vi "CAN Calibration Database Template.vi"() -> (0 "Calibration Template":string="<?xml version=\"1.0\" encoding=\"UTF-8\"?>\n<fx:FIBEX xmlns:fx=\"http://www.asam.net/xml/fbx\" xmlns:can=\"http://www.asam.net/xml/fbx/can\" xmlns:flexray=\"http://www.asam.net/xml/fbx/flexray\" xmlns:lin=\"http://www.asam.net/xml/fbx/lin\" xmlns:ho=\"http://www.asam.net/xml\" xmlns:ni=\"http://www.ni.com/xnet\" xmlns:xsi=\"http://www.w3.org/2001/XMLSchema-instance\" xsi:schemaLocation=\"http://www.asam.net/xml/fbx/all \\FIBEX311schema\\fibex4multiplatform.xsd\" VERSION=\"3.1.1\">\n  <fx:PROJECT ID=\"NI-XNET\">\n    <ho:SHORT-NAME>XNET1</ho:SHORT-NAME>\n  </fx:PROJECT>\n  <fx:ELEMENTS>\n    <fx:CLUSTERS>\n      <fx:CLUSTER ID=\"cluster1\">\n        <ho:SHORT-NAME>BS1200_Control_Bus</ho:SHORT-NAME>\n        <ho:DESC></ho:DESC>\n        <fx:SPEED>500000</fx:SPEED>\n        <fx:IS-HIGH-LOW-BIT-ORDER>true</fx:IS-HIGH-LOW-BIT-ORDER>\n        <fx:BIT-COUNTING-POLICY>SAWTOOTH</fx:BIT-COUNTING-POLICY>\n        <fx:PROTOCOL xsi:type=\"can:PROTOCOL-TYPE\">CAN</fx:PROTOCOL>\n        <fx:CHANNEL-REFS>\n          <fx:CHANNEL-REF ID-REF=\"channel1\"/>\n        </fx:CHANNEL-REFS>\n        <fx:MEDIUM>ELECTRICAL</fx:MEDIUM>\n      </fx:CLUSTER>\n    </fx:CLUSTERS>\n    <fx:CHANNELS>\n      <fx:CHANNEL ID=\"channel1\">\n        <ho:SHORT-NAME>Channel1</ho:SHORT-NAME>\n        <fx:PDU-TRIGGERINGS>\n        <fx:PDU-TRIGGERING ID=\"pdutrg1\">\n          <fx:TIMINGS>\n            <fx:CYCLIC-TIMING>\n              <fx:REPEATING-TIME-RANGE>\n                <fx:VALUE>PT0.01000000S</fx:VALUE>\n              </fx:REPEATING-TIME-RANGE>\n            </fx:CYCLIC-TIMING>\n          </fx:TIMINGS>\n          <fx:PDU-REF ID-REF=\"pdu1\"/>\n        </fx:PDU-TRIGGERING>\n        <fx:PDU-TRIGGERING ID=\"pdutrg2\">\n          <fx:TIMINGS>\n            <fx:EVENT-CONTROLLED-TIMING>\n              <fx:DEBOUNCE-TIME-RANGE>\n                <fx:VALUE>PT0.10000000S</fx:VALUE>\n              </fx:DEBOUNCE-TIME-RANGE>\n            </fx:EVENT-CONTROLLED-TIMING>\n          </fx:TIMINGS>\n          <fx:PDU-REF ID-REF=\"pdu10\"/>\n        </fx:PDU-TRIGGERING>\n        <fx:PDU-TRIGGERING ID=\"pdutrg3\">\n          <fx:TIMINGS>\n            <fx:EVENT-CONTROLLED-TIMING>\n              <fx:DEBOUNCE-TIME-RANGE>\n                <fx:VALUE>PT0.10000000S</fx:VALUE>\n              </fx:DEBOUNCE-TIME-RANGE>\n            </fx:EVENT-CONTROLLED-TIMING>\n          </fx:TIMINGS>\n          <fx:PDU-REF ID-REF=\"pdu11\"/>\n        </fx:PDU-TRIGGERING>\n        <fx:PDU-TRIGGERING ID=\"pdutrg4\">\n          <fx:TIMINGS>\n            <fx:CYCLIC-TIMING>\n              <fx:REPEATING-TIME-RANGE>\n                <fx:VALUE>PT0.01000000S</fx:VALUE>\n              </fx:REPEATING-TIME-RANGE>\n            </fx:CYCLIC-TIMING>\n          </fx:TIMINGS>\n          <fx:PDU-REF ID-REF=\"pdu12\"/>\n        </fx:PDU-TRIGGERING>\n        <fx:PDU-TRIGGERING ID=\"pdutrg5\">\n          <fx:TIMINGS>\n            <fx:CYCLIC-TIMING>\n              <fx:REPEATING-TIME-RANGE>\n                <fx:VALUE>PT0.01000000S</fx:VALUE>\n              </fx:REPEATING-TIME-RANGE>\n            </fx:CYCLIC-TIMING>\n          </fx:TIMINGS>\n          <fx:PDU-REF ID-REF=\"pdu13\"/>\n        </fx:PDU-TRIGGERING>\n        <fx:PDU-TRIGGERING ID=\"pdutrg6\">\n          <fx:TIMINGS>\n            <fx:CYCLIC-TIMING>\n              <fx:REPEATING-TIME-RANGE>\n                <fx:VALUE>PT0.01000000S</fx:VALUE>\n              </fx:REPEATING-TIME-RANGE>\n            </fx:CYCLIC-TIMING>\n          </fx:TIMINGS>\n          <fx:PDU-REF ID-REF=\"pdu14\"/>\n        </fx:PDU-TRIGGERING>\n        <fx:PDU-TRIGGERING ID=\"pdutrg7\">\n          <fx:TIMINGS>\n            <fx:EVENT-CONTROLLED-TIMING>\n              <fx:DEBOUNCE-TIME-RANGE>\n                <fx:VALUE>PT0.10000000S</fx:VALUE>\n              </fx:DEBOUNCE-TIME-RANGE>\n            </fx:EVENT-CONTROLLED-TIMING>\n          </fx:TIMINGS>\n          <fx:PDU-REF ID-REF=\"pdu15\"/>\n        </fx:PDU-TRIGGERING>\n        <fx:PDU-TRIGGERING ID=\"pdutrg8\">\n          <fx:TIMINGS>\n            <fx:EVENT-CONTROLLED-TIMING>\n              <fx:DEBOUNCE-TIME-RANGE>\n                <fx:VALUE>PT0.10000000S</fx:VALUE>\n              </fx:DEBOUNCE-TIME-RANGE>\n            </fx:EVENT-CONTROLLED-TIMING>\n          </fx:TIMINGS>\n          <fx:PDU-REF ID-REF=\"pdu16\"/>\n        </fx:PDU-TRIGGERING>\n        <fx:PDU-TRIGGERING ID=\"pdutrg9\">\n          <fx:TIMINGS>\n            <fx:EVENT-CONTROLLED-TIMING>\n              <fx:DEBOUNCE-TIME-RANGE>\n                <fx:VALUE>PT0.10000000S</fx:VALUE>\n              </fx:DEBOUNCE-TIME-RANGE>\n            </fx:EVENT-CONTROLLED-TIMING>\n          </fx:TIMINGS>\n          <fx:PDU-REF ID-REF=\"pdu17\"/>\n        </fx:PDU-TRIGGERING>\n        <fx:PDU-TRIGGERING ID=\"pdutrg10\">\n          <fx:TIMINGS>\n            <fx:EVENT-CONTROLLED-TIMING>\n              <fx:DEBOUNCE-TIME-RANGE>\n                <fx:VALUE>PT0.10000000S</fx:VALUE>\n              </fx:DEBOUNCE-TIME-RANGE>\n            </fx:EVENT-CONTROLLED-TIMING>\n          </fx:TIMINGS>\n          <fx:PDU-REF ID-REF=\"pdu18\"/>\n        </fx:PDU-TRIGGERING>\n        <fx:PDU-TRIGGERING ID=\"pdutrg11\">\n          <fx:TIMINGS>\n            <fx:EVENT-CONTROLLED-TIMING>\n              <fx:DEBOUNCE-TIME-RANGE>\n                <fx:VALUE>PT0.10000000S</fx:VALUE>\n              </fx:DEBOUNCE-TIME-RANGE>\n            </fx:EVENT-CONTROLLED-TIMING>\n          </fx:TIMINGS>\n          <fx:PDU-REF ID-REF=\"pdu19\"/>\n        </fx:PDU-TRIGGERING>\n        <fx:PDU-TRIGGERING ID=\"pdutrg12\">\n          <fx:TIMINGS>\n            <fx:CYCLIC-TIMING>\n              <fx:REPEATING-TIME-RANGE>\n                <fx:VALUE>PT0.01000000S</fx:VALUE>\n              </fx:REPEATING-TIME-RANGE>\n            </fx:CYCLIC-TIMING>\n          </fx:TIMINGS>\n          <fx:PDU-REF ID-REF=\"pdu2\"/>\n        </fx:PDU-TRIGGERING>\n        <fx:PDU-TRIGGERING ID=\"pdutrg13\">\n          <fx:TIMINGS>\n            <fx:EVENT-CONTROLLED-TIMING>\n              <fx:DEBOUNCE-TIME-RANGE>\n                <fx:VALUE>PT0.10000000S</fx:VALUE>\n              </fx:DEBOUNCE-TIME-RANGE>\n            </fx:EVENT-CONTROLLED-TIMING>\n          </fx:TIMINGS>\n          <fx:PDU-REF ID-REF=\"pdu20\"/>\n        </fx:PDU-TRIGGERING>\n        <fx:PDU-TRIGGERING ID=\"pdutrg14\">\n          <fx:TIMINGS>\n            <fx:CYCLIC-TIMING>\n              <fx:REPEATING-TIME-RANGE>\n                <fx:VALUE>PT0.01000000S</fx:VALUE>\n              </fx:REPEATING-TIME-RANGE>\n            </fx:CYCLIC-TIMING>\n          </fx:TIMINGS>\n          <fx:PDU-REF ID-REF=\"pdu21\"/>\n        </fx:PDU-TRIGGERING>\n        <fx:PDU-TRIGGERING ID=\"pdutrg15\">\n          <fx:TIMINGS>\n            <fx:EVENT-CONTROLLED-TIMING>\n              <fx:DEBOUNCE-TIME-RANGE>\n                <fx:VALUE>PT0.10000000S</fx:VALUE>\n              </fx:DEBOUNCE-TIME-RANGE>\n            </fx:EVENT-CONTROLLED-TIMING>\n          </fx:TIMINGS>\n          <fx:PDU-REF ID-REF=\"pdu22\"/>\n        </fx:PDU-TRIGGERING>\n        <fx:PDU-TRIGGERING ID=\"pdutrg16\">\n          <fx:TIMINGS>\n            <fx:EVENT-CONTROLLED-TIMING>\n              <fx:DEBOUNCE-TIME-RANGE>\n                <fx:VALUE>PT0.10000000S</fx:VALUE>\n              </fx:DEBOUNCE-TIME-RANGE>\n            </fx:EVENT-CONTROLLED-TIMING>\n          </fx:TIMINGS>\n          <fx:PDU-REF ID-REF=\"pdu23\"/>\n        </fx:PDU-TRIGGERING>\n        <fx:PDU-TRIGGERING ID=\"pdutrg17\">\n          <fx:TIMINGS>\n            <fx:CYCLIC-TIMING>\n              <fx:REPEATING-TIME-RANGE>\n                <fx:VALUE>PT1.000000S</fx:VALUE>\n              </fx:REPEATING-TIME-RANGE>\n            </fx:CYCLIC-TIMING>\n          </fx:TIMINGS>\n          <fx:PDU-REF ID-REF=\"pdu24\"/>\n        </fx:PDU-TRIGGERING>\n        <fx:PDU-TRIGGERING ID=\"pdutrg18\">\n          <fx:TIMINGS>\n            <fx:EVENT-CONTROLLED-TIMING>\n              <fx:DEBOUNCE-TIME-RANGE>\n                <fx:VALUE>PT0.10000000S</fx:VALUE>\n              </fx:DEBOUNCE-TIME-RANGE>\n            </fx:EVENT-CONTROLLED-TIMING>\n          </fx:TIMINGS>\n          <fx:PDU-REF ID-REF=\"pdu3\"/>\n        </fx:PDU-TRIGGERING>\n        <fx:PDU-TRIGGERING ID=\"pdutrg19\">\n          <fx:TIMINGS>\n            <fx:EVENT-CONTROLLED-TIMING>\n              <fx:DEBOUNCE-TIME-RANGE>\n                <fx:VALUE>PT0.10000000S</fx:VALUE>\n              </fx:DEBOUNCE-TIME-RANGE>\n            </fx:EVENT-CONTROLLED-TIMING>\n          </fx:TIMINGS>\n          <fx:PDU-REF ID-REF=\"pdu4\"/>\n        </fx:PDU-TRIGGERING>\n        <fx:PDU-TRIGGERING ID=\"pdutrg20\">\n          <fx:TIMINGS>\n            <fx:EVENT-CONTROLLED-TIMING>\n              <fx:DEBOUNCE-TIME-RANGE>\n                <fx:VALUE>PT0.10000000S</fx:VALUE>\n              </fx:DEBOUNCE-TIME-RANGE>\n            </fx:EVENT-CONTROLLED-TIMING>\n          </fx:TIMINGS>\n          <fx:PDU-REF ID-REF=\"pdu5\"/>\n        </fx:PDU-TRIGGERING>\n        <fx:PDU-TRIGGERING ID=\"pdutrg21\">\n          <fx:TIMINGS>\n            <fx:CYCLIC-TIMING>\n              <fx:REPEATING-TIME-RANGE>\n                <fx:VALUE>PT0.01000000S</fx:VALUE>\n              </fx:REPEATING-TIME-RANGE>\n            </fx:CYCLIC-TIMING>\n          </fx:TIMINGS>\n          <fx:PDU-REF ID-REF=\"pdu6\"/>\n        </fx:PDU-TRIGGERING>\n        <fx:PDU-TRIGGERING ID=\"pdutrg22\">\n          <fx:TIMINGS>\n            <fx:CYCLIC-TIMING>\n              <fx:REPEATING-TIME-RANGE>\n                <fx:VALUE>PT0.01000000S</fx:VALUE>\n              </fx:REPEATING-TIME-RANGE>\n            </fx:CYCLIC-TIMING>\n          </fx:TIMINGS>\n          <fx:PDU-REF ID-REF=\"pdu7\"/>\n        </fx:PDU-TRIGGERING>\n        <fx:PDU-TRIGGERING ID=\"pdutrg23\">\n          <fx:TIMINGS>\n            <fx:CYCLIC-TIMING>\n              <fx:REPEATING-TIME-RANGE>\n                <fx:VALUE>PT0.01000000S</fx:VALUE>\n              </fx:REPEATING-TIME-RANGE>\n            </fx:CYCLIC-TIMING>\n          </fx:TIMINGS>\n          <fx:PDU-REF ID-REF=\"pdu8\"/>\n        </fx:PDU-TRIGGERING>\n        <fx:PDU-TRIGGERING ID=\"pdutrg24\">\n          <fx:TIMINGS>\n            <fx:EVENT-CONTROLLED-TIMING>\n              <fx:DEBOUNCE-TIME-RANGE>\n                <fx:VALUE>PT0.10000000S</fx:VALUE>\n              </fx:DEBOUNCE-TIME-RANGE>\n            </fx:EVENT-CONTROLLED-TIMING>\n          </fx:TIMINGS>\n          <fx:PDU-REF ID-REF=\"pdu9\"/>\n        </fx:PDU-TRIGGERING>\n        </fx:PDU-TRIGGERINGS>\n        <fx:FRAME-TRIGGERINGS>\n          <fx:FRAME-TRIGGERING ID=\"trig1\">\n            <fx:IDENTIFIER>\n              <fx:IDENTIFIER-VALUE>128</fx:IDENTIFIER-VALUE>\n            </fx:IDENTIFIER>\n            <fx:FRAME-REF ID-REF=\"frm1\"/>\n          </fx:FRAME-TRIGGERING>\n          <fx:FRAME-TRIGGERING ID=\"trig2\">\n            <fx:IDENTIFIER>\n              <fx:IDENTIFIER-VALUE>192</fx:IDENTIFIER-VALUE>\n            </fx:IDENTIFIER>\n            <fx:FRAME-REF ID-REF=\"frm2\"/>\n          </fx:FRAME-TRIGGERING>\n          <fx:FRAME-TRIGGERING ID=\"trig3\">\n            <fx:IDENTIFIER>\n              <fx:IDENTIFIER-VALUE>1200</fx:IDENTIFIER-VALUE>\n            </fx:IDENTIFIER>\n            <fx:FRAME-REF ID-REF=\"frm3\"/>\n          </fx:FRAME-TRIGGERING>\n          <fx:FRAME-TRIGGERING ID=\"trig4\">\n            <fx:IDENTIFIER>\n              <fx:IDENTIFIER-VALUE>1280</fx:IDENTIFIER-VALUE>\n            </fx:IDENTIFIER>\n            <fx:FRAME-REF ID-REF=\"frm4\"/>\n          </fx:FRAME-TRIGGERING>\n          <fx:FRAME-TRIGGERING ID=\"trig5\">\n            <fx:IDENTIFIER>\n              <fx:IDENTIFIER-VALUE>512</fx:IDENTIFIER-VALUE>\n            </fx:IDENTIFIER>\n            <fx:FRAME-REF ID-REF=\"frm5\"/>\n          </fx:FRAME-TRIGGERING>\n          <fx:FRAME-TRIGGERING ID=\"trig6\">\n            <fx:IDENTIFIER>\n              <fx:IDENTIFIER-VALUE>544</fx:IDENTIFIER-VALUE>\n            </fx:IDENTIFIER>\n            <fx:FRAME-REF ID-REF=\"frm6\"/>\n          </fx:FRAME-TRIGGERING>\n          <fx:FRAME-TRIGGERING ID=\"trig7\">\n            <fx:IDENTIFIER>\n              <fx:IDENTIFIER-VALUE>1024</fx:IDENTIFIER-VALUE>\n            </fx:IDENTIFIER>\n            <fx:FRAME-REF ID-REF=\"frm7\"/>\n          </fx:FRAME-TRIGGERING>\n          <fx:FRAME-TRIGGERING ID=\"trig8\">\n            <fx:IDENTIFIER>\n              <fx:IDENTIFIER-VALUE>1152</fx:IDENTIFIER-VALUE>\n            </fx:IDENTIFIER>\n            <fx:FRAME-REF ID-REF=\"frm8\"/>\n          </fx:FRAME-TRIGGERING>\n          <fx:FRAME-TRIGGERING ID=\"trig9\">\n            <fx:IDENTIFIER>\n              <fx:IDENTIFIER-VALUE>1184</fx:IDENTIFIER-VALUE>\n            </fx:IDENTIFIER>\n            <fx:FRAME-REF ID-REF=\"frm9\"/>\n          </fx:FRAME-TRIGGERING>\n          <fx:FRAME-TRIGGERING ID=\"trig10\">\n            <fx:IDENTIFIER>\n              <fx:IDENTIFIER-VALUE>1296</fx:IDENTIFIER-VALUE>\n            </fx:IDENTIFIER>\n            <fx:FRAME-REF ID-REF=\"frm10\"/>\n          </fx:FRAME-TRIGGERING>\n          <fx:FRAME-TRIGGERING ID=\"trig11\">\n            <fx:IDENTIFIER>\n              <fx:IDENTIFIER-VALUE>320</fx:IDENTIFIER-VALUE>\n            </fx:IDENTIFIER>\n            <fx:FRAME-REF ID-REF=\"frm11\"/>\n          </fx:FRAME-TRIGGERING>\n          <fx:FRAME-TRIGGERING ID=\"trig12\">\n            <fx:IDENTIFIER>\n              <fx:IDENTIFIER-VALUE>384</fx:IDENTIFIER-VALUE>\n            </fx:IDENTIFIER>\n            <fx:FRAME-REF ID-REF=\"frm12\"/>\n          </fx:FRAME-TRIGGERING>\n          <fx:FRAME-TRIGGERING ID=\"trig13\">\n            <fx:IDENTIFIER>\n              <fx:IDENTIFIER-VALUE>1344</fx:IDENTIFIER-VALUE>\n            </fx:IDENTIFIER>\n            <fx:FRAME-REF ID-REF=\"frm13\"/>\n          </fx:FRAME-TRIGGERING>\n          <fx:FRAME-TRIGGERING ID=\"trig14\">\n            <fx:IDENTIFIER>\n              <fx:IDENTIFIER-VALUE>1360</fx:IDENTIFIER-VALUE>\n            </fx:IDENTIFIER>\n            <fx:FRAME-REF ID-REF=\"frm14\"/>\n          </fx:FRAME-TRIGGERING>\n          <fx:FRAME-TRIGGERING ID=\"trig15\">\n            <fx:IDENTIFIER>\n              <fx:IDENTIFIER-VALUE>256</fx:IDENTIFIER-VALUE>\n            </fx:IDENTIFIER>\n            <fx:FRAME-REF ID-REF=\"frm15\"/>\n            <fx:MANUFACTURER-EXTENSION>\n              <ni:NI-XNET-EXTENSION>\n                <ni:CAN-FD-MODE>0</ni:CAN-FD-MODE>\n              </ni:NI-XNET-EXTENSION>\n            </fx:MANUFACTURER-EXTENSION>\n          </fx:FRAME-TRIGGERING>\n          <fx:FRAME-TRIGGERING ID=\"trig16\">\n            <fx:IDENTIFIER>\n              <fx:IDENTIFIER-VALUE>288</fx:IDENTIFIER-VALUE>\n            </fx:IDENTIFIER>\n            <fx:FRAME-REF ID-REF=\"frm16\"/>\n          </fx:FRAME-TRIGGERING>\n          <fx:FRAME-TRIGGERING ID=\"trig17\">\n            <fx:IDENTIFIER>\n              <fx:IDENTIFIER-VALUE>304</fx:IDENTIFIER-VALUE>\n            </fx:IDENTIFIER>\n            <fx:FRAME-REF ID-REF=\"frm17\"/>\n          </fx:FRAME-TRIGGERING>\n          <fx:FRAME-TRIGGERING ID=\"trig18\">\n            <fx:IDENTIFIER>\n              <fx:IDENTIFIER-VALUE>160</fx:IDENTIFIER-VALUE>\n            </fx:IDENTIFIER>\n            <fx:FRAME-REF ID-REF=\"frm18\"/>\n          </fx:FRAME-TRIGGERING>\n          <fx:FRAME-TRIGGERING ID=\"trig19\">\n            <fx:IDENTIFIER>\n              <fx:IDENTIFIER-VALUE>176</fx:IDENTIFIER-VALUE>\n            </fx:IDENTIFIER>\n            <fx:FRAME-REF ID-REF=\"frm19\"/>\n          </fx:FRAME-TRIGGERING>\n          <fx:FRAME-TRIGGERING ID=\"trig20\">\n            <fx:IDENTIFIER>\n              <fx:IDENTIFIER-VALUE>400</fx:IDENTIFIER-VALUE>\n            </fx:IDENTIFIER>\n            <fx:FRAME-REF ID-REF=\"frm20\"/>\n          </fx:FRAME-TRIGGERING>\n          <fx:FRAME-TRIGGERING ID=\"trig21\">\n            <fx:IDENTIFIER>\n              <fx:IDENTIFIER-VALUE>416</fx:IDENTIFIER-VALUE>\n            </fx:IDENTIFIER>\n            <fx:FRAME-REF ID-REF=\"frm21\"/>\n          </fx:FRAME-TRIGGERING>\n          <fx:FRAME-TRIGGERING ID=\"trig22\">\n            <fx:IDENTIFIER>\n              <fx:IDENTIFIER-VALUE>640</fx:IDENTIFIER-VALUE>\n            </fx:IDENTIFIER>\n            <fx:FRAME-REF ID-REF=\"frm22\"/>\n            <fx:MANUFACTURER-EXTENSION>\n              <ni:NI-XNET-EXTENSION>\n                <ni:CAN-FD-MODE>0</ni:CAN-FD-MODE>\n              </ni:NI-XNET-EXTENSION>\n            </fx:MANUFACTURER-EXTENSION>\n          </fx:FRAME-TRIGGERING>\n          <fx:FRAME-TRIGGERING ID=\"trig23\">\n            <fx:IDENTIFIER>\n              <fx:IDENTIFIER-VALUE>672</fx:IDENTIFIER-VALUE>\n            </fx:IDENTIFIER>\n            <fx:FRAME-REF ID-REF=\"frm23\"/>\n          </fx:FRAME-TRIGGERING>\n          <fx:FRAME-TRIGGERING ID=\"trig24\">\n            <fx:IDENTIFIER>\n              <fx:IDENTIFIER-VALUE>688</fx:IDENTIFIER-VALUE>\n            </fx:IDENTIFIER>\n            <fx:FRAME-REF ID-REF=\"frm24\"/>\n          </fx:FRAME-TRIGGERING>\n        </fx:FRAME-TRIGGERINGS>\n      </fx:CHANNEL>\n    </fx:CHANNELS>\n    <fx:PDUS>\n      <fx:PDU ID=\"pdu1\">\n        <ho:SHORT-NAME>AI_Readback_1_4_pdu</ho:SHORT-NAME>\n        <ho:DESC></ho:DESC>\n        <fx:BYTE-LENGTH>8</fx:BYTE-LENGTH>\n        <fx:PDU-TYPE>APPLICATION</fx:PDU-TYPE>\n        <fx:SIGNAL-INSTANCES>\n          <fx:SIGNAL-INSTANCE ID=\"sgi1\">\n            <fx:BIT-POSITION>0</fx:BIT-POSITION>\n            <fx:IS-HIGH-LOW-BYTE-ORDER>false</fx:IS-HIGH-LOW-BYTE-ORDER>\n            <fx:SIGNAL-REF ID-REF=\"sig68\"/>\n          </fx:SIGNAL-INSTANCE>\n          <fx:SIGNAL-INSTANCE ID=\"sgi2\">\n            <fx:BIT-POSITION>16</fx:BIT-POSITION>\n            <fx:IS-HIGH-LOW-BYTE-ORDER>false</fx:IS-HIGH-LOW-BYTE-ORDER>\n            <fx:SIGNAL-REF ID-REF=\"sig69\"/>\n          </fx:SIGNAL-INSTANCE>\n          <fx:SIGNAL-INSTANCE ID=\"sgi3\">\n            <fx:BIT-POSITION>32</fx:BIT-POSITION>\n            <fx:IS-HIGH-LOW-BYTE-ORDER>false</fx:IS-HIGH-LOW-BYTE-ORDER>\n            <fx:SIGNAL-REF ID-REF=\"sig70\"/>\n          </fx:SIGNAL-INSTANCE>\n          <fx:SIGNAL-INSTANCE ID=\"sgi4\">\n            <fx:BIT-POSITION>48</fx:BIT-POSITION>\n            <fx:IS-HIGH-LOW-BYTE-ORDER>false</fx:IS-HIGH-LOW-BYTE-ORDER>\n            <fx:SIGNAL-REF ID-REF=\"sig71\"/>\n          </fx:SIGNAL-INSTANCE>\n        </fx:SIGNAL-INSTANCES>\n      </fx:PDU>\n      <fx:PDU ID=\"pdu2\">\n        <ho:SHORT-NAME>AI_Readback_5_8_pdu</ho:SHORT-NAME>\n        <ho:DESC></ho:DESC>\n        <fx:BYTE-LENGTH>8</fx:BYTE-LENGTH>\n        <fx:PDU-TYPE>APPLICATION</fx:PDU-TYPE>\n        <fx:SIGNAL-INSTANCES>\n          <fx:SIGNAL-INSTANCE ID=\"sgi5\">\n            <fx:BIT-POSITION>0</fx:BIT-POSITION>\n            <fx:IS-HIGH-LOW-BYTE-ORDER>false</fx:IS-HIGH-LOW-BYTE-ORDER>\n            <fx:SIGNAL-REF ID-REF=\"sig72\"/>\n          </fx:SIGNAL-INSTANCE>\n          <fx:SIGNAL-INSTANCE ID=\"sgi6\">\n            <fx:BIT-POSITION>16</fx:BIT-POSITION>\n            <fx:IS-HIGH-LOW-BYTE-ORDER>false</fx:IS-HIGH-LOW-BYTE-ORDER>\n            <fx:SIGNAL-REF ID-REF=\"sig73\"/>\n          </fx:SIGNAL-INSTANCE>\n          <fx:SIGNAL-INSTANCE ID=\"sgi7\">\n            <fx:BIT-POSITION>32</fx:BIT-POSITION>\n            <fx:IS-HIGH-LOW-BYTE-ORDER>false</fx:IS-HIGH-LOW-BYTE-ORDER>\n            <fx:SIGNAL-REF ID-REF=\"sig74\"/>\n          </fx:SIGNAL-INSTANCE>\n          <fx:SIGNAL-INSTANCE ID=\"sgi8\">\n            <fx:BIT-POSITION>48</fx:BIT-POSITION>\n            <fx:IS-HIGH-LOW-BYTE-ORDER>false</fx:IS-HIGH-LOW-BYTE-ORDER>\n            <fx:SIGNAL-REF ID-REF=\"sig75\"/>\n          </fx:SIGNAL-INSTANCE>\n        </fx:SIGNAL-INSTANCES>\n      </fx:PDU>\n      <fx:PDU ID=\"pdu3\">\n        <ho:SHORT-NAME>Analog_Out_Set_1_2_pdu</ho:SHORT-NAME>\n        <ho:DESC></ho:DESC>\n        <fx:BYTE-LENGTH>8</fx:BYTE-LENGTH>\n        <fx:PDU-TYPE>APPLICATION</fx:PDU-TYPE>\n        <fx:SIGNAL-INSTANCES>\n          <fx:SIGNAL-INSTANCE ID=\"sgi9\">\n            <fx:BIT-POSITION>0</fx:BIT-POSITION>\n            <fx:IS-HIGH-LOW-BYTE-ORDER>false</fx:IS-HIGH-LOW-BYTE-ORDER>\n            <fx:SIGNAL-REF ID-REF=\"sig11\"/>\n          </fx:SIGNAL-INSTANCE>\n          <fx:SIGNAL-INSTANCE ID=\"sgi10\">\n            <fx:BIT-POSITION>16</fx:BIT-POSITION>\n            <fx:IS-HIGH-LOW-BYTE-ORDER>false</fx:IS-HIGH-LOW-BYTE-ORDER>\n            <fx:SIGNAL-REF ID-REF=\"sig12\"/>\n          </fx:SIGNAL-INSTANCE>\n        </fx:SIGNAL-INSTANCES>\n      </fx:PDU>\n      <fx:PDU ID=\"pdu4\">\n        <ho:SHORT-NAME>Cell_Enable_All_pdu</ho:SHORT-NAME>\n        <ho:DESC></ho:DESC>\n        <fx:BYTE-LENGTH>1</fx:BYTE-LENGTH>\n        <fx:PDU-TYPE>APPLICATION</fx:PDU-TYPE>\n        <fx:SIGNAL-INSTANCES>\n          <fx:SIGNAL-INSTANCE ID=\"sgi11\">\n            <fx:BIT-POSITION>0</fx:BIT-POSITION>\n            <fx:IS-HIGH-LOW-BYTE-ORDER>false</fx:IS-HIGH-LOW-BYTE-ORDER>\n            <fx:SIGNAL-REF ID-REF=\"sig33\"/>\n          </fx:SIGNAL-INSTANCE>\n        </fx:SIGNAL-INSTANCES>\n      </fx:PDU>\n      <fx:PDU ID=\"pdu5\">\n        <ho:SHORT-NAME>Cell_Enable_pdu</ho:SHORT-NAME>\n        <ho:DESC></ho:DESC>\n        <fx:BYTE-LENGTH>2</fx:BYTE-LENGTH>\n        <fx:PDU-TYPE>APPLICATION</fx:PDU-TYPE>\n        <fx:SIGNAL-INSTANCES>\n          <fx:SIGNAL-INSTANCE ID=\"sgi12\">\n            <fx:BIT-POSITION>0</fx:BIT-POSITION>\n            <fx:IS-HIGH-LOW-BYTE-ORDER>false</fx:IS-HIGH-LOW-BYTE-ORDER>\n            <fx:SIGNAL-REF ID-REF=\"sig34\"/>\n          </fx:SIGNAL-INSTANCE>\n          <fx:SIGNAL-INSTANCE ID=\"sgi13\">\n            <fx:BIT-POSITION>8</fx:BIT-POSITION>\n            <fx:IS-HIGH-LOW-BYTE-ORDER>false</fx:IS-HIGH-LOW-BYTE-ORDER>\n            <fx:SIGNAL-REF ID-REF=\"sig35\"/>\n          </fx:SIGNAL-INSTANCE>\n        </fx:SIGNAL-INSTANCES>\n      </fx:PDU>\n      <fx:PDU ID=\"pdu6\">\n        <ho:SHORT-NAME>Cell_I_Readback_1_4_pdu</ho:SHORT-NAME>\n        <ho:DESC></ho:DESC>\n        <fx:BYTE-LENGTH>8</fx:BYTE-LENGTH>\n        <fx:PDU-TYPE>APPLICATION</fx:PDU-TYPE>\n        <fx:SIGNAL-INSTANCES>\n          <fx:SIGNAL-INSTANCE ID=\"sgi14\">\n            <fx:BIT-POSITION>0</fx:BIT-POSITION>\n            <fx:IS-HIGH-LOW-BYTE-ORDER>false</fx:IS-HIGH-LOW-BYTE-ORDER>\n            <fx:SIGNAL-REF ID-REF=\"sig29\"/>\n          </fx:SIGNAL-INSTANCE>\n          <fx:SIGNAL-INSTANCE ID=\"sgi15\">\n            <fx:BIT-POSITION>16</fx:BIT-POSITION>\n            <fx:IS-HIGH-LOW-BYTE-ORDER>false</fx:IS-HIGH-LOW-BYTE-ORDER>\n            <fx:SIGNAL-REF ID-REF=\"sig30\"/>\n          </fx:SIGNAL-INSTANCE>\n          <fx:SIGNAL-INSTANCE ID=\"sgi16\">\n            <fx:BIT-POSITION>32</fx:BIT-POSITION>\n            <fx:IS-HIGH-LOW-BYTE-ORDER>false</fx:IS-HIGH-LOW-BYTE-ORDER>\n            <fx:SIGNAL-REF ID-REF=\"sig31\"/>\n          </fx:SIGNAL-INSTANCE>\n          <fx:SIGNAL-INSTANCE ID=\"sgi17\">\n            <fx:BIT-POSITION>48</fx:BIT-POSITION>\n            <fx:IS-HIGH-LOW-BYTE-ORDER>false</fx:IS-HIGH-LOW-BYTE-ORDER>\n            <fx:SIGNAL-REF ID-REF=\"sig32\"/>\n          </fx:SIGNAL-INSTANCE>\n        </fx:SIGNAL-INSTANCES>\n      </fx:PDU>\n      <fx:PDU ID=\"pdu7\">\n        <ho:SHORT-NAME>Cell_I_Readback_5_8_pdu</ho:SHORT-NAME>\n        <ho:DESC></ho:DESC>\n        <fx:BYTE-LENGTH>8</fx:BYTE-LENGTH>\n        <fx:PDU-TYPE>APPLICATION</fx:PDU-TYPE>\n        <fx:SIGNAL-INSTANCES>\n          <fx:SIGNAL-INSTANCE ID=\"sgi18\">\n            <fx:BIT-POSITION>0</fx:BIT-POSITION>\n            <fx:IS-HIGH-LOW-BYTE-ORDER>false</fx:IS-HIGH-LOW-BYTE-ORDER>\n            <fx:SIGNAL-REF ID-REF=\"sig59\"/>\n          </fx:SIGNAL-INSTANCE>\n          <fx:SIGNAL-INSTANCE ID=\"sgi19\">\n            <fx:BIT-POSITION>16</fx:BIT-POSITION>\n            <fx:IS-HIGH-LOW-BYTE-ORDER>false</fx:IS-HIGH-LOW-BYTE-ORDER>\n            <fx:SIGNAL-REF ID-REF=\"sig60\"/>\n          </fx:SIGNAL-INSTANCE>\n          <fx:SIGNAL-INSTANCE ID=\"sgi20\">\n            <fx:BIT-POSITION>32</fx:BIT-POSITION>\n            <fx:IS-HIGH-LOW-BYTE-ORDER>false</fx:IS-HIGH-LOW-BYTE-ORDER>\n            <fx:SIGNAL-REF ID-REF=\"sig61\"/>\n          </fx:SIGNAL-INSTANCE>\n          <fx:SIGNAL-INSTANCE ID=\"sgi21\">\n            <fx:BIT-POSITION>48</fx:BIT-POSITION>\n            <fx:IS-HIGH-LOW-BYTE-ORDER>false</fx:IS-HIGH-LOW-BYTE-ORDER>\n            <fx:SIGNAL-REF ID-REF=\"sig62\"/>\n          </fx:SIGNAL-INSTANCE>\n        </fx:SIGNAL-INSTANCES>\n      </fx:PDU>\n      <fx:PDU ID=\"pdu8\">\n        <ho:SHORT-NAME>Cell_I_Readback_9_12_pdu</ho:SHORT-NAME>\n        <ho:DESC></ho:DESC>\n        <fx:BYTE-LENGTH>8</fx:BYTE-LENGTH>\n        <fx:PDU-TYPE>APPLICATION</fx:PDU-TYPE>\n        <fx:SIGNAL-INSTANCES>\n          <fx:SIGNAL-INSTANCE ID=\"sgi22\">\n            <fx:BIT-POSITION>0</fx:BIT-POSITION>\n            <fx:IS-HIGH-LOW-BYTE-ORDER>false</fx:IS-HIGH-LOW-BYTE-ORDER>\n            <fx:SIGNAL-REF ID-REF=\"sig63\"/>\n          </fx:SIGNAL-INSTANCE>\n          <fx:SIGNAL-INSTANCE ID=\"sgi23\">\n            <fx:BIT-POSITION>16</fx:BIT-POSITION>\n            <fx:IS-HIGH-LOW-BYTE-ORDER>false</fx:IS-HIGH-LOW-BYTE-ORDER>\n            <fx:SIGNAL-REF ID-REF=\"sig64\"/>\n          </fx:SIGNAL-INSTANCE>\n          <fx:SIGNAL-INSTANCE ID=\"sgi24\">\n            <fx:BIT-POSITION>32</fx:BIT-POSITION>\n            <fx:IS-HIGH-LOW-BYTE-ORDER>false</fx:IS-HIGH-LOW-BYTE-ORDER>\n            <fx:SIGNAL-REF ID-REF=\"sig65\"/>\n          </fx:SIGNAL-INSTANCE>\n          <fx:SIGNAL-INSTANCE ID=\"sgi25\">\n            <fx:BIT-POSITION>48</fx:BIT-POSITION>\n            <fx:IS-HIGH-LOW-BYTE-ORDER>false</fx:IS-HIGH-LOW-BYTE-ORDER>\n            <fx:SIGNAL-REF ID-REF=\"sig66\"/>\n          </fx:SIGNAL-INSTANCE>\n        </fx:SIGNAL-INSTANCES>\n      </fx:PDU>\n      <fx:PDU ID=\"pdu9\">\n        <ho:SHORT-NAME>Cell_I_Set_All_pdu</ho:SHORT-NAME>\n        <ho:DESC></ho:DESC>\n        <fx:BYTE-LENGTH>4</fx:BYTE-LENGTH>\n        <fx:PDU-TYPE>APPLICATION</fx:PDU-TYPE>\n        <fx:SIGNAL-INSTANCES>\n          <fx:SIGNAL-INSTANCE ID=\"sgi26\">\n            <fx:BIT-POSITION>0</fx:BIT-POSITION>\n            <fx:IS-HIGH-LOW-BYTE-ORDER>false</fx:IS-HIGH-LOW-BYTE-ORDER>\n            <fx:SIGNAL-REF ID-REF=\"sig19\"/>\n          </fx:SIGNAL-INSTANCE>\n          <fx:SIGNAL-INSTANCE ID=\"sgi27\">\n            <fx:BIT-POSITION>16</fx:BIT-POSITION>\n            <fx:IS-HIGH-LOW-BYTE-ORDER>false</fx:IS-HIGH-LOW-BYTE-ORDER>\n            <fx:SIGNAL-REF ID-REF=\"sig20\"/>\n          </fx:SIGNAL-INSTANCE>\n        </fx:SIGNAL-INSTANCES>\n      </fx:PDU>\n      <fx:PDU ID=\"pdu10\">\n        <ho:SHORT-NAME>Cell_I_Sink_Set_pdu</ho:SHORT-NAME>\n        <ho:DESC></ho:DESC>\n        <fx:BYTE-LENGTH>3</fx:BYTE-LENGTH>\n        <fx:PDU-TYPE>APPLICATION</fx:PDU-TYPE>\n        <fx:SIGNAL-INSTANCES>\n          <fx:SIGNAL-INSTANCE ID=\"sgi28\">\n            <fx:BIT-POSITION>0</fx:BIT-POSITION>\n            <fx:IS-HIGH-LOW-BYTE-ORDER>false</fx:IS-HIGH-LOW-BYTE-ORDER>\n            <fx:SIGNAL-REF ID-REF=\"sig21\"/>\n          </fx:SIGNAL-INSTANCE>\n          <fx:SIGNAL-INSTANCE ID=\"sgi29\">\n            <fx:BIT-POSITION>8</fx:BIT-POSITION>\n            <fx:IS-HIGH-LOW-BYTE-ORDER>false</fx:IS-HIGH-LOW-BYTE-ORDER>\n            <fx:SIGNAL-REF ID-REF=\"sig22\"/>\n          </fx:SIGNAL-INSTANCE>\n        </fx:SIGNAL-INSTANCES>\n      </fx:PDU>\n      <fx:PDU ID=\"pdu11\">\n        <ho:SHORT-NAME>Cell_I_Source_Set_pdu</ho:SHORT-NAME>\n        <ho:DESC></ho:DESC>\n        <fx:BYTE-LENGTH>3</fx:BYTE-LENGTH>\n        <fx:PDU-TYPE>APPLICATION</fx:PDU-TYPE>\n        <fx:SIGNAL-INSTANCES>\n          <fx:SIGNAL-INSTANCE ID=\"sgi30\">\n            <fx:BIT-POSITION>0</fx:BIT-POSITION>\n            <fx:IS-HIGH-LOW-BYTE-ORDER>false</fx:IS-HIGH-LOW-BYTE-ORDER>\n            <fx:SIGNAL-REF ID-REF=\"sig6\"/>\n          </fx:SIGNAL-INSTANCE>\n          <fx:SIGNAL-INSTANCE ID=\"sgi31\">\n            <fx:BIT-POSITION>8</fx:BIT-POSITION>\n            <fx:IS-HIGH-LOW-BYTE-ORDER>false</fx:IS-HIGH-LOW-BYTE-ORDER>\n            <fx:SIGNAL-REF ID-REF=\"sig7\"/>\n          </fx:SIGNAL-INSTANCE>\n        </fx:SIGNAL-INSTANCES>\n      </fx:PDU>\n      <fx:PDU ID=\"pdu12\">\n        <ho:SHORT-NAME>Cell_V_Readback_1_4_pdu</ho:SHORT-NAME>\n        <ho:DESC></ho:DESC>\n        <fx:BYTE-LENGTH>8</fx:BYTE-LENGTH>\n        <fx:PDU-TYPE>APPLICATION</fx:PDU-TYPE>\n        <fx:SIGNAL-INSTANCES>\n          <fx:SIGNAL-INSTANCE ID=\"sgi32\">\n            <fx:BIT-POSITION>0</fx:BIT-POSITION>\n            <fx:IS-HIGH-LOW-BYTE-ORDER>false</fx:IS-HIGH-LOW-BYTE-ORDER>\n            <fx:SIGNAL-REF ID-REF=\"sig43\"/>\n          </fx:SIGNAL-INSTANCE>\n          <fx:SIGNAL-INSTANCE ID=\"sgi33\">\n            <fx:BIT-POSITION>16</fx:BIT-POSITION>\n            <fx:IS-HIGH-LOW-BYTE-ORDER>false</fx:IS-HIGH-LOW-BYTE-ORDER>\n            <fx:SIGNAL-REF ID-REF=\"sig44\"/>\n          </fx:SIGNAL-INSTANCE>\n          <fx:SIGNAL-INSTANCE ID=\"sgi34\">\n            <fx:BIT-POSITION>32</fx:BIT-POSITION>\n            <fx:IS-HIGH-LOW-BYTE-ORDER>false</fx:IS-HIGH-LOW-BYTE-ORDER>\n            <fx:SIGNAL-REF ID-REF=\"sig45\"/>\n          </fx:SIGNAL-INSTANCE>\n          <fx:SIGNAL-INSTANCE ID=\"sgi35\">\n            <fx:BIT-POSITION>48</fx:BIT-POSITION>\n            <fx:IS-HIGH-LOW-BYTE-ORDER>false</fx:IS-HIGH-LOW-BYTE-ORDER>\n            <fx:SIGNAL-REF ID-REF=\"sig46\"/>\n          </fx:SIGNAL-INSTANCE>\n        </fx:SIGNAL-INSTANCES>\n      </fx:PDU>\n      <fx:PDU ID=\"pdu13\">\n        <ho:SHORT-NAME>Cell_V_Readback_5_8_pdu</ho:SHORT-NAME>\n        <ho:DESC></ho:DESC>\n        <fx:BYTE-LENGTH>8</fx:BYTE-LENGTH>\n        <fx:PDU-TYPE>APPLICATION</fx:PDU-TYPE>\n        <fx:SIGNAL-INSTANCES>\n          <fx:SIGNAL-INSTANCE ID=\"sgi36\">\n            <fx:BIT-POSITION>0</fx:BIT-POSITION>\n            <fx:IS-HIGH-LOW-BYTE-ORDER>false</fx:IS-HIGH-LOW-BYTE-ORDER>\n            <fx:SIGNAL-REF ID-REF=\"sig47\"/>\n          </fx:SIGNAL-INSTANCE>\n          <fx:SIGNAL-INSTANCE ID=\"sgi37\">\n            <fx:BIT-POSITION>16</fx:BIT-POSITION>\n            <fx:IS-HIGH-LOW-BYTE-ORDER>false</fx:IS-HIGH-LOW-BYTE-ORDER>\n            <fx:SIGNAL-REF ID-REF=\"sig48\"/>\n          </fx:SIGNAL-INSTANCE>\n          <fx:SIGNAL-INSTANCE ID=\"sgi38\">\n            <fx:BIT-POSITION>32</fx:BIT-POSITION>\n            <fx:IS-HIGH-LOW-BYTE-ORDER>false</fx:IS-HIGH-LOW-BYTE-ORDER>\n            <fx:SIGNAL-REF ID-REF=\"sig49\"/>\n          </fx:SIGNAL-INSTANCE>\n          <fx:SIGNAL-INSTANCE ID=\"sgi39\">\n            <fx:BIT-POSITION>48</fx:BIT-POSITION>\n            <fx:IS-HIGH-LOW-BYTE-ORDER>false</fx:IS-HIGH-LOW-BYTE-ORDER>\n            <fx:SIGNAL-REF ID-REF=\"sig50\"/>\n          </fx:SIGNAL-INSTANCE>\n        </fx:SIGNAL-INSTANCES>\n      </fx:PDU>\n      <fx:PDU ID=\"pdu14\">\n        <ho:SHORT-NAME>Cell_V_Readback_9_12_pdu</ho:SHORT-NAME>\n        <ho:DESC></ho:DESC>\n        <fx:BYTE-LENGTH>8</fx:BYTE-LENGTH>\n        <fx:PDU-TYPE>APPLICATION</fx:PDU-TYPE>\n        <fx:SIGNAL-INSTANCES>\n          <fx:SIGNAL-INSTANCE ID=\"sgi40\">\n            <fx:BIT-POSITION>0</fx:BIT-POSITION>\n            <fx:IS-HIGH-LOW-BYTE-ORDER>false</fx:IS-HIGH-LOW-BYTE-ORDER>\n            <fx:SIGNAL-REF ID-REF=\"sig25\"/>\n          </fx:SIGNAL-INSTANCE>\n          <fx:SIGNAL-INSTANCE ID=\"sgi41\">\n            <fx:BIT-POSITION>16</fx:BIT-POSITION>\n            <fx:IS-HIGH-LOW-BYTE-ORDER>false</fx:IS-HIGH-LOW-BYTE-ORDER>\n            <fx:SIGNAL-REF ID-REF=\"sig26\"/>\n          </fx:SIGNAL-INSTANCE>\n          <fx:SIGNAL-INSTANCE ID=\"sgi42\">\n            <fx:BIT-POSITION>32</fx:BIT-POSITION>\n            <fx:IS-HIGH-LOW-BYTE-ORDER>false</fx:IS-HIGH-LOW-BYTE-ORDER>\n            <fx:SIGNAL-REF ID-REF=\"sig27\"/>\n          </fx:SIGNAL-INSTANCE>\n          <fx:SIGNAL-INSTANCE ID=\"sgi43\">\n            <fx:BIT-POSITION>48</fx:BIT-POSITION>\n            <fx:IS-HIGH-LOW-BYTE-ORDER>false</fx:IS-HIGH-LOW-BYTE-ORDER>\n            <fx:SIGNAL-REF ID-REF=\"sig28\"/>\n          </fx:SIGNAL-INSTANCE>\n        </fx:SIGNAL-INSTANCES>\n      </fx:PDU>\n      <fx:PDU ID=\"pdu15\">\n        <ho:SHORT-NAME>Cell_V_Set_1_4_pdu</ho:SHORT-NAME>\n        <ho:DESC></ho:DESC>\n        <fx:BYTE-LENGTH>8</fx:BYTE-LENGTH>\n        <fx:PDU-TYPE>APPLICATION</fx:PDU-TYPE>\n        <fx:SIGNAL-INSTANCES>\n          <fx:SIGNAL-INSTANCE ID=\"sgi44\">\n            <fx:BIT-POSITION>0</fx:BIT-POSITION>\n            <fx:IS-HIGH-LOW-BYTE-ORDER>false</fx:IS-HIGH-LOW-BYTE-ORDER>\n            <fx:SIGNAL-REF ID-REF=\"sig51\"/>\n          </fx:SIGNAL-INSTANCE>\n          <fx:SIGNAL-INSTANCE ID=\"sgi45\">\n            <fx:BIT-POSITION>16</fx:BIT-POSITION>\n            <fx:IS-HIGH-LOW-BYTE-ORDER>false</fx:IS-HIGH-LOW-BYTE-ORDER>\n            <fx:SIGNAL-REF ID-REF=\"sig52\"/>\n          </fx:SIGNAL-INSTANCE>\n          <fx:SIGNAL-INSTANCE ID=\"sgi46\">\n            <fx:BIT-POSITION>32</fx:BIT-POSITION>\n            <fx:IS-HIGH-LOW-BYTE-ORDER>false</fx:IS-HIGH-LOW-BYTE-ORDER>\n            <fx:SIGNAL-REF ID-REF=\"sig53\"/>\n          </fx:SIGNAL-INSTANCE>\n          <fx:SIGNAL-INSTANCE ID=\"sgi47\">\n            <fx:BIT-POSITION>48</fx:BIT-POSITION>\n            <fx:IS-HIGH-LOW-BYTE-ORDER>false</fx:IS-HIGH-LOW-BYTE-ORDER>\n            <fx:SIGNAL-REF ID-REF=\"sig54\"/>\n          </fx:SIGNAL-INSTANCE>\n        </fx:SIGNAL-INSTANCES>\n      </fx:PDU>\n      <fx:PDU ID=\"pdu16\">\n        <ho:SHORT-NAME>Cell_V_Set_5_8_pdu</ho:SHORT-NAME>\n        <ho:DESC></ho:DESC>\n        <fx:BYTE-LENGTH>8</fx:BYTE-LENGTH>\n        <fx:PDU-TYPE>APPLICATION</fx:PDU-TYPE>\n        <fx:SIGNAL-INSTANCES>\n          <fx:SIGNAL-INSTANCE ID=\"sgi48\">\n            <fx:BIT-POSITION>0</fx:BIT-POSITION>\n            <fx:IS-HIGH-LOW-BYTE-ORDER>false</fx:IS-HIGH-LOW-BYTE-ORDER>\n            <fx:SIGNAL-REF ID-REF=\"sig55\"/>\n          </fx:SIGNAL-INSTANCE>\n          <fx:SIGNAL-INSTANCE ID=\"sgi49\">\n            <fx:BIT-POSITION>16</fx:BIT-POSITION>\n            <fx:IS-HIGH-LOW-BYTE-ORDER>false</fx:IS-HIGH-LOW-BYTE-ORDER>\n            <fx:SIGNAL-REF ID-REF=\"sig56\"/>\n          </fx:SIGNAL-INSTANCE>\n          <fx:SIGNAL-INSTANCE ID=\"sgi50\">\n            <fx:BIT-POSITION>32</fx:BIT-POSITION>\n            <fx:IS-HIGH-LOW-BYTE-ORDER>false</fx:IS-HIGH-LOW-BYTE-ORDER>\n            <fx:SIGNAL-REF ID-REF=\"sig57\"/>\n          </fx:SIGNAL-INSTANCE>\n          <fx:SIGNAL-INSTANCE ID=\"sgi51\">\n            <fx:BIT-POSITION>48</fx:BIT-POSITION>\n            <fx:IS-HIGH-LOW-BYTE-ORDER>false</fx:IS-HIGH-LOW-BYTE-ORDER>\n            <fx:SIGNAL-REF ID-REF=\"sig58\"/>\n          </fx:SIGNAL-INSTANCE>\n        </fx:SIGNAL-INSTANCES>\n      </fx:PDU>\n      <fx:PDU ID=\"pdu17\">\n        <ho:SHORT-NAME>Cell_V_Set_9_12_pdu</ho:SHORT-NAME>\n        <ho:DESC></ho:DESC>\n        <fx:BYTE-LENGTH>8</fx:BYTE-LENGTH>\n        <fx:PDU-TYPE>APPLICATION</fx:PDU-TYPE>\n        <fx:SIGNAL-INSTANCES>\n          <fx:SIGNAL-INSTANCE ID=\"sgi52\">\n            <fx:BIT-POSITION>0</fx:BIT-POSITION>\n            <fx:IS-HIGH-LOW-BYTE-ORDER>false</fx:IS-HIGH-LOW-BYTE-ORDER>\n            <fx:SIGNAL-REF ID-REF=\"sig2\"/>\n          </fx:SIGNAL-INSTANCE>\n          <fx:SIGNAL-INSTANCE ID=\"sgi53\">\n            <fx:BIT-POSITION>16</fx:BIT-POSITION>\n            <fx:IS-HIGH-LOW-BYTE-ORDER>false</fx:IS-HIGH-LOW-BYTE-ORDER>\n            <fx:SIGNAL-REF ID-REF=\"sig3\"/>\n          </fx:SIGNAL-INSTANCE>\n          <fx:SIGNAL-INSTANCE ID=\"sgi54\">\n            <fx:BIT-POSITION>32</fx:BIT-POSITION>\n            <fx:IS-HIGH-LOW-BYTE-ORDER>false</fx:IS-HIGH-LOW-BYTE-ORDER>\n            <fx:SIGNAL-REF ID-REF=\"sig4\"/>\n          </fx:SIGNAL-INSTANCE>\n          <fx:SIGNAL-INSTANCE ID=\"sgi55\">\n            <fx:BIT-POSITION>48</fx:BIT-POSITION>\n            <fx:IS-HIGH-LOW-BYTE-ORDER>false</fx:IS-HIGH-LOW-BYTE-ORDER>\n            <fx:SIGNAL-REF ID-REF=\"sig5\"/>\n          </fx:SIGNAL-INSTANCE>\n        </fx:SIGNAL-INSTANCES>\n      </fx:PDU>\n      <fx:PDU ID=\"pdu18\">\n        <ho:SHORT-NAME>Cell_V_Set_All_pdu</ho:SHORT-NAME>\n        <ho:DESC></ho:DESC>\n        <fx:BYTE-LENGTH>2</fx:BYTE-LENGTH>\n        <fx:PDU-TYPE>APPLICATION</fx:PDU-TYPE>\n        <fx:SIGNAL-INSTANCES>\n          <fx:SIGNAL-INSTANCE ID=\"sgi56\">\n            <fx:BIT-POSITION>0</fx:BIT-POSITION>\n            <fx:IS-HIGH-LOW-BYTE-ORDER>false</fx:IS-HIGH-LOW-BYTE-ORDER>\n            <fx:SIGNAL-REF ID-REF=\"sig8\"/>\n          </fx:SIGNAL-INSTANCE>\n        </fx:SIGNAL-INSTANCES>\n      </fx:PDU>\n      <fx:PDU ID=\"pdu19\">\n        <ho:SHORT-NAME>Cell_V_Set_pdu</ho:SHORT-NAME>\n        <ho:DESC></ho:DESC>\n        <fx:BYTE-LENGTH>3</fx:BYTE-LENGTH>\n        <fx:PDU-TYPE>APPLICATION</fx:PDU-TYPE>\n        <fx:SIGNAL-INSTANCES>\n          <fx:SIGNAL-INSTANCE ID=\"sgi57\">\n            <fx:BIT-POSITION>0</fx:BIT-POSITION>\n            <fx:IS-HIGH-LOW-BYTE-ORDER>false</fx:IS-HIGH-LOW-BYTE-ORDER>\n            <fx:SIGNAL-REF ID-REF=\"sig23\"/>\n          </fx:SIGNAL-INSTANCE>\n          <fx:SIGNAL-INSTANCE ID=\"sgi58\">\n            <fx:BIT-POSITION>8</fx:BIT-POSITION>\n            <fx:IS-HIGH-LOW-BYTE-ORDER>false</fx:IS-HIGH-LOW-BYTE-ORDER>\n            <fx:SIGNAL-REF ID-REF=\"sig24\"/>\n          </fx:SIGNAL-INSTANCE>\n        </fx:SIGNAL-INSTANCES>\n      </fx:PDU>\n      <fx:PDU ID=\"pdu20\">\n        <ho:SHORT-NAME>Configure_pdu</ho:SHORT-NAME>\n        <ho:DESC></ho:DESC>\n        <fx:BYTE-LENGTH>3</fx:BYTE-LENGTH>\n        <fx:PDU-TYPE>APPLICATION</fx:PDU-TYPE>\n        <fx:SIGNAL-INSTANCES>\n          <fx:SIGNAL-INSTANCE ID=\"sgi59\">\n            <fx:BIT-POSITION>0</fx:BIT-POSITION>\n            <fx:IS-HIGH-LOW-BYTE-ORDER>false</fx:IS-HIGH-LOW-BYTE-ORDER>\n            <fx:SIGNAL-REF ID-REF=\"sig13\"/>\n          </fx:SIGNAL-INSTANCE>\n          <fx:SIGNAL-INSTANCE ID=\"sgi60\">\n            <fx:BIT-POSITION>1</fx:BIT-POSITION>\n            <fx:IS-HIGH-LOW-BYTE-ORDER>false</fx:IS-HIGH-LOW-BYTE-ORDER>\n            <fx:SIGNAL-REF ID-REF=\"sig14\"/>\n          </fx:SIGNAL-INSTANCE>\n          <fx:SIGNAL-INSTANCE ID=\"sgi61\">\n            <fx:BIT-POSITION>8</fx:BIT-POSITION>\n            <fx:IS-HIGH-LOW-BYTE-ORDER>false</fx:IS-HIGH-LOW-BYTE-ORDER>\n            <fx:SIGNAL-REF ID-REF=\"sig15\"/>\n          </fx:SIGNAL-INSTANCE>\n          <fx:SIGNAL-INSTANCE ID=\"sgi62\">\n            <fx:BIT-POSITION>9</fx:BIT-POSITION>\n            <fx:IS-HIGH-LOW-BYTE-ORDER>false</fx:IS-HIGH-LOW-BYTE-ORDER>\n            <fx:SIGNAL-REF ID-REF=\"sig16\"/>\n          </fx:SIGNAL-INSTANCE>\n          <fx:SIGNAL-INSTANCE ID=\"sgi63\">\n            <fx:BIT-POSITION>10</fx:BIT-POSITION>\n            <fx:IS-HIGH-LOW-BYTE-ORDER>false</fx:IS-HIGH-LOW-BYTE-ORDER>\n            <fx:SIGNAL-REF ID-REF=\"sig17\"/>\n          </fx:SIGNAL-INSTANCE>\n          <fx:SIGNAL-INSTANCE ID=\"sgi64\">\n            <fx:BIT-POSITION>16</fx:BIT-POSITION>\n            <fx:IS-HIGH-LOW-BYTE-ORDER>false</fx:IS-HIGH-LOW-BYTE-ORDER>\n            <fx:SIGNAL-REF ID-REF=\"sig18\"/>\n          </fx:SIGNAL-INSTANCE>\n        </fx:SIGNAL-INSTANCES>\n      </fx:PDU>\n      <fx:PDU ID=\"pdu21\">\n        <ho:SHORT-NAME>DIO_Readback_1_8_pdu</ho:SHORT-NAME>\n        <ho:DESC></ho:DESC>\n        <fx:BYTE-LENGTH>8</fx:BYTE-LENGTH>\n        <fx:PDU-TYPE>APPLICATION</fx:PDU-TYPE>\n        <fx:SIGNAL-INSTANCES>\n          <fx:SIGNAL-INSTANCE ID=\"sgi65\">\n            <fx:BIT-POSITION>0</fx:BIT-POSITION>\n            <fx:IS-HIGH-LOW-BYTE-ORDER>false</fx:IS-HIGH-LOW-BYTE-ORDER>\n            <fx:SIGNAL-REF ID-REF=\"sig67\"/>\n          </fx:SIGNAL-INSTANCE>\n        </fx:SIGNAL-INSTANCES>\n      </fx:PDU>\n      <fx:PDU ID=\"pdu22\">\n        <ho:SHORT-NAME>Digital_IO_Set_1_8_pdu</ho:SHORT-NAME>\n        <ho:DESC></ho:DESC>\n        <fx:BYTE-LENGTH>2</fx:BYTE-LENGTH>\n        <fx:PDU-TYPE>APPLICATION</fx:PDU-TYPE>\n        <fx:SIGNAL-INSTANCES>\n          <fx:SIGNAL-INSTANCE ID=\"sgi66\">\n            <fx:BIT-POSITION>0</fx:BIT-POSITION>\n            <fx:IS-HIGH-LOW-BYTE-ORDER>false</fx:IS-HIGH-LOW-BYTE-ORDER>\n            <fx:SIGNAL-REF ID-REF=\"sig9\"/>\n          </fx:SIGNAL-INSTANCE>\n          <fx:SIGNAL-INSTANCE ID=\"sgi67\">\n            <fx:BIT-POSITION>8</fx:BIT-POSITION>\n            <fx:IS-HIGH-LOW-BYTE-ORDER>false</fx:IS-HIGH-LOW-BYTE-ORDER>\n            <fx:SIGNAL-REF ID-REF=\"sig10\"/>\n          </fx:SIGNAL-INSTANCE>\n        </fx:SIGNAL-INSTANCES>\n      </fx:PDU>\n      <fx:PDU ID=\"pdu23\">\n        <ho:SHORT-NAME>HIL_Mode_pdu</ho:SHORT-NAME>\n        <ho:DESC></ho:DESC>\n        <fx:BYTE-LENGTH>1</fx:BYTE-LENGTH>\n        <fx:PDU-TYPE>APPLICATION</fx:PDU-TYPE>\n        <fx:SIGNAL-INSTANCES>\n          <fx:SIGNAL-INSTANCE ID=\"sgi68\">\n            <fx:BIT-POSITION>0</fx:BIT-POSITION>\n            <fx:IS-HIGH-LOW-BYTE-ORDER>false</fx:IS-HIGH-LOW-BYTE-ORDER>\n            <fx:SIGNAL-REF ID-REF=\"sig1\"/>\n          </fx:SIGNAL-INSTANCE>\n        </fx:SIGNAL-INSTANCES>\n      </fx:PDU>\n      <fx:PDU ID=\"pdu24\">\n        <ho:SHORT-NAME>System_Status_pdu</ho:SHORT-NAME>\n        <ho:DESC></ho:DESC>\n        <fx:BYTE-LENGTH>8</fx:BYTE-LENGTH>\n        <fx:PDU-TYPE>APPLICATION</fx:PDU-TYPE>\n        <fx:SIGNAL-INSTANCES>\n          <fx:SIGNAL-INSTANCE ID=\"sgi69\">\n            <fx:BIT-POSITION>8</fx:BIT-POSITION>\n            <fx:IS-HIGH-LOW-BYTE-ORDER>false</fx:IS-HIGH-LOW-BYTE-ORDER>\n            <fx:SIGNAL-REF ID-REF=\"sig36\"/>\n          </fx:SIGNAL-INSTANCE>\n          <fx:SIGNAL-INSTANCE ID=\"sgi70\">\n            <fx:BIT-POSITION>16</fx:BIT-POSITION>\n            <fx:IS-HIGH-LOW-BYTE-ORDER>false</fx:IS-HIGH-LOW-BYTE-ORDER>\n            <fx:SIGNAL-REF ID-REF=\"sig37\"/>\n          </fx:SIGNAL-INSTANCE>\n          <fx:SIGNAL-INSTANCE ID=\"sgi71\">\n            <fx:BIT-POSITION>24</fx:BIT-POSITION>\n            <fx:IS-HIGH-LOW-BYTE-ORDER>false</fx:IS-HIGH-LOW-BYTE-ORDER>\n            <fx:SIGNAL-REF ID-REF=\"sig38\"/>\n          </fx:SIGNAL-INSTANCE>\n          <fx:SIGNAL-INSTANCE ID=\"sgi72\">\n            <fx:BIT-POSITION>0</fx:BIT-POSITION>\n            <fx:IS-HIGH-LOW-BYTE-ORDER>false</fx:IS-HIGH-LOW-BYTE-ORDER>\n            <fx:SIGNAL-REF ID-REF=\"sig39\"/>\n          </fx:SIGNAL-INSTANCE>\n          <fx:SIGNAL-INSTANCE ID=\"sgi73\">\n            <fx:BIT-POSITION>1</fx:BIT-POSITION>\n            <fx:IS-HIGH-LOW-BYTE-ORDER>false</fx:IS-HIGH-LOW-BYTE-ORDER>\n            <fx:SIGNAL-REF ID-REF=\"sig40\"/>\n          </fx:SIGNAL-INSTANCE>\n          <fx:SIGNAL-INSTANCE ID=\"sgi74\">\n            <fx:BIT-POSITION>2</fx:BIT-POSITION>\n            <fx:IS-HIGH-LOW-BYTE-ORDER>false</fx:IS-HIGH-LOW-BYTE-ORDER>\n            <fx:SIGNAL-REF ID-REF=\"sig41\"/>\n          </fx:SIGNAL-INSTANCE>\n          <fx:SIGNAL-INSTANCE ID=\"sgi75\">\n            <fx:BIT-POSITION>3</fx:BIT-POSITION>\n            <fx:IS-HIGH-LOW-BYTE-ORDER>false</fx:IS-HIGH-LOW-BYTE-ORDER>\n            <fx:SIGNAL-REF ID-REF=\"sig42\"/>\n          </fx:SIGNAL-INSTANCE>\n        </fx:SIGNAL-INSTANCES>\n      </fx:PDU>\n    </fx:PDUS>\n    <fx:FRAMES>\n      <fx:FRAME ID=\"frm1\">\n        <ho:SHORT-NAME>HIL_Mode</ho:SHORT-NAME>\n        <ho:DESC></ho:DESC>\n        <fx:BYTE-LENGTH>1</fx:BYTE-LENGTH>\n        <fx:PDU-INSTANCES>\n          <fx:PDU-INSTANCE ID=\"pduinst1\">\n            <fx:PDU-REF ID-REF=\"pdu23\"/>\n            <fx:BIT-POSITION>0</fx:BIT-POSITION>\n            <fx:IS-HIGH-LOW-BYTE-ORDER>false</fx:IS-HIGH-LOW-BYTE-ORDER>\n          </fx:PDU-INSTANCE>\n        </fx:PDU-INSTANCES>\n      </fx:FRAME>\n      <fx:FRAME ID=\"frm2\">\n        <ho:SHORT-NAME>Cell_V_Set_9_12</ho:SHORT-NAME>\n        <ho:DESC></ho:DESC>\n        <fx:BYTE-LENGTH>8</fx:BYTE-LENGTH>\n        <fx:PDU-INSTANCES>\n          <fx:PDU-INSTANCE ID=\"pduinst2\">\n            <fx:PDU-REF ID-REF=\"pdu17\"/>\n            <fx:BIT-POSITION>0</fx:BIT-POSITION>\n            <fx:IS-HIGH-LOW-BYTE-ORDER>false</fx:IS-HIGH-LOW-BYTE-ORDER>\n          </fx:PDU-INSTANCE>\n        </fx:PDU-INSTANCES>\n      </fx:FRAME>\n      <fx:FRAME ID=\"frm3\">\n        <ho:SHORT-NAME>Cell_I_Source_Set</ho:SHORT-NAME>\n        <ho:DESC></ho:DESC>\n        <fx:BYTE-LENGTH>3</fx:BYTE-LENGTH>\n        <fx:PDU-INSTANCES>\n          <fx:PDU-INSTANCE ID=\"pduinst3\">\n            <fx:PDU-REF ID-REF=\"pdu11\"/>\n            <fx:BIT-POSITION>0</fx:BIT-POSITION>\n            <fx:IS-HIGH-LOW-BYTE-ORDER>false</fx:IS-HIGH-LOW-BYTE-ORDER>\n          </fx:PDU-INSTANCE>\n        </fx:PDU-INSTANCES>\n      </fx:FRAME>\n      <fx:FRAME ID=\"frm4\">\n        <ho:SHORT-NAME>Cell_V_Set_All</ho:SHORT-NAME>\n        <ho:DESC></ho:DESC>\n        <fx:BYTE-LENGTH>2</fx:BYTE-LENGTH>\n        <fx:PDU-INSTANCES>\n          <fx:PDU-INSTANCE ID=\"pduinst4\">\n            <fx:PDU-REF ID-REF=\"pdu18\"/>\n            <fx:BIT-POSITION>0</fx:BIT-POSITION>\n            <fx:IS-HIGH-LOW-BYTE-ORDER>false</fx:IS-HIGH-LOW-BYTE-ORDER>\n          </fx:PDU-INSTANCE>\n        </fx:PDU-INSTANCES>\n      </fx:FRAME>\n      <fx:FRAME ID=\"frm5\">\n        <ho:SHORT-NAME>Digital_IO_Set_1_8</ho:SHORT-NAME>\n        <ho:DESC></ho:DESC>\n        <fx:BYTE-LENGTH>2</fx:BYTE-LENGTH>\n        <fx:PDU-INSTANCES>\n          <fx:PDU-INSTANCE ID=\"pduinst5\">\n            <fx:PDU-REF ID-REF=\"pdu22\"/>\n            <fx:BIT-POSITION>0</fx:BIT-POSITION>\n            <fx:IS-HIGH-LOW-BYTE-ORDER>false</fx:IS-HIGH-LOW-BYTE-ORDER>\n          </fx:PDU-INSTANCE>\n        </fx:PDU-INSTANCES>\n      </fx:FRAME>\n      <fx:FRAME ID=\"frm6\">\n        <ho:SHORT-NAME>Analog_Out_Set_1_2</ho:SHORT-NAME>\n        <ho:DESC></ho:DESC>\n        <fx:BYTE-LENGTH>8</fx:BYTE-LENGTH>\n        <fx:PDU-INSTANCES>\n          <fx:PDU-INSTANCE ID=\"pduinst6\">\n            <fx:PDU-REF ID-REF=\"pdu3\"/>\n            <fx:BIT-POSITION>0</fx:BIT-POSITION>\n            <fx:IS-HIGH-LOW-BYTE-ORDER>false</fx:IS-HIGH-LOW-BYTE-ORDER>\n          </fx:PDU-INSTANCE>\n        </fx:PDU-INSTANCES>\n      </fx:FRAME>\n      <fx:FRAME ID=\"frm7\">\n        <ho:SHORT-NAME>Configure</ho:SHORT-NAME>\n        <ho:DESC></ho:DESC>\n        <fx:BYTE-LENGTH>3</fx:BYTE-LENGTH>\n        <fx:PDU-INSTANCES>\n          <fx:PDU-INSTANCE ID=\"pduinst7\">\n            <fx:PDU-REF ID-REF=\"pdu20\"/>\n            <fx:BIT-POSITION>0</fx:BIT-POSITION>\n            <fx:IS-HIGH-LOW-BYTE-ORDER>false</fx:IS-HIGH-LOW-BYTE-ORDER>\n          </fx:PDU-INSTANCE>\n        </fx:PDU-INSTANCES>\n      </fx:FRAME>\n      <fx:FRAME ID=\"frm8\">\n        <ho:SHORT-NAME>Cell_I_Set_All</ho:SHORT-NAME>\n        <ho:DESC></ho:DESC>\n        <fx:BYTE-LENGTH>4</fx:BYTE-LENGTH>\n        <fx:PDU-INSTANCES>\n          <fx:PDU-INSTANCE ID=\"pduinst8\">\n            <fx:PDU-REF ID-REF=\"pdu9\"/>\n            <fx:BIT-POSITION>0</fx:BIT-POSITION>\n            <fx:IS-HIGH-LOW-BYTE-ORDER>false</fx:IS-HIGH-LOW-BYTE-ORDER>\n          </fx:PDU-INSTANCE>\n        </fx:PDU-INSTANCES>\n      </fx:FRAME>\n      <fx:FRAME ID=\"frm9\">\n        <ho:SHORT-NAME>Cell_I_Sink_Set</ho:SHORT-NAME>\n        <ho:DESC></ho:DESC>\n        <fx:BYTE-LENGTH>3</fx:BYTE-LENGTH>\n        <fx:PDU-INSTANCES>\n          <fx:PDU-INSTANCE ID=\"pduinst9\">\n            <fx:PDU-REF ID-REF=\"pdu10\"/>\n            <fx:BIT-POSITION>0</fx:BIT-POSITION>\n            <fx:IS-HIGH-LOW-BYTE-ORDER>false</fx:IS-HIGH-LOW-BYTE-ORDER>\n          </fx:PDU-INSTANCE>\n        </fx:PDU-INSTANCES>\n      </fx:FRAME>\n      <fx:FRAME ID=\"frm10\">\n        <ho:SHORT-NAME>Cell_V_Set</ho:SHORT-NAME>\n        <ho:DESC></ho:DESC>\n        <fx:BYTE-LENGTH>3</fx:BYTE-LENGTH>\n        <fx:PDU-INSTANCES>\n          <fx:PDU-INSTANCE ID=\"pduinst10\">\n            <fx:PDU-REF ID-REF=\"pdu19\"/>\n            <fx:BIT-POSITION>0</fx:BIT-POSITION>\n            <fx:IS-HIGH-LOW-BYTE-ORDER>false</fx:IS-HIGH-LOW-BYTE-ORDER>\n          </fx:PDU-INSTANCE>\n        </fx:PDU-INSTANCES>\n      </fx:FRAME>\n      <fx:FRAME ID=\"frm11\">\n        <ho:SHORT-NAME>Cell_V_Readback_9_12</ho:SHORT-NAME>\n        <ho:DESC></ho:DESC>\n        <fx:BYTE-LENGTH>8</fx:BYTE-LENGTH>\n        <fx:PDU-INSTANCES>\n          <fx:PDU-INSTANCE ID=\"pduinst11\">\n            <fx:PDU-REF ID-REF=\"pdu14\"/>\n            <fx:BIT-POSITION>0</fx:BIT-POSITION>\n            <fx:IS-HIGH-LOW-BYTE-ORDER>false</fx:IS-HIGH-LOW-BYTE-ORDER>\n          </fx:PDU-INSTANCE>\n        </fx:PDU-INSTANCES>\n      </fx:FRAME>\n      <fx:FRAME ID=\"frm12\">\n        <ho:SHORT-NAME>Cell_I_Readback_1_4</ho:SHORT-NAME>\n        <ho:DESC></ho:DESC>\n        <fx:BYTE-LENGTH>8</fx:BYTE-LENGTH>\n        <fx:PDU-INSTANCES>\n          <fx:PDU-INSTANCE ID=\"pduinst12\">\n            <fx:PDU-REF ID-REF=\"pdu6\"/>\n            <fx:BIT-POSITION>0</fx:BIT-POSITION>\n            <fx:IS-HIGH-LOW-BYTE-ORDER>false</fx:IS-HIGH-LOW-BYTE-ORDER>\n          </fx:PDU-INSTANCE>\n        </fx:PDU-INSTANCES>\n      </fx:FRAME>\n      <fx:FRAME ID=\"frm13\">\n        <ho:SHORT-NAME>Cell_Enable_All</ho:SHORT-NAME>\n        <ho:DESC></ho:DESC>\n        <fx:BYTE-LENGTH>1</fx:BYTE-LENGTH>\n        <fx:PDU-INSTANCES>\n          <fx:PDU-INSTANCE ID=\"pduinst13\">\n            <fx:PDU-REF ID-REF=\"pdu4\"/>\n            <fx:BIT-POSITION>0</fx:BIT-POSITION>\n            <fx:IS-HIGH-LOW-BYTE-ORDER>false</fx:IS-HIGH-LOW-BYTE-ORDER>\n          </fx:PDU-INSTANCE>\n        </fx:PDU-INSTANCES>\n      </fx:FRAME>\n      <fx:FRAME ID=\"frm14\">\n        <ho:SHORT-NAME>Cell_Enable</ho:SHORT-NAME>\n        <ho:DESC></ho:DESC>\n        <fx:BYTE-LENGTH>2</fx:BYTE-LENGTH>\n        <fx:PDU-INSTANCES>\n          <fx:PDU-INSTANCE ID=\"pduinst14\">\n            <fx:PDU-REF ID-REF=\"pdu5\"/>\n            <fx:BIT-POSITION>0</fx:BIT-POSITION>\n            <fx:IS-HIGH-LOW-BYTE-ORDER>false</fx:IS-HIGH-LOW-BYTE-ORDER>\n          </fx:PDU-INSTANCE>\n        </fx:PDU-INSTANCES>\n      </fx:FRAME>\n      <fx:FRAME ID=\"frm15\">\n        <ho:SHORT-NAME>System_Status</ho:SHORT-NAME>\n        <ho:DESC></ho:DESC>\n        <fx:BYTE-LENGTH>8</fx:BYTE-LENGTH>\n        <fx:PDU-INSTANCES>\n          <fx:PDU-INSTANCE ID=\"pduinst15\">\n            <fx:PDU-REF ID-REF=\"pdu24\"/>\n            <fx:BIT-POSITION>0</fx:BIT-POSITION>\n            <fx:IS-HIGH-LOW-BYTE-ORDER>false</fx:IS-HIGH-LOW-BYTE-ORDER>\n          </fx:PDU-INSTANCE>\n        </fx:PDU-INSTANCES>\n      </fx:FRAME>\n      <fx:FRAME ID=\"frm16\">\n        <ho:SHORT-NAME>Cell_V_Readback_1_4</ho:SHORT-NAME>\n        <ho:DESC></ho:DESC>\n        <fx:BYTE-LENGTH>8</fx:BYTE-LENGTH>\n        <fx:PDU-INSTANCES>\n          <fx:PDU-INSTANCE ID=\"pduinst16\">\n            <fx:PDU-REF ID-REF=\"pdu12\"/>\n            <fx:BIT-POSITION>0</fx:BIT-POSITION>\n            <fx:IS-HIGH-LOW-BYTE-ORDER>false</fx:IS-HIGH-LOW-BYTE-ORDER>\n          </fx:PDU-INSTANCE>\n        </fx:PDU-INSTANCES>\n      </fx:FRAME>\n      <fx:FRAME ID=\"frm17\">\n        <ho:SHORT-NAME>Cell_V_Readback_5_8</ho:SHORT-NAME>\n        <ho:DESC></ho:DESC>\n        <fx:BYTE-LENGTH>8</fx:BYTE-LENGTH>\n        <fx:PDU-INSTANCES>\n          <fx:PDU-INSTANCE ID=\"pduinst17\">\n            <fx:PDU-REF ID-REF=\"pdu13\"/>\n            <fx:BIT-POSITION>0</fx:BIT-POSITION>\n            <fx:IS-HIGH-LOW-BYTE-ORDER>false</fx:IS-HIGH-LOW-BYTE-ORDER>\n          </fx:PDU-INSTANCE>\n        </fx:PDU-INSTANCES>\n      </fx:FRAME>\n      <fx:FRAME ID=\"frm18\">\n        <ho:SHORT-NAME>Cell_V_Set_1_4</ho:SHORT-NAME>\n        <ho:DESC></ho:DESC>\n        <fx:BYTE-LENGTH>8</fx:BYTE-LENGTH>\n        <fx:PDU-INSTANCES>\n          <fx:PDU-INSTANCE ID=\"pduinst18\">\n            <fx:PDU-REF ID-REF=\"pdu15\"/>\n            <fx:BIT-POSITION>0</fx:BIT-POSITION>\n            <fx:IS-HIGH-LOW-BYTE-ORDER>false</fx:IS-HIGH-LOW-BYTE-ORDER>\n          </fx:PDU-INSTANCE>\n        </fx:PDU-INSTANCES>\n      </fx:FRAME>\n      <fx:FRAME ID=\"frm19\">\n        <ho:SHORT-NAME>Cell_V_Set_5_8</ho:SHORT-NAME>\n        <ho:DESC></ho:DESC>\n        <fx:BYTE-LENGTH>8</fx:BYTE-LENGTH>\n        <fx:PDU-INSTANCES>\n          <fx:PDU-INSTANCE ID=\"pduinst19\">\n            <fx:PDU-REF ID-REF=\"pdu16\"/>\n            <fx:BIT-POSITION>0</fx:BIT-POSITION>\n            <fx:IS-HIGH-LOW-BYTE-ORDER>false</fx:IS-HIGH-LOW-BYTE-ORDER>\n          </fx:PDU-INSTANCE>\n        </fx:PDU-INSTANCES>\n      </fx:FRAME>\n      <fx:FRAME ID=\"frm20\">\n        <ho:SHORT-NAME>Cell_I_Readback_5_8</ho:SHORT-NAME>\n        <ho:DESC></ho:DESC>\n        <fx:BYTE-LENGTH>8</fx:BYTE-LENGTH>\n        <fx:PDU-INSTANCES>\n          <fx:PDU-INSTANCE ID=\"pduinst20\">\n            <fx:PDU-REF ID-REF=\"pdu7\"/>\n            <fx:BIT-POSITION>0</fx:BIT-POSITION>\n            <fx:IS-HIGH-LOW-BYTE-ORDER>false</fx:IS-HIGH-LOW-BYTE-ORDER>\n          </fx:PDU-INSTANCE>\n        </fx:PDU-INSTANCES>\n      </fx:FRAME>\n      <fx:FRAME ID=\"frm21\">\n        <ho:SHORT-NAME>Cell_I_Readback_9_12</ho:SHORT-NAME>\n        <ho:DESC></ho:DESC>\n        <fx:BYTE-LENGTH>8</fx:BYTE-LENGTH>\n        <fx:PDU-INSTANCES>\n          <fx:PDU-INSTANCE ID=\"pduinst21\">\n            <fx:PDU-REF ID-REF=\"pdu8\"/>\n            <fx:BIT-POSITION>0</fx:BIT-POSITION>\n            <fx:IS-HIGH-LOW-BYTE-ORDER>false</fx:IS-HIGH-LOW-BYTE-ORDER>\n          </fx:PDU-INSTANCE>\n        </fx:PDU-INSTANCES>\n      </fx:FRAME>\n      <fx:FRAME ID=\"frm22\">\n        <ho:SHORT-NAME>DIO_Readback_1_8</ho:SHORT-NAME>\n        <ho:DESC></ho:DESC>\n        <fx:BYTE-LENGTH>8</fx:BYTE-LENGTH>\n        <fx:PDU-INSTANCES>\n          <fx:PDU-INSTANCE ID=\"pduinst22\">\n            <fx:PDU-REF ID-REF=\"pdu21\"/>\n            <fx:BIT-POSITION>0</fx:BIT-POSITION>\n            <fx:IS-HIGH-LOW-BYTE-ORDER>false</fx:IS-HIGH-LOW-BYTE-ORDER>\n          </fx:PDU-INSTANCE>\n        </fx:PDU-INSTANCES>\n      </fx:FRAME>\n      <fx:FRAME ID=\"frm23\">\n        <ho:SHORT-NAME>AI_Readback_1_4</ho:SHORT-NAME>\n        <ho:DESC></ho:DESC>\n        <fx:BYTE-LENGTH>8</fx:BYTE-LENGTH>\n        <fx:PDU-INSTANCES>\n          <fx:PDU-INSTANCE ID=\"pduinst23\">\n            <fx:PDU-REF ID-REF=\"pdu1\"/>\n            <fx:BIT-POSITION>0</fx:BIT-POSITION>\n            <fx:IS-HIGH-LOW-BYTE-ORDER>false</fx:IS-HIGH-LOW-BYTE-ORDER>\n          </fx:PDU-INSTANCE>\n        </fx:PDU-INSTANCES>\n      </fx:FRAME>\n      <fx:FRAME ID=\"frm24\">\n        <ho:SHORT-NAME>AI_Readback_5_8</ho:SHORT-NAME>\n        <ho:DESC></ho:DESC>\n        <fx:BYTE-LENGTH>8</fx:BYTE-LENGTH>\n        <fx:PDU-INSTANCES>\n          <fx:PDU-INSTANCE ID=\"pduinst24\">\n            <fx:PDU-REF ID-REF=\"pdu2\"/>\n            <fx:BIT-POSITION>0</fx:BIT-POSITION>\n            <fx:IS-HIGH-LOW-BYTE-ORDER>false</fx:IS-HIGH-LOW-BYTE-ORDER>\n          </fx:PDU-INSTANCE>\n        </fx:PDU-INSTANCES>\n      </fx:FRAME>\n    </fx:FRAMES>\n    <fx:SIGNALS>\n      <fx:SIGNAL ID=\"sig1\">\n        <ho:SHORT-NAME>Enable</ho:SHORT-NAME>\n        <ho:DESC>Set to True to enable HIL mode</ho:DESC>\n        <fx:DEFAULT-VALUE>0</fx:DEFAULT-VALUE>\n        <fx:CODING-REF ID-REF=\"cod1\"/>\n      </fx:SIGNAL>\n      <fx:SIGNAL ID=\"sig2\">\n        <ho:SHORT-NAME>Cell_Voltage_9</ho:SHORT-NAME>\n        <fx:DEFAULT-VALUE>0</fx:DEFAULT-VALUE>\n        <fx:CODING-REF ID-REF=\"cod2\"/>\n      </fx:SIGNAL>\n      <fx:SIGNAL ID=\"sig3\">\n        <ho:SHORT-NAME>Cell_Voltage_10</ho:SHORT-NAME>\n        <fx:DEFAULT-VALUE>0</fx:DEFAULT-VALUE>\n        <fx:CODING-REF ID-REF=\"cod3\"/>\n      </fx:SIGNAL>\n      <fx:SIGNAL ID=\"sig4\">\n        <ho:SHORT-NAME>Cell_Voltage_11</ho:SHORT-NAME>\n        <fx:DEFAULT-VALUE>0</fx:DEFAULT-VALUE>\n        <fx:CODING-REF ID-REF=\"cod4\"/>\n      </fx:SIGNAL>\n      <fx:SIGNAL ID=\"sig5\">\n        <ho:SHORT-NAME>Cell_Voltage_12</ho:SHORT-NAME>\n        <fx:DEFAULT-VALUE>0</fx:DEFAULT-VALUE>\n        <fx:CODING-REF ID-REF=\"cod5\"/>\n      </fx:SIGNAL>\n      <fx:SIGNAL ID=\"sig6\">\n        <ho:SHORT-NAME>Channel</ho:SHORT-NAME>\n        <fx:DEFAULT-VALUE>1</fx:DEFAULT-VALUE>\n        <fx:CODING-REF ID-REF=\"cod6\"/>\n      </fx:SIGNAL>\n      <fx:SIGNAL ID=\"sig7\">\n        <ho:SHORT-NAME>I_Source</ho:SHORT-NAME>\n        <fx:DEFAULT-VALUE>0</fx:DEFAULT-VALUE>\n        <fx:CODING-REF ID-REF=\"cod7\"/>\n      </fx:SIGNAL>\n      <fx:SIGNAL ID=\"sig8\">\n        <ho:SHORT-NAME>Cell_Voltage_All</ho:SHORT-NAME>\n        <fx:DEFAULT-VALUE>0</fx:DEFAULT-VALUE>\n        <fx:CODING-REF ID-REF=\"cod8\"/>\n      </fx:SIGNAL>\n      <fx:SIGNAL ID=\"sig9\">\n        <ho:SHORT-NAME>DIO_Output_Val</ho:SHORT-NAME>\n        <fx:DEFAULT-VALUE>0</fx:DEFAULT-VALUE>\n        <fx:CODING-REF ID-REF=\"cod9\"/>\n      </fx:SIGNAL>\n      <fx:SIGNAL ID=\"sig10\">\n        <ho:SHORT-NAME>DIO_Direction</ho:SHORT-NAME>\n        <fx:DEFAULT-VALUE>0</fx:DEFAULT-VALUE>\n        <fx:CODING-REF ID-REF=\"cod10\"/>\n      </fx:SIGNAL>\n      <fx:SIGNAL ID=\"sig11\">\n        <ho:SHORT-NAME>AO1_Voltage</ho:SHORT-NAME>\n        <fx:DEFAULT-VALUE>0</fx:DEFAULT-VALUE>\n        <fx:CODING-REF ID-REF=\"cod11\"/>\n      </fx:SIGNAL>\n      <fx:SIGNAL ID=\"sig12\">\n        <ho:SHORT-NAME>AO2_Voltage</ho:SHORT-NAME>\n        <fx:DEFAULT-VALUE>0</fx:DEFAULT-VALUE>\n        <fx:CODING-REF ID-REF=\"cod12\"/>\n      </fx:SIGNAL>\n      <fx:SIGNAL ID=\"sig13\">\n        <ho:SHORT-NAME>DIO_HIL_Set_Enable</ho:SHORT-NAME>\n        <fx:DEFAULT-VALUE>0</fx:DEFAULT-VALUE>\n        <fx:CODING-REF ID-REF=\"cod13\"/>\n      </fx:SIGNAL>\n      <fx:SIGNAL ID=\"sig14\">\n        <ho:SHORT-NAME>AO_HIL_Set_Enable</ho:SHORT-NAME>\n        <fx:DEFAULT-VALUE>0</fx:DEFAULT-VALUE>\n        <fx:CODING-REF ID-REF=\"cod14\"/>\n      </fx:SIGNAL>\n      <fx:SIGNAL ID=\"sig15\">\n        <ho:SHORT-NAME>DIO_HIL_BCast_Enable</ho:SHORT-NAME>\n        <fx:DEFAULT-VALUE>0</fx:DEFAULT-VALUE>\n        <fx:CODING-REF ID-REF=\"cod15\"/>\n      </fx:SIGNAL>\n      <fx:SIGNAL ID=\"sig16\">\n        <ho:SHORT-NAME>AI_1_4_HIL_BCast_Enable</ho:SHORT-NAME>\n        <fx:DEFAULT-VALUE>0</fx:DEFAULT-VALUE>\n        <fx:CODING-REF ID-REF=\"cod16\"/>\n      </fx:SIGNAL>\n      <fx:SIGNAL ID=\"sig17\">\n        <ho:SHORT-NAME>AI_5_8_HIL_BCast_Enable</ho:SHORT-NAME>\n        <fx:DEFAULT-VALUE>0</fx:DEFAULT-VALUE>\n        <fx:CODING-REF ID-REF=\"cod17\"/>\n      </fx:SIGNAL>\n      <fx:SIGNAL ID=\"sig18\">\n        <ho:SHORT-NAME>Calibration_Mode</ho:SHORT-NAME>\n        <fx:DEFAULT-VALUE>0</fx:DEFAULT-VALUE>\n        <fx:CODING-REF ID-REF=\"cod18\"/>\n      </fx:SIGNAL>\n      <fx:SIGNAL ID=\"sig19\">\n        <ho:SHORT-NAME>Source_I_All</ho:SHORT-NAME>\n        <fx:DEFAULT-VALUE>0</fx:DEFAULT-VALUE>\n        <fx:CODING-REF ID-REF=\"cod19\"/>\n      </fx:SIGNAL>\n      <fx:SIGNAL ID=\"sig20\">\n        <ho:SHORT-NAME>Sink_I_All</ho:SHORT-NAME>\n        <fx:DEFAULT-VALUE>0</fx:DEFAULT-VALUE>\n        <fx:CODING-REF ID-REF=\"cod20\"/>\n      </fx:SIGNAL>\n      <fx:SIGNAL ID=\"sig21\">\n        <ho:SHORT-NAME>Channel</ho:SHORT-NAME>\n        <fx:DEFAULT-VALUE>1</fx:DEFAULT-VALUE>\n        <fx:CODING-REF ID-REF=\"cod21\"/>\n      </fx:SIGNAL>\n      <fx:SIGNAL ID=\"sig22\">\n        <ho:SHORT-NAME>I_Sink</ho:SHORT-NAME>\n        <fx:DEFAULT-VALUE>0</fx:DEFAULT-VALUE>\n        <fx:CODING-REF ID-REF=\"cod22\"/>\n      </fx:SIGNAL>\n      <fx:SIGNAL ID=\"sig23\">\n        <ho:SHORT-NAME>Channel</ho:SHORT-NAME>\n        <fx:DEFAULT-VALUE>1</fx:DEFAULT-VALUE>\n        <fx:CODING-REF ID-REF=\"cod23\"/>\n      </fx:SIGNAL>\n      <fx:SIGNAL ID=\"sig24\">\n        <ho:SHORT-NAME>Cell_Voltage</ho:SHORT-NAME>\n        <fx:DEFAULT-VALUE>0</fx:DEFAULT-VALUE>\n        <fx:CODING-REF ID-REF=\"cod24\"/>\n      </fx:SIGNAL>\n      <fx:SIGNAL ID=\"sig25\">\n        <ho:SHORT-NAME>Cell_V_09</ho:SHORT-NAME>\n        <fx:DEFAULT-VALUE>0</fx:DEFAULT-VALUE>\n        <fx:CODING-REF ID-REF=\"cod25\"/>\n      </fx:SIGNAL>\n      <fx:SIGNAL ID=\"sig26\">\n        <ho:SHORT-NAME>Cell_V_10</ho:SHORT-NAME>\n        <fx:DEFAULT-VALUE>0</fx:DEFAULT-VALUE>\n        <fx:CODING-REF ID-REF=\"cod26\"/>\n      </fx:SIGNAL>\n      <fx:SIGNAL ID=\"sig27\">\n        <ho:SHORT-NAME>Cell_V_11</ho:SHORT-NAME>\n        <fx:DEFAULT-VALUE>0</fx:DEFAULT-VALUE>\n        <fx:CODING-REF ID-REF=\"cod27\"/>\n      </fx:SIGNAL>\n      <fx:SIGNAL ID=\"sig28\">\n        <ho:SHORT-NAME>Cell_V_12</ho:SHORT-NAME>\n        <fx:DEFAULT-VALUE>0</fx:DEFAULT-VALUE>\n        <fx:CODING-REF ID-REF=\"cod28\"/>\n      </fx:SIGNAL>\n      <fx:SIGNAL ID=\"sig29\">\n        <ho:SHORT-NAME>Cell_I_1</ho:SHORT-NAME>\n        <fx:DEFAULT-VALUE>0</fx:DEFAULT-VALUE>\n        <fx:CODING-REF ID-REF=\"cod29\"/>\n      </fx:SIGNAL>\n      <fx:SIGNAL ID=\"sig30\">\n        <ho:SHORT-NAME>Cell_I_2</ho:SHORT-NAME>\n        <fx:DEFAULT-VALUE>0</fx:DEFAULT-VALUE>\n        <fx:CODING-REF ID-REF=\"cod30\"/>\n      </fx:SIGNAL>\n      <fx:SIGNAL ID=\"sig31\">\n        <ho:SHORT-NAME>Cell_I_3</ho:SHORT-NAME>\n        <fx:DEFAULT-VALUE>0</fx:DEFAULT-VALUE>\n        <fx:CODING-REF ID-REF=\"cod31\"/>\n      </fx:SIGNAL>\n      <fx:SIGNAL ID=\"sig32\">\n        <ho:SHORT-NAME>Cell_I_4</ho:SHORT-NAME>\n        <fx:DEFAULT-VALUE>0</fx:DEFAULT-VALUE>\n        <fx:CODING-REF ID-REF=\"cod32\"/>\n      </fx:SIGNAL>\n      <fx:SIGNAL ID=\"sig33\">\n        <ho:SHORT-NAME>Enable</ho:SHORT-NAME>\n        <fx:DEFAULT-VALUE>0</fx:DEFAULT-VALUE>\n        <fx:CODING-REF ID-REF=\"cod33\"/>\n      </fx:SIGNAL>\n      <fx:SIGNAL ID=\"sig34\">\n        <ho:SHORT-NAME>Channel</ho:SHORT-NAME>\n        <fx:DEFAULT-VALUE>1</fx:DEFAULT-VALUE>\n        <fx:CODING-REF ID-REF=\"cod34\"/>\n      </fx:SIGNAL>\n      <fx:SIGNAL ID=\"sig35\">\n        <ho:SHORT-NAME>Enable</ho:SHORT-NAME>\n        <fx:DEFAULT-VALUE>0</fx:DEFAULT-VALUE>\n        <fx:CODING-REF ID-REF=\"cod35\"/>\n      </fx:SIGNAL>\n      <fx:SIGNAL ID=\"sig36\">\n        <ho:SHORT-NAME>Temp_Sensor_1</ho:SHORT-NAME>\n        <fx:DEFAULT-VALUE>0</fx:DEFAULT-VALUE>\n        <fx:CODING-REF ID-REF=\"cod36\"/>\n      </fx:SIGNAL>\n      <fx:SIGNAL ID=\"sig37\">\n        <ho:SHORT-NAME>Temp_Sensor_2</ho:SHORT-NAME>\n        <fx:DEFAULT-VALUE>0</fx:DEFAULT-VALUE>\n        <fx:CODING-REF ID-REF=\"cod37\"/>\n      </fx:SIGNAL>\n      <fx:SIGNAL ID=\"sig38\">\n        <ho:SHORT-NAME>Temp_Sensor_3</ho:SHORT-NAME>\n        <fx:DEFAULT-VALUE>0</fx:DEFAULT-VALUE>\n        <fx:CODING-REF ID-REF=\"cod38\"/>\n      </fx:SIGNAL>\n      <fx:SIGNAL ID=\"sig39\">\n        <ho:SHORT-NAME>Fan_Fail_1</ho:SHORT-NAME>\n        <fx:DEFAULT-VALUE>0</fx:DEFAULT-VALUE>\n        <fx:CODING-REF ID-REF=\"cod39\"/>\n      </fx:SIGNAL>\n      <fx:SIGNAL ID=\"sig40\">\n        <ho:SHORT-NAME>Fan_Fail_2</ho:SHORT-NAME>\n        <fx:DEFAULT-VALUE>0</fx:DEFAULT-VALUE>\n        <fx:CODING-REF ID-REF=\"cod40\"/>\n      </fx:SIGNAL>\n      <fx:SIGNAL ID=\"sig41\">\n        <ho:SHORT-NAME>Fan_Fail_3</ho:SHORT-NAME>\n        <fx:DEFAULT-VALUE>0</fx:DEFAULT-VALUE>\n        <fx:CODING-REF ID-REF=\"cod41\"/>\n      </fx:SIGNAL>\n      <fx:SIGNAL ID=\"sig42\">\n        <ho:SHORT-NAME>Fan_Fail_4</ho:SHORT-NAME>\n        <fx:DEFAULT-VALUE>0</fx:DEFAULT-VALUE>\n        <fx:CODING-REF ID-REF=\"cod42\"/>\n      </fx:SIGNAL>\n      <fx:SIGNAL ID=\"sig43\">\n        <ho:SHORT-NAME>Cell_V_1</ho:SHORT-NAME>\n        <fx:DEFAULT-VALUE>0</fx:DEFAULT-VALUE>\n        <fx:CODING-REF ID-REF=\"cod43\"/>\n      </fx:SIGNAL>\n      <fx:SIGNAL ID=\"sig44\">\n        <ho:SHORT-NAME>Cell_V_2</ho:SHORT-NAME>\n        <fx:DEFAULT-VALUE>0</fx:DEFAULT-VALUE>\n        <fx:CODING-REF ID-REF=\"cod44\"/>\n      </fx:SIGNAL>\n      <fx:SIGNAL ID=\"sig45\">\n        <ho:SHORT-NAME>Cell_V_3</ho:SHORT-NAME>\n        <fx:DEFAULT-VALUE>0</fx:DEFAULT-VALUE>\n        <fx:CODING-REF ID-REF=\"cod45\"/>\n      </fx:SIGNAL>\n      <fx:SIGNAL ID=\"sig46\">\n        <ho:SHORT-NAME>Cell_V_4</ho:SHORT-NAME>\n        <fx:DEFAULT-VALUE>0</fx:DEFAULT-VALUE>\n        <fx:CODING-REF ID-REF=\"cod46\"/>\n      </fx:SIGNAL>\n      <fx:SIGNAL ID=\"sig47\">\n        <ho:SHORT-NAME>Cell_V_5</ho:SHORT-NAME>\n        <fx:DEFAULT-VALUE>0</fx:DEFAULT-VALUE>\n        <fx:CODING-REF ID-REF=\"cod47\"/>\n      </fx:SIGNAL>\n      <fx:SIGNAL ID=\"sig48\">\n        <ho:SHORT-NAME>Cell_V_6</ho:SHORT-NAME>\n        <fx:DEFAULT-VALUE>0</fx:DEFAULT-VALUE>\n        <fx:CODING-REF ID-REF=\"cod48\"/>\n      </fx:SIGNAL>\n      <fx:SIGNAL ID=\"sig49\">\n        <ho:SHORT-NAME>Cell_V_7</ho:SHORT-NAME>\n        <fx:DEFAULT-VALUE>0</fx:DEFAULT-VALUE>\n        <fx:CODING-REF ID-REF=\"cod49\"/>\n      </fx:SIGNAL>\n      <fx:SIGNAL ID=\"sig50\">\n        <ho:SHORT-NAME>Cell_V_8</ho:SHORT-NAME>\n        <fx:DEFAULT-VALUE>0</fx:DEFAULT-VALUE>\n        <fx:CODING-REF ID-REF=\"cod50\"/>\n      </fx:SIGNAL>\n      <fx:SIGNAL ID=\"sig51\">\n        <ho:SHORT-NAME>Cell_1_Voltage</ho:SHORT-NAME>\n        <fx:DEFAULT-VALUE>0</fx:DEFAULT-VALUE>\n        <fx:CODING-REF ID-REF=\"cod51\"/>\n      </fx:SIGNAL>\n      <fx:SIGNAL ID=\"sig52\">\n        <ho:SHORT-NAME>Cell_2_Voltage</ho:SHORT-NAME>\n        <fx:DEFAULT-VALUE>0</fx:DEFAULT-VALUE>\n        <fx:CODING-REF ID-REF=\"cod52\"/>\n      </fx:SIGNAL>\n      <fx:SIGNAL ID=\"sig53\">\n        <ho:SHORT-NAME>Cell_3_Voltage</ho:SHORT-NAME>\n        <fx:DEFAULT-VALUE>0</fx:DEFAULT-VALUE>\n        <fx:CODING-REF ID-REF=\"cod53\"/>\n      </fx:SIGNAL>\n      <fx:SIGNAL ID=\"sig54\">\n        <ho:SHORT-NAME>Cell_4_Voltage</ho:SHORT-NAME>\n        <fx:DEFAULT-VALUE>0</fx:DEFAULT-VALUE>\n        <fx:CODING-REF ID-REF=\"cod54\"/>\n      </fx:SIGNAL>\n      <fx:SIGNAL ID=\"sig55\">\n        <ho:SHORT-NAME>Cell_5_Voltage</ho:SHORT-NAME>\n        <fx:DEFAULT-VALUE>0</fx:DEFAULT-VALUE>\n        <fx:CODING-REF ID-REF=\"cod55\"/>\n      </fx:SIGNAL>\n      <fx:SIGNAL ID=\"sig56\">\n        <ho:SHORT-NAME>Cell_6_Voltage</ho:SHORT-NAME>\n        <fx:DEFAULT-VALUE>0</fx:DEFAULT-VALUE>\n        <fx:CODING-REF ID-REF=\"cod56\"/>\n      </fx:SIGNAL>\n      <fx:SIGNAL ID=\"sig57\">\n        <ho:SHORT-NAME>Cell_7_Voltage</ho:SHORT-NAME>\n        <fx:DEFAULT-VALUE>0</fx:DEFAULT-VALUE>\n        <fx:CODING-REF ID-REF=\"cod57\"/>\n      </fx:SIGNAL>\n      <fx:SIGNAL ID=\"sig58\">\n        <ho:SHORT-NAME>Cell_8_Voltage</ho:SHORT-NAME>\n        <fx:DEFAULT-VALUE>0</fx:DEFAULT-VALUE>\n        <fx:CODING-REF ID-REF=\"cod58\"/>\n      </fx:SIGNAL>\n      <fx:SIGNAL ID=\"sig59\">\n        <ho:SHORT-NAME>Cell_I_5</ho:SHORT-NAME>\n        <fx:DEFAULT-VALUE>0</fx:DEFAULT-VALUE>\n        <fx:CODING-REF ID-REF=\"cod59\"/>\n      </fx:SIGNAL>\n      <fx:SIGNAL ID=\"sig60\">\n        <ho:SHORT-NAME>Cell_I_6</ho:SHORT-NAME>\n        <fx:DEFAULT-VALUE>0</fx:DEFAULT-VALUE>\n        <fx:CODING-REF ID-REF=\"cod60\"/>\n      </fx:SIGNAL>\n      <fx:SIGNAL ID=\"sig61\">\n        <ho:SHORT-NAME>Cell_I_7</ho:SHORT-NAME>\n        <fx:DEFAULT-VALUE>0</fx:DEFAULT-VALUE>\n        <fx:CODING-REF ID-REF=\"cod61\"/>\n      </fx:SIGNAL>\n      <fx:SIGNAL ID=\"sig62\">\n        <ho:SHORT-NAME>Cell_I_8</ho:SHORT-NAME>\n        <fx:DEFAULT-VALUE>0</fx:DEFAULT-VALUE>\n        <fx:CODING-REF ID-REF=\"cod62\"/>\n      </fx:SIGNAL>\n      <fx:SIGNAL ID=\"sig63\">\n        <ho:SHORT-NAME>Cell_I_09</ho:SHORT-NAME>\n        <fx:DEFAULT-VALUE>0</fx:DEFAULT-VALUE>\n        <fx:CODING-REF ID-REF=\"cod63\"/>\n      </fx:SIGNAL>\n      <fx:SIGNAL ID=\"sig64\">\n        <ho:SHORT-NAME>Cell_I_10</ho:SHORT-NAME>\n        <fx:DEFAULT-VALUE>0</fx:DEFAULT-VALUE>\n        <fx:CODING-REF ID-REF=\"cod64\"/>\n      </fx:SIGNAL>\n      <fx:SIGNAL ID=\"sig65\">\n        <ho:SHORT-NAME>Cell_I_11</ho:SHORT-NAME>\n        <fx:DEFAULT-VALUE>0</fx:DEFAULT-VALUE>\n        <fx:CODING-REF ID-REF=\"cod65\"/>\n      </fx:SIGNAL>\n      <fx:SIGNAL ID=\"sig66\">\n        <ho:SHORT-NAME>Cell_I_12</ho:SHORT-NAME>\n        <fx:DEFAULT-VALUE>0</fx:DEFAULT-VALUE>\n        <fx:CODING-REF ID-REF=\"cod66\"/>\n      </fx:SIGNAL>\n      <fx:SIGNAL ID=\"sig67\">\n        <ho:SHORT-NAME>DIO_1_8</ho:SHORT-NAME>\n        <fx:DEFAULT-VALUE>0</fx:DEFAULT-VALUE>\n        <fx:CODING-REF ID-REF=\"cod67\"/>\n      </fx:SIGNAL>\n      <fx:SIGNAL ID=\"sig68\">\n        <ho:SHORT-NAME>AI_1</ho:SHORT-NAME>\n        <fx:DEFAULT-VALUE>0</fx:DEFAULT-VALUE>\n        <fx:CODING-REF ID-REF=\"cod68\"/>\n      </fx:SIGNAL>\n      <fx:SIGNAL ID=\"sig69\">\n        <ho:SHORT-NAME>AI_2</ho:SHORT-NAME>\n        <fx:DEFAULT-VALUE>0</fx:DEFAULT-VALUE>\n        <fx:CODING-REF ID-REF=\"cod69\"/>\n      </fx:SIGNAL>\n      <fx:SIGNAL ID=\"sig70\">\n        <ho:SHORT-NAME>AI_3</ho:SHORT-NAME>\n        <fx:DEFAULT-VALUE>0</fx:DEFAULT-VALUE>\n        <fx:CODING-REF ID-REF=\"cod70\"/>\n      </fx:SIGNAL>\n      <fx:SIGNAL ID=\"sig71\">\n        <ho:SHORT-NAME>AI_4</ho:SHORT-NAME>\n        <fx:DEFAULT-VALUE>0</fx:DEFAULT-VALUE>\n        <fx:CODING-REF ID-REF=\"cod71\"/>\n      </fx:SIGNAL>\n      <fx:SIGNAL ID=\"sig72\">\n        <ho:SHORT-NAME>AI_5</ho:SHORT-NAME>\n        <fx:DEFAULT-VALUE>0</fx:DEFAULT-VALUE>\n        <fx:CODING-REF ID-REF=\"cod72\"/>\n      </fx:SIGNAL>\n      <fx:SIGNAL ID=\"sig73\">\n        <ho:SHORT-NAME>AI_6</ho:SHORT-NAME>\n        <fx:DEFAULT-VALUE>0</fx:DEFAULT-VALUE>\n        <fx:CODING-REF ID-REF=\"cod73\"/>\n      </fx:SIGNAL>\n      <fx:SIGNAL ID=\"sig74\">\n        <ho:SHORT-NAME>AI_7</ho:SHORT-NAME>\n        <fx:DEFAULT-VALUE>0</fx:DEFAULT-VALUE>\n        <fx:CODING-REF ID-REF=\"cod74\"/>\n      </fx:SIGNAL>\n      <fx:SIGNAL ID=\"sig75\">\n        <ho:SHORT-NAME>AI_8</ho:SHORT-NAME>\n        <fx:DEFAULT-VALUE>0</fx:DEFAULT-VALUE>\n        <fx:CODING-REF ID-REF=\"cod75\"/>\n      </fx:SIGNAL>\n    </fx:SIGNALS>\n  </fx:ELEMENTS>\n  <fx:PROCESSING-INFORMATION xmlns=\"http://www.asam.net/xml\">\n    <ho:UNIT-SPEC>\n      <ho:UNITS>\n        <ho:UNIT ID=\"unit1\">\n          <ho:SHORT-NAME>unit1</ho:SHORT-NAME>\n          <ho:DISPLAY-NAME></ho:DISPLAY-NAME>\n        </ho:UNIT>\n        <ho:UNIT ID=\"unit2\">\n          <ho:SHORT-NAME>unit2</ho:SHORT-NAME>\n          <ho:DISPLAY-NAME>V</ho:DISPLAY-NAME>\n        </ho:UNIT>\n        <ho:UNIT ID=\"unit3\">\n          <ho:SHORT-NAME>unit3</ho:SHORT-NAME>\n          <ho:DISPLAY-NAME>V</ho:DISPLAY-NAME>\n        </ho:UNIT>\n        <ho:UNIT ID=\"unit4\">\n          <ho:SHORT-NAME>unit4</ho:SHORT-NAME>\n          <ho:DISPLAY-NAME>V</ho:DISPLAY-NAME>\n        </ho:UNIT>\n        <ho:UNIT ID=\"unit5\">\n          <ho:SHORT-NAME>unit5</ho:SHORT-NAME>\n          <ho:DISPLAY-NAME>V</ho:DISPLAY-NAME>\n        </ho:UNIT>\n        <ho:UNIT ID=\"unit6\">\n          <ho:SHORT-NAME>unit6</ho:SHORT-NAME>\n          <ho:DISPLAY-NAME></ho:DISPLAY-NAME>\n        </ho:UNIT>\n        <ho:UNIT ID=\"unit7\">\n          <ho:SHORT-NAME>unit7</ho:SHORT-NAME>\n          <ho:DISPLAY-NAME>mA</ho:DISPLAY-NAME>\n        </ho:UNIT>\n        <ho:UNIT ID=\"unit8\">\n          <ho:SHORT-NAME>unit8</ho:SHORT-NAME>\n          <ho:DISPLAY-NAME>V</ho:DISPLAY-NAME>\n        </ho:UNIT>\n        <ho:UNIT ID=\"unit9\">\n          <ho:SHORT-NAME>unit9</ho:SHORT-NAME>\n          <ho:DISPLAY-NAME></ho:DISPLAY-NAME>\n        </ho:UNIT>\n        <ho:UNIT ID=\"unit10\">\n          <ho:SHORT-NAME>unit10</ho:SHORT-NAME>\n          <ho:DISPLAY-NAME></ho:DISPLAY-NAME>\n        </ho:UNIT>\n        <ho:UNIT ID=\"unit11\">\n          <ho:SHORT-NAME>unit11</ho:SHORT-NAME>\n          <ho:DISPLAY-NAME>V</ho:DISPLAY-NAME>\n        </ho:UNIT>\n        <ho:UNIT ID=\"unit12\">\n          <ho:SHORT-NAME>unit12</ho:SHORT-NAME>\n          <ho:DISPLAY-NAME>V</ho:DISPLAY-NAME>\n        </ho:UNIT>\n        <ho:UNIT ID=\"unit13\">\n          <ho:SHORT-NAME>unit13</ho:SHORT-NAME>\n          <ho:DISPLAY-NAME></ho:DISPLAY-NAME>\n        </ho:UNIT>\n        <ho:UNIT ID=\"unit14\">\n          <ho:SHORT-NAME>unit14</ho:SHORT-NAME>\n          <ho:DISPLAY-NAME></ho:DISPLAY-NAME>\n        </ho:UNIT>\n        <ho:UNIT ID=\"unit15\">\n          <ho:SHORT-NAME>unit15</ho:SHORT-NAME>\n          <ho:DISPLAY-NAME></ho:DISPLAY-NAME>\n        </ho:UNIT>\n        <ho:UNIT ID=\"unit16\">\n          <ho:SHORT-NAME>unit16</ho:SHORT-NAME>\n          <ho:DISPLAY-NAME></ho:DISPLAY-NAME>\n        </ho:UNIT>\n        <ho:UNIT ID=\"unit17\">\n          <ho:SHORT-NAME>unit17</ho:SHORT-NAME>\n          <ho:DISPLAY-NAME></ho:DISPLAY-NAME>\n        </ho:UNIT>\n        <ho:UNIT ID=\"unit18\">\n          <ho:SHORT-NAME>unit18</ho:SHORT-NAME>\n          <ho:DISPLAY-NAME></ho:DISPLAY-NAME>\n        </ho:UNIT>\n        <ho:UNIT ID=\"unit19\">\n          <ho:SHORT-NAME>unit19</ho:SHORT-NAME>\n          <ho:DISPLAY-NAME>mA</ho:DISPLAY-NAME>\n        </ho:UNIT>\n        <ho:UNIT ID=\"unit20\">\n          <ho:SHORT-NAME>unit20</ho:SHORT-NAME>\n          <ho:DISPLAY-NAME>mA</ho:DISPLAY-NAME>\n        </ho:UNIT>\n        <ho:UNIT ID=\"unit21\">\n          <ho:SHORT-NAME>unit21</ho:SHORT-NAME>\n          <ho:DISPLAY-NAME></ho:DISPLAY-NAME>\n        </ho:UNIT>\n        <ho:UNIT ID=\"unit22\">\n          <ho:SHORT-NAME>unit22</ho:SHORT-NAME>\n          <ho:DISPLAY-NAME>mA</ho:DISPLAY-NAME>\n        </ho:UNIT>\n        <ho:UNIT ID=\"unit23\">\n          <ho:SHORT-NAME>unit23</ho:SHORT-NAME>\n          <ho:DISPLAY-NAME></ho:DISPLAY-NAME>\n        </ho:UNIT>\n        <ho:UNIT ID=\"unit24\">\n          <ho:SHORT-NAME>unit24</ho:SHORT-NAME>\n          <ho:DISPLAY-NAME>V</ho:DISPLAY-NAME>\n        </ho:UNIT>\n        <ho:UNIT ID=\"unit25\">\n          <ho:SHORT-NAME>unit25</ho:SHORT-NAME>\n          <ho:DISPLAY-NAME>V</ho:DISPLAY-NAME>\n        </ho:UNIT>\n        <ho:UNIT ID=\"unit26\">\n          <ho:SHORT-NAME>unit26</ho:SHORT-NAME>\n          <ho:DISPLAY-NAME>V</ho:DISPLAY-NAME>\n        </ho:UNIT>\n        <ho:UNIT ID=\"unit27\">\n          <ho:SHORT-NAME>unit27</ho:SHORT-NAME>\n          <ho:DISPLAY-NAME>V</ho:DISPLAY-NAME>\n        </ho:UNIT>\n        <ho:UNIT ID=\"unit28\">\n          <ho:SHORT-NAME>unit28</ho:SHORT-NAME>\n          <ho:DISPLAY-NAME>V</ho:DISPLAY-NAME>\n        </ho:UNIT>\n        <ho:UNIT ID=\"unit29\">\n          <ho:SHORT-NAME>unit29</ho:SHORT-NAME>\n          <ho:DISPLAY-NAME>mA</ho:DISPLAY-NAME>\n        </ho:UNIT>\n        <ho:UNIT ID=\"unit30\">\n          <ho:SHORT-NAME>unit30</ho:SHORT-NAME>\n          <ho:DISPLAY-NAME>mA</ho:DISPLAY-NAME>\n        </ho:UNIT>\n        <ho:UNIT ID=\"unit31\">\n          <ho:SHORT-NAME>unit31</ho:SHORT-NAME>\n          <ho:DISPLAY-NAME>mA</ho:DISPLAY-NAME>\n        </ho:UNIT>\n        <ho:UNIT ID=\"unit32\">\n          <ho:SHORT-NAME>unit32</ho:SHORT-NAME>\n          <ho:DISPLAY-NAME>mA</ho:DISPLAY-NAME>\n        </ho:UNIT>\n        <ho:UNIT ID=\"unit33\">\n          <ho:SHORT-NAME>unit33</ho:SHORT-NAME>\n          <ho:DISPLAY-NAME></ho:DISPLAY-NAME>\n        </ho:UNIT>\n        <ho:UNIT ID=\"unit34\">\n          <ho:SHORT-NAME>unit34</ho:SHORT-NAME>\n          <ho:DISPLAY-NAME></ho:DISPLAY-NAME>\n        </ho:UNIT>\n        <ho:UNIT ID=\"unit35\">\n          <ho:SHORT-NAME>unit35</ho:SHORT-NAME>\n          <ho:DISPLAY-NAME></ho:DISPLAY-NAME>\n        </ho:UNIT>\n        <ho:UNIT ID=\"unit36\">\n          <ho:SHORT-NAME>unit36</ho:SHORT-NAME>\n          <ho:DISPLAY-NAME>Degrees C</ho:DISPLAY-NAME>\n        </ho:UNIT>\n        <ho:UNIT ID=\"unit37\">\n          <ho:SHORT-NAME>unit37</ho:SHORT-NAME>\n          <ho:DISPLAY-NAME>Degrees C</ho:DISPLAY-NAME>\n        </ho:UNIT>\n        <ho:UNIT ID=\"unit38\">\n          <ho:SHORT-NAME>unit38</ho:SHORT-NAME>\n          <ho:DISPLAY-NAME>Degrees C</ho:DISPLAY-NAME>\n        </ho:UNIT>\n        <ho:UNIT ID=\"unit39\">\n          <ho:SHORT-NAME>unit39</ho:SHORT-NAME>\n          <ho:DISPLAY-NAME></ho:DISPLAY-NAME>\n        </ho:UNIT>\n        <ho:UNIT ID=\"unit40\">\n          <ho:SHORT-NAME>unit40</ho:SHORT-NAME>\n          <ho:DISPLAY-NAME></ho:DISPLAY-NAME>\n        </ho:UNIT>\n        <ho:UNIT ID=\"unit41\">\n          <ho:SHORT-NAME>unit41</ho:SHORT-NAME>\n          <ho:DISPLAY-NAME></ho:DISPLAY-NAME>\n        </ho:UNIT>\n        <ho:UNIT ID=\"unit42\">\n          <ho:SHORT-NAME>unit42</ho:SHORT-NAME>\n          <ho:DISPLAY-NAME></ho:DISPLAY-NAME>\n        </ho:UNIT>\n        <ho:UNIT ID=\"unit43\">\n          <ho:SHORT-NAME>unit43</ho:SHORT-NAME>\n          <ho:DISPLAY-NAME>V</ho:DISPLAY-NAME>\n        </ho:UNIT>\n        <ho:UNIT ID=\"unit44\">\n          <ho:SHORT-NAME>unit44</ho:SHORT-NAME>\n          <ho:DISPLAY-NAME>V</ho:DISPLAY-NAME>\n        </ho:UNIT>\n        <ho:UNIT ID=\"unit45\">\n          <ho:SHORT-NAME>unit45</ho:SHORT-NAME>\n          <ho:DISPLAY-NAME>V</ho:DISPLAY-NAME>\n        </ho:UNIT>\n        <ho:UNIT ID=\"unit46\">\n          <ho:SHORT-NAME>unit46</ho:SHORT-NAME>\n          <ho:DISPLAY-NAME>V</ho:DISPLAY-NAME>\n        </ho:UNIT>\n        <ho:UNIT ID=\"unit47\">\n          <ho:SHORT-NAME>unit47</ho:SHORT-NAME>\n          <ho:DISPLAY-NAME>V</ho:DISPLAY-NAME>\n        </ho:UNIT>\n        <ho:UNIT ID=\"unit48\">\n          <ho:SHORT-NAME>unit48</ho:SHORT-NAME>\n          <ho:DISPLAY-NAME>V</ho:DISPLAY-NAME>\n        </ho:UNIT>\n        <ho:UNIT ID=\"unit49\">\n          <ho:SHORT-NAME>unit49</ho:SHORT-NAME>\n          <ho:DISPLAY-NAME>V</ho:DISPLAY-NAME>\n        </ho:UNIT>\n        <ho:UNIT ID=\"unit50\">\n          <ho:SHORT-NAME>unit50</ho:SHORT-NAME>\n          <ho:DISPLAY-NAME>V</ho:DISPLAY-NAME>\n        </ho:UNIT>\n        <ho:UNIT ID=\"unit51\">\n          <ho:SHORT-NAME>unit51</ho:SHORT-NAME>\n          <ho:DISPLAY-NAME>V</ho:DISPLAY-NAME>\n        </ho:UNIT>\n        <ho:UNIT ID=\"unit52\">\n          <ho:SHORT-NAME>unit52</ho:SHORT-NAME>\n          <ho:DISPLAY-NAME>V</ho:DISPLAY-NAME>\n        </ho:UNIT>\n        <ho:UNIT ID=\"unit53\">\n          <ho:SHORT-NAME>unit53</ho:SHORT-NAME>\n          <ho:DISPLAY-NAME>V</ho:DISPLAY-NAME>\n        </ho:UNIT>\n        <ho:UNIT ID=\"unit54\">\n          <ho:SHORT-NAME>unit54</ho:SHORT-NAME>\n          <ho:DISPLAY-NAME></ho:DISPLAY-NAME>\n        </ho:UNIT>\n        <ho:UNIT ID=\"unit55\">\n          <ho:SHORT-NAME>unit55</ho:SHORT-NAME>\n          <ho:DISPLAY-NAME>V</ho:DISPLAY-NAME>\n        </ho:UNIT>\n        <ho:UNIT ID=\"unit56\">\n          <ho:SHORT-NAME>unit56</ho:SHORT-NAME>\n          <ho:DISPLAY-NAME>V</ho:DISPLAY-NAME>\n        </ho:UNIT>\n        <ho:UNIT ID=\"unit57\">\n          <ho:SHORT-NAME>unit57</ho:SHORT-NAME>\n          <ho:DISPLAY-NAME>V</ho:DISPLAY-NAME>\n        </ho:UNIT>\n        <ho:UNIT ID=\"unit58\">\n          <ho:SHORT-NAME>unit58</ho:SHORT-NAME>\n          <ho:DISPLAY-NAME>V</ho:DISPLAY-NAME>\n        </ho:UNIT>\n        <ho:UNIT ID=\"unit59\">\n          <ho:SHORT-NAME>unit59</ho:SHORT-NAME>\n          <ho:DISPLAY-NAME>mA</ho:DISPLAY-NAME>\n        </ho:UNIT>\n        <ho:UNIT ID=\"unit60\">\n          <ho:SHORT-NAME>unit60</ho:SHORT-NAME>\n          <ho:DISPLAY-NAME>mA</ho:DISPLAY-NAME>\n        </ho:UNIT>\n        <ho:UNIT ID=\"unit61\">\n          <ho:SHORT-NAME>unit61</ho:SHORT-NAME>\n          <ho:DISPLAY-NAME>mA</ho:DISPLAY-NAME>\n        </ho:UNIT>\n        <ho:UNIT ID=\"unit62\">\n          <ho:SHORT-NAME>unit62</ho:SHORT-NAME>\n          <ho:DISPLAY-NAME>mA</ho:DISPLAY-NAME>\n        </ho:UNIT>\n        <ho:UNIT ID=\"unit63\">\n          <ho:SHORT-NAME>unit63</ho:SHORT-NAME>\n          <ho:DISPLAY-NAME>mA</ho:DISPLAY-NAME>\n        </ho:UNIT>\n        <ho:UNIT ID=\"unit64\">\n          <ho:SHORT-NAME>unit64</ho:SHORT-NAME>\n          <ho:DISPLAY-NAME>mA</ho:DISPLAY-NAME>\n        </ho:UNIT>\n        <ho:UNIT ID=\"unit65\">\n          <ho:SHORT-NAME>unit65</ho:SHORT-NAME>\n          <ho:DISPLAY-NAME>mA</ho:DISPLAY-NAME>\n        </ho:UNIT>\n        <ho:UNIT ID=\"unit66\">\n          <ho:SHORT-NAME>unit66</ho:SHORT-NAME>\n          <ho:DISPLAY-NAME>mA</ho:DISPLAY-NAME>\n        </ho:UNIT>\n        <ho:UNIT ID=\"unit67\">\n          <ho:SHORT-NAME>unit67</ho:SHORT-NAME>\n          <ho:DISPLAY-NAME></ho:DISPLAY-NAME>\n        </ho:UNIT>\n        <ho:UNIT ID=\"unit68\">\n          <ho:SHORT-NAME>unit68</ho:SHORT-NAME>\n          <ho:DISPLAY-NAME>V</ho:DISPLAY-NAME>\n        </ho:UNIT>\n        <ho:UNIT ID=\"unit69\">\n          <ho:SHORT-NAME>unit69</ho:SHORT-NAME>\n          <ho:DISPLAY-NAME>V</ho:DISPLAY-NAME>\n        </ho:UNIT>\n        <ho:UNIT ID=\"unit70\">\n          <ho:SHORT-NAME>unit70</ho:SHORT-NAME>\n          <ho:DISPLAY-NAME>V</ho:DISPLAY-NAME>\n        </ho:UNIT>\n        <ho:UNIT ID=\"unit71\">\n          <ho:SHORT-NAME>unit71</ho:SHORT-NAME>\n          <ho:DISPLAY-NAME>V</ho:DISPLAY-NAME>\n        </ho:UNIT>\n        <ho:UNIT ID=\"unit72\">\n          <ho:SHORT-NAME>unit72</ho:SHORT-NAME>\n          <ho:DISPLAY-NAME>V</ho:DISPLAY-NAME>\n        </ho:UNIT>\n        <ho:UNIT ID=\"unit73\">\n          <ho:SHORT-NAME>unit73</ho:SHORT-NAME>\n          <ho:DISPLAY-NAME>V</ho:DISPLAY-NAME>\n        </ho:UNIT>\n        <ho:UNIT ID=\"unit74\">\n          <ho:SHORT-NAME>unit74</ho:SHORT-NAME>\n          <ho:DISPLAY-NAME>V</ho:DISPLAY-NAME>\n        </ho:UNIT>\n        <ho:UNIT ID=\"unit75\">\n          <ho:SHORT-NAME>unit75</ho:SHORT-NAME>\n          <ho:DISPLAY-NAME>V</ho:DISPLAY-NAME>\n        </ho:UNIT>\n      </ho:UNITS>\n    </ho:UNIT-SPEC>\n    <fx:CODINGS>\n      <fx:CODING ID=\"cod1\">\n        <ho:SHORT-NAME>cod1</ho:SHORT-NAME>\n        <ho:CODED-TYPE ho:BASE-DATA-TYPE=\"A_UINT8\" CATEGORY=\"STANDARD-LENGTH-TYPE\" ENCODING=\"UNSIGNED\">\n          <ho:BIT-LENGTH>1</ho:BIT-LENGTH>\n        </ho:CODED-TYPE>\n        <ho:COMPU-METHODS>\n          <ho:COMPU-METHOD>\n            <ho:SHORT-NAME>cpm1</ho:SHORT-NAME>\n            <ho:CATEGORY>LINEAR</ho:CATEGORY>\n            <ho:UNIT-REF ID-REF=\"unit1\"/>\n            <ho:PHYS-CONSTRS>\n              <ho:SCALE-CONSTR>\n                <ho:LOWER-LIMIT INTERVAL-TYPE=\"CLOSED\">0</ho:LOWER-LIMIT>\n                <ho:UPPER-LIMIT INTERVAL-TYPE=\"CLOSED\">1000</ho:UPPER-LIMIT>\n              </ho:SCALE-CONSTR>\n            </ho:PHYS-CONSTRS>\n            <ho:COMPU-INTERNAL-TO-PHYS>\n              <ho:COMPU-SCALES>\n                <ho:COMPU-SCALE>\n                  <ho:COMPU-RATIONAL-COEFFS>\n                    <ho:COMPU-NUMERATOR>\n                      <ho:V>0</ho:V>\n                      <ho:V>1</ho:V>\n                    </ho:COMPU-NUMERATOR>\n                    <ho:COMPU-DENOMINATOR>\n                      <ho:V>1</ho:V>\n                    </ho:COMPU-DENOMINATOR>\n                  </ho:COMPU-RATIONAL-COEFFS>\n                </ho:COMPU-SCALE>\n              </ho:COMPU-SCALES>\n            </ho:COMPU-INTERNAL-TO-PHYS>\n          </ho:COMPU-METHOD>\n        </ho:COMPU-METHODS>\n      </fx:CODING>\n      <fx:CODING ID=\"cod2\">\n        <ho:SHORT-NAME>cod2</ho:SHORT-NAME>\n        <ho:CODED-TYPE ho:BASE-DATA-TYPE=\"A_UINT16\" CATEGORY=\"STANDARD-LENGTH-TYPE\" ENCODING=\"UNSIGNED\">\n          <ho:BIT-LENGTH>16</ho:BIT-LENGTH>\n        </ho:CODED-TYPE>\n        <ho:COMPU-METHODS>\n          <ho:COMPU-METHOD>\n            <ho:SHORT-NAME>cpm2</ho:SHORT-NAME>\n            <ho:CATEGORY>LINEAR</ho:CATEGORY>\n            <ho:UNIT-REF ID-REF=\"unit2\"/>\n            <ho:PHYS-CONSTRS>\n              <ho:SCALE-CONSTR>\n                <ho:LOWER-LIMIT INTERVAL-TYPE=\"CLOSED\">0</ho:LOWER-LIMIT>\n                <ho:UPPER-LIMIT INTERVAL-TYPE=\"CLOSED\">5</ho:UPPER-LIMIT>\n              </ho:SCALE-CONSTR>\n            </ho:PHYS-CONSTRS>\n            <ho:COMPU-INTERNAL-TO-PHYS>\n              <ho:COMPU-SCALES>\n                <ho:COMPU-SCALE>\n                  <ho:COMPU-RATIONAL-COEFFS>\n                    <ho:COMPU-NUMERATOR>\n                      <ho:V>0</ho:V>\n                      <ho:V>1</ho:V>\n                    </ho:COMPU-NUMERATOR>\n                    <ho:COMPU-DENOMINATOR>\n                      <ho:V>1</ho:V>\n                    </ho:COMPU-DENOMINATOR>\n                  </ho:COMPU-RATIONAL-COEFFS>\n                </ho:COMPU-SCALE>\n              </ho:COMPU-SCALES>\n            </ho:COMPU-INTERNAL-TO-PHYS>\n          </ho:COMPU-METHOD>\n        </ho:COMPU-METHODS>\n      </fx:CODING>\n      <fx:CODING ID=\"cod3\">\n        <ho:SHORT-NAME>cod3</ho:SHORT-NAME>\n        <ho:CODED-TYPE ho:BASE-DATA-TYPE=\"A_UINT16\" CATEGORY=\"STANDARD-LENGTH-TYPE\" ENCODING=\"UNSIGNED\">\n          <ho:BIT-LENGTH>16</ho:BIT-LENGTH>\n        </ho:CODED-TYPE>\n        <ho:COMPU-METHODS>\n          <ho:COMPU-METHOD>\n            <ho:SHORT-NAME>cpm3</ho:SHORT-NAME>\n            <ho:CATEGORY>LINEAR</ho:CATEGORY>\n            <ho:UNIT-REF ID-REF=\"unit3\"/>\n            <ho:PHYS-CONSTRS>\n              <ho:SCALE-CONSTR>\n                <ho:LOWER-LIMIT INTERVAL-TYPE=\"CLOSED\">0</ho:LOWER-LIMIT>\n                <ho:UPPER-LIMIT INTERVAL-TYPE=\"CLOSED\">5</ho:UPPER-LIMIT>\n              </ho:SCALE-CONSTR>\n            </ho:PHYS-CONSTRS>\n            <ho:COMPU-INTERNAL-TO-PHYS>\n              <ho:COMPU-SCALES>\n                <ho:COMPU-SCALE>\n                  <ho:COMPU-RATIONAL-COEFFS>\n                    <ho:COMPU-NUMERATOR>\n                      <ho:V>0</ho:V>\n                      <ho:V>1</ho:V>\n                    </ho:COMPU-NUMERATOR>\n                    <ho:COMPU-DENOMINATOR>\n                      <ho:V>1</ho:V>\n                    </ho:COMPU-DENOMINATOR>\n                  </ho:COMPU-RATIONAL-COEFFS>\n                </ho:COMPU-SCALE>\n              </ho:COMPU-SCALES>\n            </ho:COMPU-INTERNAL-TO-PHYS>\n          </ho:COMPU-METHOD>\n        </ho:COMPU-METHODS>\n      </fx:CODING>\n      <fx:CODING ID=\"cod4\">\n        <ho:SHORT-NAME>cod4</ho:SHORT-NAME>\n        <ho:CODED-TYPE ho:BASE-DATA-TYPE=\"A_UINT16\" CATEGORY=\"STANDARD-LENGTH-TYPE\" ENCODING=\"UNSIGNED\">\n          <ho:BIT-LENGTH>16</ho:BIT-LENGTH>\n        </ho:CODED-TYPE>\n        <ho:COMPU-METHODS>\n          <ho:COMPU-METHOD>\n            <ho:SHORT-NAME>cpm4</ho:SHORT-NAME>\n            <ho:CATEGORY>LINEAR</ho:CATEGORY>\n            <ho:UNIT-REF ID-REF=\"unit4\"/>\n            <ho:PHYS-CONSTRS>\n              <ho:SCALE-CONSTR>\n                <ho:LOWER-LIMIT INTERVAL-TYPE=\"CLOSED\">0</ho:LOWER-LIMIT>\n                <ho:UPPER-LIMIT INTERVAL-TYPE=\"CLOSED\">5</ho:UPPER-LIMIT>\n              </ho:SCALE-CONSTR>\n            </ho:PHYS-CONSTRS>\n            <ho:COMPU-INTERNAL-TO-PHYS>\n              <ho:COMPU-SCALES>\n                <ho:COMPU-SCALE>\n                  <ho:COMPU-RATIONAL-COEFFS>\n                    <ho:COMPU-NUMERATOR>\n                      <ho:V>0</ho:V>\n                      <ho:V>1</ho:V>\n                    </ho:COMPU-NUMERATOR>\n                    <ho:COMPU-DENOMINATOR>\n                      <ho:V>1</ho:V>\n                    </ho:COMPU-DENOMINATOR>\n                  </ho:COMPU-RATIONAL-COEFFS>\n                </ho:COMPU-SCALE>\n              </ho:COMPU-SCALES>\n            </ho:COMPU-INTERNAL-TO-PHYS>\n          </ho:COMPU-METHOD>\n        </ho:COMPU-METHODS>\n      </fx:CODING>\n      <fx:CODING ID=\"cod5\">\n        <ho:SHORT-NAME>cod5</ho:SHORT-NAME>\n        <ho:CODED-TYPE ho:BASE-DATA-TYPE=\"A_UINT16\" CATEGORY=\"STANDARD-LENGTH-TYPE\" ENCODING=\"UNSIGNED\">\n          <ho:BIT-LENGTH>16</ho:BIT-LENGTH>\n        </ho:CODED-TYPE>\n        <ho:COMPU-METHODS>\n          <ho:COMPU-METHOD>\n            <ho:SHORT-NAME>cpm5</ho:SHORT-NAME>\n            <ho:CATEGORY>LINEAR</ho:CATEGORY>\n            <ho:UNIT-REF ID-REF=\"unit5\"/>\n            <ho:PHYS-CONSTRS>\n              <ho:SCALE-CONSTR>\n                <ho:LOWER-LIMIT INTERVAL-TYPE=\"CLOSED\">0</ho:LOWER-LIMIT>\n                <ho:UPPER-LIMIT INTERVAL-TYPE=\"CLOSED\">5</ho:UPPER-LIMIT>\n              </ho:SCALE-CONSTR>\n            </ho:PHYS-CONSTRS>\n            <ho:COMPU-INTERNAL-TO-PHYS>\n              <ho:COMPU-SCALES>\n                <ho:COMPU-SCALE>\n                  <ho:COMPU-RATIONAL-COEFFS>\n                    <ho:COMPU-NUMERATOR>\n                      <ho:V>0</ho:V>\n                      <ho:V>1</ho:V>\n                    </ho:COMPU-NUMERATOR>\n                    <ho:COMPU-DENOMINATOR>\n                      <ho:V>1</ho:V>\n                    </ho:COMPU-DENOMINATOR>\n                  </ho:COMPU-RATIONAL-COEFFS>\n                </ho:COMPU-SCALE>\n              </ho:COMPU-SCALES>\n            </ho:COMPU-INTERNAL-TO-PHYS>\n          </ho:COMPU-METHOD>\n        </ho:COMPU-METHODS>\n      </fx:CODING>\n      <fx:CODING ID=\"cod6\">\n        <ho:SHORT-NAME>cod6</ho:SHORT-NAME>\n        <ho:CODED-TYPE ho:BASE-DATA-TYPE=\"A_UINT8\" CATEGORY=\"STANDARD-LENGTH-TYPE\" ENCODING=\"UNSIGNED\">\n          <ho:BIT-LENGTH>8</ho:BIT-LENGTH>\n        </ho:CODED-TYPE>\n        <ho:COMPU-METHODS>\n          <ho:COMPU-METHOD>\n            <ho:SHORT-NAME>cpm6</ho:SHORT-NAME>\n            <ho:CATEGORY>LINEAR</ho:CATEGORY>\n            <ho:UNIT-REF ID-REF=\"unit6\"/>\n            <ho:PHYS-CONSTRS>\n              <ho:SCALE-CONSTR>\n                <ho:LOWER-LIMIT INTERVAL-TYPE=\"CLOSED\">1</ho:LOWER-LIMIT>\n                <ho:UPPER-LIMIT INTERVAL-TYPE=\"CLOSED\">12</ho:UPPER-LIMIT>\n              </ho:SCALE-CONSTR>\n            </ho:PHYS-CONSTRS>\n            <ho:COMPU-INTERNAL-TO-PHYS>\n              <ho:COMPU-SCALES>\n                <ho:COMPU-SCALE>\n                  <ho:COMPU-RATIONAL-COEFFS>\n                    <ho:COMPU-NUMERATOR>\n                      <ho:V>1</ho:V>\n                      <ho:V>1</ho:V>\n                    </ho:COMPU-NUMERATOR>\n                    <ho:COMPU-DENOMINATOR>\n                      <ho:V>1</ho:V>\n                    </ho:COMPU-DENOMINATOR>\n                  </ho:COMPU-RATIONAL-COEFFS>\n                </ho:COMPU-SCALE>\n              </ho:COMPU-SCALES>\n            </ho:COMPU-INTERNAL-TO-PHYS>\n          </ho:COMPU-METHOD>\n        </ho:COMPU-METHODS>\n      </fx:CODING>\n      <fx:CODING ID=\"cod7\">\n        <ho:SHORT-NAME>cod7</ho:SHORT-NAME>\n        <ho:CODED-TYPE ho:BASE-DATA-TYPE=\"A_UINT16\" CATEGORY=\"STANDARD-LENGTH-TYPE\" ENCODING=\"UNSIGNED\">\n          <ho:BIT-LENGTH>16</ho:BIT-LENGTH>\n        </ho:CODED-TYPE>\n        <ho:COMPU-METHODS>\n          <ho:COMPU-METHOD>\n            <ho:SHORT-NAME>cpm7</ho:SHORT-NAME>\n            <ho:CATEGORY>LINEAR</ho:CATEGORY>\n            <ho:UNIT-REF ID-REF=\"unit7\"/>\n            <ho:PHYS-CONSTRS>\n              <ho:SCALE-CONSTR>\n                <ho:LOWER-LIMIT INTERVAL-TYPE=\"CLOSED\">0</ho:LOWER-LIMIT>\n                <ho:UPPER-LIMIT INTERVAL-TYPE=\"CLOSED\">500.0000000000001</ho:UPPER-LIMIT>\n              </ho:SCALE-CONSTR>\n            </ho:PHYS-CONSTRS>\n            <ho:COMPU-INTERNAL-TO-PHYS>\n              <ho:COMPU-SCALES>\n                <ho:COMPU-SCALE>\n                  <ho:COMPU-RATIONAL-COEFFS>\n                    <ho:COMPU-NUMERATOR>\n                      <ho:V>0</ho:V>\n                      <ho:V>1</ho:V>\n                    </ho:COMPU-NUMERATOR>\n                    <ho:COMPU-DENOMINATOR>\n                      <ho:V>1</ho:V>\n                    </ho:COMPU-DENOMINATOR>\n                  </ho:COMPU-RATIONAL-COEFFS>\n                </ho:COMPU-SCALE>\n              </ho:COMPU-SCALES>\n            </ho:COMPU-INTERNAL-TO-PHYS>\n          </ho:COMPU-METHOD>\n        </ho:COMPU-METHODS>\n      </fx:CODING>\n      <fx:CODING ID=\"cod8\">\n        <ho:SHORT-NAME>cod8</ho:SHORT-NAME>\n        <ho:CODED-TYPE ho:BASE-DATA-TYPE=\"A_UINT16\" CATEGORY=\"STANDARD-LENGTH-TYPE\" ENCODING=\"UNSIGNED\">\n          <ho:BIT-LENGTH>16</ho:BIT-LENGTH>\n        </ho:CODED-TYPE>\n        <ho:COMPU-METHODS>\n          <ho:COMPU-METHOD>\n            <ho:SHORT-NAME>cpm8</ho:SHORT-NAME>\n            <ho:CATEGORY>LINEAR</ho:CATEGORY>\n            <ho:UNIT-REF ID-REF=\"unit8\"/>\n            <ho:PHYS-CONSTRS>\n              <ho:SCALE-CONSTR>\n                <ho:LOWER-LIMIT INTERVAL-TYPE=\"CLOSED\">0</ho:LOWER-LIMIT>\n                <ho:UPPER-LIMIT INTERVAL-TYPE=\"CLOSED\">5</ho:UPPER-LIMIT>\n              </ho:SCALE-CONSTR>\n            </ho:PHYS-CONSTRS>\n            <ho:COMPU-INTERNAL-TO-PHYS>\n              <ho:COMPU-SCALES>\n                <ho:COMPU-SCALE>\n                  <ho:COMPU-RATIONAL-COEFFS>\n                    <ho:COMPU-NUMERATOR>\n                      <ho:V>0</ho:V>\n                      <ho:V>1</ho:V>\n                    </ho:COMPU-NUMERATOR>\n                    <ho:COMPU-DENOMINATOR>\n                      <ho:V>1</ho:V>\n                    </ho:COMPU-DENOMINATOR>\n                  </ho:COMPU-RATIONAL-COEFFS>\n                </ho:COMPU-SCALE>\n              </ho:COMPU-SCALES>\n            </ho:COMPU-INTERNAL-TO-PHYS>\n          </ho:COMPU-METHOD>\n        </ho:COMPU-METHODS>\n      </fx:CODING>\n      <fx:CODING ID=\"cod9\">\n        <ho:SHORT-NAME>cod9</ho:SHORT-NAME>\n        <ho:CODED-TYPE ho:BASE-DATA-TYPE=\"A_UINT8\" CATEGORY=\"STANDARD-LENGTH-TYPE\" ENCODING=\"UNSIGNED\">\n          <ho:BIT-LENGTH>8</ho:BIT-LENGTH>\n        </ho:CODED-TYPE>\n        <ho:COMPU-METHODS>\n          <ho:COMPU-METHOD>\n            <ho:SHORT-NAME>cpm9</ho:SHORT-NAME>\n            <ho:CATEGORY>LINEAR</ho:CATEGORY>\n            <ho:UNIT-REF ID-REF=\"unit9\"/>\n            <ho:PHYS-CONSTRS>\n              <ho:SCALE-CONSTR>\n                <ho:LOWER-LIMIT INTERVAL-TYPE=\"CLOSED\">0</ho:LOWER-LIMIT>\n                <ho:UPPER-LIMIT INTERVAL-TYPE=\"CLOSED\">255</ho:UPPER-LIMIT>\n              </ho:SCALE-CONSTR>\n            </ho:PHYS-CONSTRS>\n            <ho:COMPU-INTERNAL-TO-PHYS>\n              <ho:COMPU-SCALES>\n                <ho:COMPU-SCALE>\n                  <ho:COMPU-RATIONAL-COEFFS>\n                    <ho:COMPU-NUMERATOR>\n                      <ho:V>0</ho:V>\n                      <ho:V>1</ho:V>\n                    </ho:COMPU-NUMERATOR>\n                    <ho:COMPU-DENOMINATOR>\n                      <ho:V>1</ho:V>\n                    </ho:COMPU-DENOMINATOR>\n                  </ho:COMPU-RATIONAL-COEFFS>\n                </ho:COMPU-SCALE>\n              </ho:COMPU-SCALES>\n            </ho:COMPU-INTERNAL-TO-PHYS>\n          </ho:COMPU-METHOD>\n        </ho:COMPU-METHODS>\n      </fx:CODING>\n      <fx:CODING ID=\"cod10\">\n        <ho:SHORT-NAME>cod10</ho:SHORT-NAME>\n        <ho:CODED-TYPE ho:BASE-DATA-TYPE=\"A_UINT8\" CATEGORY=\"STANDARD-LENGTH-TYPE\" ENCODING=\"UNSIGNED\">\n          <ho:BIT-LENGTH>8</ho:BIT-LENGTH>\n        </ho:CODED-TYPE>\n        <ho:COMPU-METHODS>\n          <ho:COMPU-METHOD>\n            <ho:SHORT-NAME>cpm10</ho:SHORT-NAME>\n            <ho:CATEGORY>LINEAR</ho:CATEGORY>\n            <ho:UNIT-REF ID-REF=\"unit10\"/>\n            <ho:PHYS-CONSTRS>\n              <ho:SCALE-CONSTR>\n                <ho:LOWER-LIMIT INTERVAL-TYPE=\"CLOSED\">0</ho:LOWER-LIMIT>\n                <ho:UPPER-LIMIT INTERVAL-TYPE=\"CLOSED\">255</ho:UPPER-LIMIT>\n              </ho:SCALE-CONSTR>\n            </ho:PHYS-CONSTRS>\n            <ho:COMPU-INTERNAL-TO-PHYS>\n              <ho:COMPU-SCALES>\n                <ho:COMPU-SCALE>\n                  <ho:COMPU-RATIONAL-COEFFS>\n                    <ho:COMPU-NUMERATOR>\n                      <ho:V>0</ho:V>\n                      <ho:V>1</ho:V>\n                    </ho:COMPU-NUMERATOR>\n                    <ho:COMPU-DENOMINATOR>\n                      <ho:V>1</ho:V>\n                    </ho:COMPU-DENOMINATOR>\n                  </ho:COMPU-RATIONAL-COEFFS>\n                </ho:COMPU-SCALE>\n              </ho:COMPU-SCALES>\n            </ho:COMPU-INTERNAL-TO-PHYS>\n          </ho:COMPU-METHOD>\n        </ho:COMPU-METHODS>\n      </fx:CODING>\n      <fx:CODING ID=\"cod11\">\n        <ho:SHORT-NAME>cod11</ho:SHORT-NAME>\n        <ho:CODED-TYPE ho:BASE-DATA-TYPE=\"A_UINT16\" CATEGORY=\"STANDARD-LENGTH-TYPE\" ENCODING=\"UNSIGNED\">\n          <ho:BIT-LENGTH>16</ho:BIT-LENGTH>\n        </ho:CODED-TYPE>\n        <ho:COMPU-METHODS>\n          <ho:COMPU-METHOD>\n            <ho:SHORT-NAME>cpm11</ho:SHORT-NAME>\n            <ho:CATEGORY>LINEAR</ho:CATEGORY>\n            <ho:UNIT-REF ID-REF=\"unit11\"/>\n            <ho:PHYS-CONSTRS>\n              <ho:SCALE-CONSTR>\n                <ho:LOWER-LIMIT INTERVAL-TYPE=\"CLOSED\">0</ho:LOWER-LIMIT>\n                <ho:UPPER-LIMIT INTERVAL-TYPE=\"CLOSED\">5</ho:UPPER-LIMIT>\n              </ho:SCALE-CONSTR>\n            </ho:PHYS-CONSTRS>\n            <ho:COMPU-INTERNAL-TO-PHYS>\n              <ho:COMPU-SCALES>\n                <ho:COMPU-SCALE>\n                  <ho:COMPU-RATIONAL-COEFFS>\n                    <ho:COMPU-NUMERATOR>\n                      <ho:V>0</ho:V>\n                      <ho:V>1</ho:V>\n                    </ho:COMPU-NUMERATOR>\n                    <ho:COMPU-DENOMINATOR>\n                      <ho:V>1</ho:V>\n                    </ho:COMPU-DENOMINATOR>\n                  </ho:COMPU-RATIONAL-COEFFS>\n                </ho:COMPU-SCALE>\n              </ho:COMPU-SCALES>\n            </ho:COMPU-INTERNAL-TO-PHYS>\n          </ho:COMPU-METHOD>\n        </ho:COMPU-METHODS>\n      </fx:CODING>\n      <fx:CODING ID=\"cod12\">\n        <ho:SHORT-NAME>cod12</ho:SHORT-NAME>\n        <ho:CODED-TYPE ho:BASE-DATA-TYPE=\"A_UINT16\" CATEGORY=\"STANDARD-LENGTH-TYPE\" ENCODING=\"UNSIGNED\">\n          <ho:BIT-LENGTH>16</ho:BIT-LENGTH>\n        </ho:CODED-TYPE>\n        <ho:COMPU-METHODS>\n          <ho:COMPU-METHOD>\n            <ho:SHORT-NAME>cpm12</ho:SHORT-NAME>\n            <ho:CATEGORY>LINEAR</ho:CATEGORY>\n            <ho:UNIT-REF ID-REF=\"unit12\"/>\n            <ho:PHYS-CONSTRS>\n              <ho:SCALE-CONSTR>\n                <ho:LOWER-LIMIT INTERVAL-TYPE=\"CLOSED\">0</ho:LOWER-LIMIT>\n                <ho:UPPER-LIMIT INTERVAL-TYPE=\"CLOSED\">5</ho:UPPER-LIMIT>\n              </ho:SCALE-CONSTR>\n            </ho:PHYS-CONSTRS>\n            <ho:COMPU-INTERNAL-TO-PHYS>\n              <ho:COMPU-SCALES>\n                <ho:COMPU-SCALE>\n                  <ho:COMPU-RATIONAL-COEFFS>\n                    <ho:COMPU-NUMERATOR>\n                      <ho:V>0</ho:V>\n                      <ho:V>1</ho:V>\n                    </ho:COMPU-NUMERATOR>\n                    <ho:COMPU-DENOMINATOR>\n                      <ho:V>1</ho:V>\n                    </ho:COMPU-DENOMINATOR>\n                  </ho:COMPU-RATIONAL-COEFFS>\n                </ho:COMPU-SCALE>\n              </ho:COMPU-SCALES>\n            </ho:COMPU-INTERNAL-TO-PHYS>\n          </ho:COMPU-METHOD>\n        </ho:COMPU-METHODS>\n      </fx:CODING>\n      <fx:CODING ID=\"cod13\">\n        <ho:SHORT-NAME>cod13</ho:SHORT-NAME>\n        <ho:CODED-TYPE ho:BASE-DATA-TYPE=\"A_UINT8\" CATEGORY=\"STANDARD-LENGTH-TYPE\" ENCODING=\"UNSIGNED\">\n          <ho:BIT-LENGTH>1</ho:BIT-LENGTH>\n        </ho:CODED-TYPE>\n        <ho:COMPU-METHODS>\n          <ho:COMPU-METHOD>\n            <ho:SHORT-NAME>cpm13</ho:SHORT-NAME>\n            <ho:CATEGORY>LINEAR</ho:CATEGORY>\n            <ho:UNIT-REF ID-REF=\"unit13\"/>\n            <ho:PHYS-CONSTRS>\n              <ho:SCALE-CONSTR>\n                <ho:LOWER-LIMIT INTERVAL-TYPE=\"CLOSED\">0</ho:LOWER-LIMIT>\n                <ho:UPPER-LIMIT INTERVAL-TYPE=\"CLOSED\">1</ho:UPPER-LIMIT>\n              </ho:SCALE-CONSTR>\n            </ho:PHYS-CONSTRS>\n            <ho:COMPU-INTERNAL-TO-PHYS>\n              <ho:COMPU-SCALES>\n                <ho:COMPU-SCALE>\n                  <ho:COMPU-RATIONAL-COEFFS>\n                    <ho:COMPU-NUMERATOR>\n                      <ho:V>0</ho:V>\n                      <ho:V>1</ho:V>\n                    </ho:COMPU-NUMERATOR>\n                    <ho:COMPU-DENOMINATOR>\n                      <ho:V>1</ho:V>\n                    </ho:COMPU-DENOMINATOR>\n                  </ho:COMPU-RATIONAL-COEFFS>\n                </ho:COMPU-SCALE>\n              </ho:COMPU-SCALES>\n            </ho:COMPU-INTERNAL-TO-PHYS>\n          </ho:COMPU-METHOD>\n        </ho:COMPU-METHODS>\n      </fx:CODING>\n      <fx:CODING ID=\"cod14\">\n        <ho:SHORT-NAME>cod14</ho:SHORT-NAME>\n        <ho:CODED-TYPE ho:BASE-DATA-TYPE=\"A_UINT8\" CATEGORY=\"STANDARD-LENGTH-TYPE\" ENCODING=\"UNSIGNED\">\n          <ho:BIT-LENGTH>1</ho:BIT-LENGTH>\n        </ho:CODED-TYPE>\n        <ho:COMPU-METHODS>\n          <ho:COMPU-METHOD>\n            <ho:SHORT-NAME>cpm14</ho:SHORT-NAME>\n            <ho:CATEGORY>LINEAR</ho:CATEGORY>\n            <ho:UNIT-REF ID-REF=\"unit14\"/>\n            <ho:PHYS-CONSTRS>\n              <ho:SCALE-CONSTR>\n                <ho:LOWER-LIMIT INTERVAL-TYPE=\"CLOSED\">0</ho:LOWER-LIMIT>\n                <ho:UPPER-LIMIT INTERVAL-TYPE=\"CLOSED\">1</ho:UPPER-LIMIT>\n              </ho:SCALE-CONSTR>\n            </ho:PHYS-CONSTRS>\n            <ho:COMPU-INTERNAL-TO-PHYS>\n              <ho:COMPU-SCALES>\n                <ho:COMPU-SCALE>\n                  <ho:COMPU-RATIONAL-COEFFS>\n                    <ho:COMPU-NUMERATOR>\n                      <ho:V>0</ho:V>\n                      <ho:V>1</ho:V>\n                    </ho:COMPU-NUMERATOR>\n                    <ho:COMPU-DENOMINATOR>\n                      <ho:V>1</ho:V>\n                    </ho:COMPU-DENOMINATOR>\n                  </ho:COMPU-RATIONAL-COEFFS>\n                </ho:COMPU-SCALE>\n              </ho:COMPU-SCALES>\n            </ho:COMPU-INTERNAL-TO-PHYS>\n          </ho:COMPU-METHOD>\n        </ho:COMPU-METHODS>\n      </fx:CODING>\n      <fx:CODING ID=\"cod15\">\n        <ho:SHORT-NAME>cod15</ho:SHORT-NAME>\n        <ho:CODED-TYPE ho:BASE-DATA-TYPE=\"A_UINT8\" CATEGORY=\"STANDARD-LENGTH-TYPE\" ENCODING=\"UNSIGNED\">\n          <ho:BIT-LENGTH>1</ho:BIT-LENGTH>\n        </ho:CODED-TYPE>\n        <ho:COMPU-METHODS>\n          <ho:COMPU-METHOD>\n            <ho:SHORT-NAME>cpm15</ho:SHORT-NAME>\n            <ho:CATEGORY>LINEAR</ho:CATEGORY>\n            <ho:UNIT-REF ID-REF=\"unit15\"/>\n            <ho:PHYS-CONSTRS>\n              <ho:SCALE-CONSTR>\n                <ho:LOWER-LIMIT INTERVAL-TYPE=\"CLOSED\">0</ho:LOWER-LIMIT>\n                <ho:UPPER-LIMIT INTERVAL-TYPE=\"CLOSED\">1</ho:UPPER-LIMIT>\n              </ho:SCALE-CONSTR>\n            </ho:PHYS-CONSTRS>\n            <ho:COMPU-INTERNAL-TO-PHYS>\n              <ho:COMPU-SCALES>\n                <ho:COMPU-SCALE>\n                  <ho:COMPU-RATIONAL-COEFFS>\n                    <ho:COMPU-NUMERATOR>\n                      <ho:V>0</ho:V>\n                      <ho:V>1</ho:V>\n                    </ho:COMPU-NUMERATOR>\n                    <ho:COMPU-DENOMINATOR>\n                      <ho:V>1</ho:V>\n                    </ho:COMPU-DENOMINATOR>\n                  </ho:COMPU-RATIONAL-COEFFS>\n                </ho:COMPU-SCALE>\n              </ho:COMPU-SCALES>\n            </ho:COMPU-INTERNAL-TO-PHYS>\n          </ho:COMPU-METHOD>\n        </ho:COMPU-METHODS>\n      </fx:CODING>\n      <fx:CODING ID=\"cod16\">\n        <ho:SHORT-NAME>cod16</ho:SHORT-NAME>\n        <ho:CODED-TYPE ho:BASE-DATA-TYPE=\"A_UINT8\" CATEGORY=\"STANDARD-LENGTH-TYPE\" ENCODING=\"UNSIGNED\">\n          <ho:BIT-LENGTH>1</ho:BIT-LENGTH>\n        </ho:CODED-TYPE>\n        <ho:COMPU-METHODS>\n          <ho:COMPU-METHOD>\n            <ho:SHORT-NAME>cpm16</ho:SHORT-NAME>\n            <ho:CATEGORY>LINEAR</ho:CATEGORY>\n            <ho:UNIT-REF ID-REF=\"unit16\"/>\n            <ho:PHYS-CONSTRS>\n              <ho:SCALE-CONSTR>\n                <ho:LOWER-LIMIT INTERVAL-TYPE=\"CLOSED\">0</ho:LOWER-LIMIT>\n                <ho:UPPER-LIMIT INTERVAL-TYPE=\"CLOSED\">1</ho:UPPER-LIMIT>\n              </ho:SCALE-CONSTR>\n            </ho:PHYS-CONSTRS>\n            <ho:COMPU-INTERNAL-TO-PHYS>\n              <ho:COMPU-SCALES>\n                <ho:COMPU-SCALE>\n                  <ho:COMPU-RATIONAL-COEFFS>\n                    <ho:COMPU-NUMERATOR>\n                      <ho:V>0</ho:V>\n                      <ho:V>1</ho:V>\n                    </ho:COMPU-NUMERATOR>\n                    <ho:COMPU-DENOMINATOR>\n                      <ho:V>1</ho:V>\n                    </ho:COMPU-DENOMINATOR>\n                  </ho:COMPU-RATIONAL-COEFFS>\n                </ho:COMPU-SCALE>\n              </ho:COMPU-SCALES>\n            </ho:COMPU-INTERNAL-TO-PHYS>\n          </ho:COMPU-METHOD>\n        </ho:COMPU-METHODS>\n      </fx:CODING>\n      <fx:CODING ID=\"cod17\">\n        <ho:SHORT-NAME>cod17</ho:SHORT-NAME>\n        <ho:CODED-TYPE ho:BASE-DATA-TYPE=\"A_UINT8\" CATEGORY=\"STANDARD-LENGTH-TYPE\" ENCODING=\"UNSIGNED\">\n          <ho:BIT-LENGTH>1</ho:BIT-LENGTH>\n        </ho:CODED-TYPE>\n        <ho:COMPU-METHODS>\n          <ho:COMPU-METHOD>\n            <ho:SHORT-NAME>cpm17</ho:SHORT-NAME>\n            <ho:CATEGORY>LINEAR</ho:CATEGORY>\n            <ho:UNIT-REF ID-REF=\"unit17\"/>\n            <ho:PHYS-CONSTRS>\n              <ho:SCALE-CONSTR>\n                <ho:LOWER-LIMIT INTERVAL-TYPE=\"CLOSED\">0</ho:LOWER-LIMIT>\n                <ho:UPPER-LIMIT INTERVAL-TYPE=\"CLOSED\">1</ho:UPPER-LIMIT>\n              </ho:SCALE-CONSTR>\n            </ho:PHYS-CONSTRS>\n            <ho:COMPU-INTERNAL-TO-PHYS>\n              <ho:COMPU-SCALES>\n                <ho:COMPU-SCALE>\n                  <ho:COMPU-RATIONAL-COEFFS>\n                    <ho:COMPU-NUMERATOR>\n                      <ho:V>0</ho:V>\n                      <ho:V>1</ho:V>\n                    </ho:COMPU-NUMERATOR>\n                    <ho:COMPU-DENOMINATOR>\n                      <ho:V>1</ho:V>\n                    </ho:COMPU-DENOMINATOR>\n                  </ho:COMPU-RATIONAL-COEFFS>\n                </ho:COMPU-SCALE>\n              </ho:COMPU-SCALES>\n            </ho:COMPU-INTERNAL-TO-PHYS>\n          </ho:COMPU-METHOD>\n        </ho:COMPU-METHODS>\n      </fx:CODING>\n      <fx:CODING ID=\"cod18\">\n        <ho:SHORT-NAME>cod18</ho:SHORT-NAME>\n        <ho:CODED-TYPE ho:BASE-DATA-TYPE=\"A_UINT8\" CATEGORY=\"STANDARD-LENGTH-TYPE\" ENCODING=\"UNSIGNED\">\n          <ho:BIT-LENGTH>1</ho:BIT-LENGTH>\n        </ho:CODED-TYPE>\n        <ho:COMPU-METHODS>\n          <ho:COMPU-METHOD>\n            <ho:SHORT-NAME>cpm18</ho:SHORT-NAME>\n            <ho:CATEGORY>LINEAR</ho:CATEGORY>\n            <ho:UNIT-REF ID-REF=\"unit18\"/>\n            <ho:PHYS-CONSTRS>\n              <ho:SCALE-CONSTR>\n                <ho:LOWER-LIMIT INTERVAL-TYPE=\"CLOSED\">0</ho:LOWER-LIMIT>\n                <ho:UPPER-LIMIT INTERVAL-TYPE=\"CLOSED\">1000</ho:UPPER-LIMIT>\n              </ho:SCALE-CONSTR>\n            </ho:PHYS-CONSTRS>\n            <ho:COMPU-INTERNAL-TO-PHYS>\n              <ho:COMPU-SCALES>\n                <ho:COMPU-SCALE>\n                  <ho:COMPU-RATIONAL-COEFFS>\n                    <ho:COMPU-NUMERATOR>\n                      <ho:V>0</ho:V>\n                      <ho:V>1</ho:V>\n                    </ho:COMPU-NUMERATOR>\n                    <ho:COMPU-DENOMINATOR>\n                      <ho:V>1</ho:V>\n                    </ho:COMPU-DENOMINATOR>\n                  </ho:COMPU-RATIONAL-COEFFS>\n                </ho:COMPU-SCALE>\n              </ho:COMPU-SCALES>\n            </ho:COMPU-INTERNAL-TO-PHYS>\n          </ho:COMPU-METHOD>\n        </ho:COMPU-METHODS>\n      </fx:CODING>\n      <fx:CODING ID=\"cod19\">\n        <ho:SHORT-NAME>cod19</ho:SHORT-NAME>\n        <ho:CODED-TYPE ho:BASE-DATA-TYPE=\"A_UINT16\" CATEGORY=\"STANDARD-LENGTH-TYPE\" ENCODING=\"UNSIGNED\">\n          <ho:BIT-LENGTH>16</ho:BIT-LENGTH>\n        </ho:CODED-TYPE>\n        <ho:COMPU-METHODS>\n          <ho:COMPU-METHOD>\n            <ho:SHORT-NAME>cpm19</ho:SHORT-NAME>\n            <ho:CATEGORY>LINEAR</ho:CATEGORY>\n            <ho:UNIT-REF ID-REF=\"unit19\"/>\n            <ho:PHYS-CONSTRS>\n              <ho:SCALE-CONSTR>\n                <ho:LOWER-LIMIT INTERVAL-TYPE=\"CLOSED\">0</ho:LOWER-LIMIT>\n                <ho:UPPER-LIMIT INTERVAL-TYPE=\"CLOSED\">500.0000000000001</ho:UPPER-LIMIT>\n              </ho:SCALE-CONSTR>\n            </ho:PHYS-CONSTRS>\n            <ho:COMPU-INTERNAL-TO-PHYS>\n              <ho:COMPU-SCALES>\n                <ho:COMPU-SCALE>\n                  <ho:COMPU-RATIONAL-COEFFS>\n                    <ho:COMPU-NUMERATOR>\n                      <ho:V>0</ho:V>\n                      <ho:V>1</ho:V>\n                    </ho:COMPU-NUMERATOR>\n                    <ho:COMPU-DENOMINATOR>\n                      <ho:V>1</ho:V>\n                    </ho:COMPU-DENOMINATOR>\n                  </ho:COMPU-RATIONAL-COEFFS>\n                </ho:COMPU-SCALE>\n              </ho:COMPU-SCALES>\n            </ho:COMPU-INTERNAL-TO-PHYS>\n          </ho:COMPU-METHOD>\n        </ho:COMPU-METHODS>\n      </fx:CODING>\n      <fx:CODING ID=\"cod20\">\n        <ho:SHORT-NAME>cod20</ho:SHORT-NAME>\n        <ho:CODED-TYPE ho:BASE-DATA-TYPE=\"A_UINT16\" CATEGORY=\"STANDARD-LENGTH-TYPE\" ENCODING=\"UNSIGNED\">\n          <ho:BIT-LENGTH>16</ho:BIT-LENGTH>\n        </ho:CODED-TYPE>\n        <ho:COMPU-METHODS>\n          <ho:COMPU-METHOD>\n            <ho:SHORT-NAME>cpm20</ho:SHORT-NAME>\n            <ho:CATEGORY>LINEAR</ho:CATEGORY>\n            <ho:UNIT-REF ID-REF=\"unit20\"/>\n            <ho:PHYS-CONSTRS>\n              <ho:SCALE-CONSTR>\n                <ho:LOWER-LIMIT INTERVAL-TYPE=\"CLOSED\">0</ho:LOWER-LIMIT>\n                <ho:UPPER-LIMIT INTERVAL-TYPE=\"CLOSED\">500.0000000000001</ho:UPPER-LIMIT>\n              </ho:SCALE-CONSTR>\n            </ho:PHYS-CONSTRS>\n            <ho:COMPU-INTERNAL-TO-PHYS>\n              <ho:COMPU-SCALES>\n                <ho:COMPU-SCALE>\n                  <ho:COMPU-RATIONAL-COEFFS>\n                    <ho:COMPU-NUMERATOR>\n                      <ho:V>0</ho:V>\n                      <ho:V>1</ho:V>\n                    </ho:COMPU-NUMERATOR>\n                    <ho:COMPU-DENOMINATOR>\n                      <ho:V>1</ho:V>\n                    </ho:COMPU-DENOMINATOR>\n                  </ho:COMPU-RATIONAL-COEFFS>\n                </ho:COMPU-SCALE>\n              </ho:COMPU-SCALES>\n            </ho:COMPU-INTERNAL-TO-PHYS>\n          </ho:COMPU-METHOD>\n        </ho:COMPU-METHODS>\n      </fx:CODING>\n      <fx:CODING ID=\"cod21\">\n        <ho:SHORT-NAME>cod21</ho:SHORT-NAME>\n        <ho:CODED-TYPE ho:BASE-DATA-TYPE=\"A_UINT8\" CATEGORY=\"STANDARD-LENGTH-TYPE\" ENCODING=\"UNSIGNED\">\n          <ho:BIT-LENGTH>8</ho:BIT-LENGTH>\n        </ho:CODED-TYPE>\n        <ho:COMPU-METHODS>\n          <ho:COMPU-METHOD>\n            <ho:SHORT-NAME>cpm21</ho:SHORT-NAME>\n            <ho:CATEGORY>LINEAR</ho:CATEGORY>\n            <ho:UNIT-REF ID-REF=\"unit21\"/>\n            <ho:PHYS-CONSTRS>\n              <ho:SCALE-CONSTR>\n                <ho:LOWER-LIMIT INTERVAL-TYPE=\"CLOSED\">1</ho:LOWER-LIMIT>\n                <ho:UPPER-LIMIT INTERVAL-TYPE=\"CLOSED\">12</ho:UPPER-LIMIT>\n              </ho:SCALE-CONSTR>\n            </ho:PHYS-CONSTRS>\n            <ho:COMPU-INTERNAL-TO-PHYS>\n              <ho:COMPU-SCALES>\n                <ho:COMPU-SCALE>\n                  <ho:COMPU-RATIONAL-COEFFS>\n                    <ho:COMPU-NUMERATOR>\n                      <ho:V>1</ho:V>\n                      <ho:V>1</ho:V>\n                    </ho:COMPU-NUMERATOR>\n                    <ho:COMPU-DENOMINATOR>\n                      <ho:V>1</ho:V>\n                    </ho:COMPU-DENOMINATOR>\n                  </ho:COMPU-RATIONAL-COEFFS>\n                </ho:COMPU-SCALE>\n              </ho:COMPU-SCALES>\n            </ho:COMPU-INTERNAL-TO-PHYS>\n          </ho:COMPU-METHOD>\n        </ho:COMPU-METHODS>\n      </fx:CODING>\n      <fx:CODING ID=\"cod22\">\n        <ho:SHORT-NAME>cod22</ho:SHORT-NAME>\n        <ho:CODED-TYPE ho:BASE-DATA-TYPE=\"A_UINT16\" CATEGORY=\"STANDARD-LENGTH-TYPE\" ENCODING=\"UNSIGNED\">\n          <ho:BIT-LENGTH>16</ho:BIT-LENGTH>\n        </ho:CODED-TYPE>\n        <ho:COMPU-METHODS>\n          <ho:COMPU-METHOD>\n            <ho:SHORT-NAME>cpm22</ho:SHORT-NAME>\n            <ho:CATEGORY>LINEAR</ho:CATEGORY>\n            <ho:UNIT-REF ID-REF=\"unit22\"/>\n            <ho:PHYS-CONSTRS>\n              <ho:SCALE-CONSTR>\n                <ho:LOWER-LIMIT INTERVAL-TYPE=\"CLOSED\">0</ho:LOWER-LIMIT>\n                <ho:UPPER-LIMIT INTERVAL-TYPE=\"CLOSED\">500.0000000000001</ho:UPPER-LIMIT>\n              </ho:SCALE-CONSTR>\n            </ho:PHYS-CONSTRS>\n            <ho:COMPU-INTERNAL-TO-PHYS>\n              <ho:COMPU-SCALES>\n                <ho:COMPU-SCALE>\n                  <ho:COMPU-RATIONAL-COEFFS>\n                    <ho:COMPU-NUMERATOR>\n                      <ho:V>0</ho:V>\n                      <ho:V>1</ho:V>\n                    </ho:COMPU-NUMERATOR>\n                    <ho:COMPU-DENOMINATOR>\n                      <ho:V>1</ho:V>\n                    </ho:COMPU-DENOMINATOR>\n                  </ho:COMPU-RATIONAL-COEFFS>\n                </ho:COMPU-SCALE>\n              </ho:COMPU-SCALES>\n            </ho:COMPU-INTERNAL-TO-PHYS>\n          </ho:COMPU-METHOD>\n        </ho:COMPU-METHODS>\n      </fx:CODING>\n      <fx:CODING ID=\"cod23\">\n        <ho:SHORT-NAME>cod23</ho:SHORT-NAME>\n        <ho:CODED-TYPE ho:BASE-DATA-TYPE=\"A_UINT8\" CATEGORY=\"STANDARD-LENGTH-TYPE\" ENCODING=\"UNSIGNED\">\n          <ho:BIT-LENGTH>8</ho:BIT-LENGTH>\n        </ho:CODED-TYPE>\n        <ho:COMPU-METHODS>\n          <ho:COMPU-METHOD>\n            <ho:SHORT-NAME>cpm23</ho:SHORT-NAME>\n            <ho:CATEGORY>LINEAR</ho:CATEGORY>\n            <ho:UNIT-REF ID-REF=\"unit23\"/>\n            <ho:PHYS-CONSTRS>\n              <ho:SCALE-CONSTR>\n                <ho:LOWER-LIMIT INTERVAL-TYPE=\"CLOSED\">1</ho:LOWER-LIMIT>\n                <ho:UPPER-LIMIT INTERVAL-TYPE=\"CLOSED\">12</ho:UPPER-LIMIT>\n              </ho:SCALE-CONSTR>\n            </ho:PHYS-CONSTRS>\n            <ho:COMPU-INTERNAL-TO-PHYS>\n              <ho:COMPU-SCALES>\n                <ho:COMPU-SCALE>\n                  <ho:COMPU-RATIONAL-COEFFS>\n                    <ho:COMPU-NUMERATOR>\n                      <ho:V>1</ho:V>\n                      <ho:V>1</ho:V>\n                    </ho:COMPU-NUMERATOR>\n                    <ho:COMPU-DENOMINATOR>\n                      <ho:V>1</ho:V>\n                    </ho:COMPU-DENOMINATOR>\n                  </ho:COMPU-RATIONAL-COEFFS>\n                </ho:COMPU-SCALE>\n              </ho:COMPU-SCALES>\n            </ho:COMPU-INTERNAL-TO-PHYS>\n          </ho:COMPU-METHOD>\n        </ho:COMPU-METHODS>\n      </fx:CODING>\n      <fx:CODING ID=\"cod24\">\n        <ho:SHORT-NAME>cod24</ho:SHORT-NAME>\n        <ho:CODED-TYPE ho:BASE-DATA-TYPE=\"A_UINT16\" CATEGORY=\"STANDARD-LENGTH-TYPE\" ENCODING=\"UNSIGNED\">\n          <ho:BIT-LENGTH>16</ho:BIT-LENGTH>\n        </ho:CODED-TYPE>\n        <ho:COMPU-METHODS>\n          <ho:COMPU-METHOD>\n            <ho:SHORT-NAME>cpm24</ho:SHORT-NAME>\n            <ho:CATEGORY>LINEAR</ho:CATEGORY>\n            <ho:UNIT-REF ID-REF=\"unit24\"/>\n            <ho:PHYS-CONSTRS>\n              <ho:SCALE-CONSTR>\n                <ho:LOWER-LIMIT INTERVAL-TYPE=\"CLOSED\">0</ho:LOWER-LIMIT>\n                <ho:UPPER-LIMIT INTERVAL-TYPE=\"CLOSED\">5</ho:UPPER-LIMIT>\n              </ho:SCALE-CONSTR>\n            </ho:PHYS-CONSTRS>\n            <ho:COMPU-INTERNAL-TO-PHYS>\n              <ho:COMPU-SCALES>\n                <ho:COMPU-SCALE>\n                  <ho:COMPU-RATIONAL-COEFFS>\n                    <ho:COMPU-NUMERATOR>\n                      <ho:V>0</ho:V>\n                      <ho:V>1</ho:V>\n                    </ho:COMPU-NUMERATOR>\n                    <ho:COMPU-DENOMINATOR>\n                      <ho:V>1</ho:V>\n                    </ho:COMPU-DENOMINATOR>\n                  </ho:COMPU-RATIONAL-COEFFS>\n                </ho:COMPU-SCALE>\n              </ho:COMPU-SCALES>\n            </ho:COMPU-INTERNAL-TO-PHYS>\n          </ho:COMPU-METHOD>\n        </ho:COMPU-METHODS>\n      </fx:CODING>\n      <fx:CODING ID=\"cod25\">\n        <ho:SHORT-NAME>cod25</ho:SHORT-NAME>\n        <ho:CODED-TYPE ho:BASE-DATA-TYPE=\"A_UINT16\" CATEGORY=\"STANDARD-LENGTH-TYPE\" ENCODING=\"UNSIGNED\">\n          <ho:BIT-LENGTH>16</ho:BIT-LENGTH>\n        </ho:CODED-TYPE>\n        <ho:COMPU-METHODS>\n          <ho:COMPU-METHOD>\n            <ho:SHORT-NAME>cpm25</ho:SHORT-NAME>\n            <ho:CATEGORY>LINEAR</ho:CATEGORY>\n            <ho:UNIT-REF ID-REF=\"unit25\"/>\n            <ho:PHYS-CONSTRS>\n              <ho:SCALE-CONSTR>\n                <ho:LOWER-LIMIT INTERVAL-TYPE=\"CLOSED\">0</ho:LOWER-LIMIT>\n                <ho:UPPER-LIMIT INTERVAL-TYPE=\"CLOSED\">5</ho:UPPER-LIMIT>\n              </ho:SCALE-CONSTR>\n            </ho:PHYS-CONSTRS>\n            <ho:COMPU-INTERNAL-TO-PHYS>\n              <ho:COMPU-SCALES>\n                <ho:COMPU-SCALE>\n                  <ho:COMPU-RATIONAL-COEFFS>\n                    <ho:COMPU-NUMERATOR>\n                      <ho:V>0</ho:V>\n                      <ho:V>1</ho:V>\n                    </ho:COMPU-NUMERATOR>\n                    <ho:COMPU-DENOMINATOR>\n                      <ho:V>1</ho:V>\n                    </ho:COMPU-DENOMINATOR>\n                  </ho:COMPU-RATIONAL-COEFFS>\n                </ho:COMPU-SCALE>\n              </ho:COMPU-SCALES>\n            </ho:COMPU-INTERNAL-TO-PHYS>\n          </ho:COMPU-METHOD>\n        </ho:COMPU-METHODS>\n      </fx:CODING>\n      <fx:CODING ID=\"cod26\">\n        <ho:SHORT-NAME>cod26</ho:SHORT-NAME>\n        <ho:CODED-TYPE ho:BASE-DATA-TYPE=\"A_UINT16\" CATEGORY=\"STANDARD-LENGTH-TYPE\" ENCODING=\"UNSIGNED\">\n          <ho:BIT-LENGTH>16</ho:BIT-LENGTH>\n        </ho:CODED-TYPE>\n        <ho:COMPU-METHODS>\n          <ho:COMPU-METHOD>\n            <ho:SHORT-NAME>cpm26</ho:SHORT-NAME>\n            <ho:CATEGORY>LINEAR</ho:CATEGORY>\n            <ho:UNIT-REF ID-REF=\"unit26\"/>\n            <ho:PHYS-CONSTRS>\n              <ho:SCALE-CONSTR>\n                <ho:LOWER-LIMIT INTERVAL-TYPE=\"CLOSED\">0</ho:LOWER-LIMIT>\n                <ho:UPPER-LIMIT INTERVAL-TYPE=\"CLOSED\">5</ho:UPPER-LIMIT>\n              </ho:SCALE-CONSTR>\n            </ho:PHYS-CONSTRS>\n            <ho:COMPU-INTERNAL-TO-PHYS>\n              <ho:COMPU-SCALES>\n                <ho:COMPU-SCALE>\n                  <ho:COMPU-RATIONAL-COEFFS>\n                    <ho:COMPU-NUMERATOR>\n                      <ho:V>0</ho:V>\n                      <ho:V>1</ho:V>\n                    </ho:COMPU-NUMERATOR>\n                    <ho:COMPU-DENOMINATOR>\n                      <ho:V>1</ho:V>\n                    </ho:COMPU-DENOMINATOR>\n                  </ho:COMPU-RATIONAL-COEFFS>\n                </ho:COMPU-SCALE>\n              </ho:COMPU-SCALES>\n            </ho:COMPU-INTERNAL-TO-PHYS>\n          </ho:COMPU-METHOD>\n        </ho:COMPU-METHODS>\n      </fx:CODING>\n      <fx:CODING ID=\"cod27\">\n        <ho:SHORT-NAME>cod27</ho:SHORT-NAME>\n        <ho:CODED-TYPE ho:BASE-DATA-TYPE=\"A_UINT16\" CATEGORY=\"STANDARD-LENGTH-TYPE\" ENCODING=\"UNSIGNED\">\n          <ho:BIT-LENGTH>16</ho:BIT-LENGTH>\n        </ho:CODED-TYPE>\n        <ho:COMPU-METHODS>\n          <ho:COMPU-METHOD>\n            <ho:SHORT-NAME>cpm27</ho:SHORT-NAME>\n            <ho:CATEGORY>LINEAR</ho:CATEGORY>\n            <ho:UNIT-REF ID-REF=\"unit27\"/>\n            <ho:PHYS-CONSTRS>\n              <ho:SCALE-CONSTR>\n                <ho:LOWER-LIMIT INTERVAL-TYPE=\"CLOSED\">0</ho:LOWER-LIMIT>\n                <ho:UPPER-LIMIT INTERVAL-TYPE=\"CLOSED\">5</ho:UPPER-LIMIT>\n              </ho:SCALE-CONSTR>\n            </ho:PHYS-CONSTRS>\n            <ho:COMPU-INTERNAL-TO-PHYS>\n              <ho:COMPU-SCALES>\n                <ho:COMPU-SCALE>\n                  <ho:COMPU-RATIONAL-COEFFS>\n                    <ho:COMPU-NUMERATOR>\n                      <ho:V>0</ho:V>\n                      <ho:V>1</ho:V>\n                    </ho:COMPU-NUMERATOR>\n                    <ho:COMPU-DENOMINATOR>\n                      <ho:V>1</ho:V>\n                    </ho:COMPU-DENOMINATOR>\n                  </ho:COMPU-RATIONAL-COEFFS>\n                </ho:COMPU-SCALE>\n              </ho:COMPU-SCALES>\n            </ho:COMPU-INTERNAL-TO-PHYS>\n          </ho:COMPU-METHOD>\n        </ho:COMPU-METHODS>\n      </fx:CODING>\n      <fx:CODING ID=\"cod28\">\n        <ho:SHORT-NAME>cod28</ho:SHORT-NAME>\n        <ho:CODED-TYPE ho:BASE-DATA-TYPE=\"A_UINT16\" CATEGORY=\"STANDARD-LENGTH-TYPE\" ENCODING=\"UNSIGNED\">\n          <ho:BIT-LENGTH>16</ho:BIT-LENGTH>\n        </ho:CODED-TYPE>\n        <ho:COMPU-METHODS>\n          <ho:COMPU-METHOD>\n            <ho:SHORT-NAME>cpm28</ho:SHORT-NAME>\n            <ho:CATEGORY>LINEAR</ho:CATEGORY>\n            <ho:UNIT-REF ID-REF=\"unit28\"/>\n            <ho:PHYS-CONSTRS>\n              <ho:SCALE-CONSTR>\n                <ho:LOWER-LIMIT INTERVAL-TYPE=\"CLOSED\">0</ho:LOWER-LIMIT>\n                <ho:UPPER-LIMIT INTERVAL-TYPE=\"CLOSED\">5</ho:UPPER-LIMIT>\n              </ho:SCALE-CONSTR>\n            </ho:PHYS-CONSTRS>\n            <ho:COMPU-INTERNAL-TO-PHYS>\n              <ho:COMPU-SCALES>\n                <ho:COMPU-SCALE>\n                  <ho:COMPU-RATIONAL-COEFFS>\n                    <ho:COMPU-NUMERATOR>\n                      <ho:V>0</ho:V>\n                      <ho:V>1</ho:V>\n                    </ho:COMPU-NUMERATOR>\n                    <ho:COMPU-DENOMINATOR>\n                      <ho:V>1</ho:V>\n                    </ho:COMPU-DENOMINATOR>\n                  </ho:COMPU-RATIONAL-COEFFS>\n                </ho:COMPU-SCALE>\n              </ho:COMPU-SCALES>\n            </ho:COMPU-INTERNAL-TO-PHYS>\n          </ho:COMPU-METHOD>\n        </ho:COMPU-METHODS>\n      </fx:CODING>\n      <fx:CODING ID=\"cod29\">\n        <ho:SHORT-NAME>cod29</ho:SHORT-NAME>\n        <ho:CODED-TYPE ho:BASE-DATA-TYPE=\"A_UINT16\" CATEGORY=\"STANDARD-LENGTH-TYPE\" ENCODING=\"UNSIGNED\">\n          <ho:BIT-LENGTH>16</ho:BIT-LENGTH>\n        </ho:CODED-TYPE>\n        <ho:COMPU-METHODS>\n          <ho:COMPU-METHOD>\n            <ho:SHORT-NAME>cpm29</ho:SHORT-NAME>\n            <ho:CATEGORY>LINEAR</ho:CATEGORY>\n            <ho:UNIT-REF ID-REF=\"unit29\"/>\n            <ho:PHYS-CONSTRS>\n              <ho:SCALE-CONSTR>\n                <ho:LOWER-LIMIT INTERVAL-TYPE=\"CLOSED\">-500.0000000000001</ho:LOWER-LIMIT>\n                <ho:UPPER-LIMIT INTERVAL-TYPE=\"CLOSED\">500.0000000000001</ho:UPPER-LIMIT>\n              </ho:SCALE-CONSTR>\n            </ho:PHYS-CONSTRS>\n            <ho:COMPU-INTERNAL-TO-PHYS>\n              <ho:COMPU-SCALES>\n                <ho:COMPU-SCALE>\n                  <ho:COMPU-RATIONAL-COEFFS>\n                    <ho:COMPU-NUMERATOR>\n                      <ho:V>0</ho:V>\n                      <ho:V>1</ho:V>\n                    </ho:COMPU-NUMERATOR>\n                    <ho:COMPU-DENOMINATOR>\n                      <ho:V>1</ho:V>\n                    </ho:COMPU-DENOMINATOR>\n                  </ho:COMPU-RATIONAL-COEFFS>\n                </ho:COMPU-SCALE>\n              </ho:COMPU-SCALES>\n            </ho:COMPU-INTERNAL-TO-PHYS>\n          </ho:COMPU-METHOD>\n        </ho:COMPU-METHODS>\n      </fx:CODING>\n      <fx:CODING ID=\"cod30\">\n        <ho:SHORT-NAME>cod30</ho:SHORT-NAME>\n        <ho:CODED-TYPE ho:BASE-DATA-TYPE=\"A_UINT16\" CATEGORY=\"STANDARD-LENGTH-TYPE\" ENCODING=\"UNSIGNED\">\n          <ho:BIT-LENGTH>16</ho:BIT-LENGTH>\n        </ho:CODED-TYPE>\n        <ho:COMPU-METHODS>\n          <ho:COMPU-METHOD>\n            <ho:SHORT-NAME>cpm30</ho:SHORT-NAME>\n            <ho:CATEGORY>LINEAR</ho:CATEGORY>\n            <ho:UNIT-REF ID-REF=\"unit30\"/>\n            <ho:PHYS-CONSTRS>\n              <ho:SCALE-CONSTR>\n                <ho:LOWER-LIMIT INTERVAL-TYPE=\"CLOSED\">-500.0000000000001</ho:LOWER-LIMIT>\n                <ho:UPPER-LIMIT INTERVAL-TYPE=\"CLOSED\">500.0000000000001</ho:UPPER-LIMIT>\n              </ho:SCALE-CONSTR>\n            </ho:PHYS-CONSTRS>\n            <ho:COMPU-INTERNAL-TO-PHYS>\n              <ho:COMPU-SCALES>\n                <ho:COMPU-SCALE>\n                  <ho:COMPU-RATIONAL-COEFFS>\n                    <ho:COMPU-NUMERATOR>\n                      <ho:V>0</ho:V>\n                      <ho:V>1</ho:V>\n                    </ho:COMPU-NUMERATOR>\n                    <ho:COMPU-DENOMINATOR>\n                      <ho:V>1</ho:V>\n                    </ho:COMPU-DENOMINATOR>\n                  </ho:COMPU-RATIONAL-COEFFS>\n                </ho:COMPU-SCALE>\n              </ho:COMPU-SCALES>\n            </ho:COMPU-INTERNAL-TO-PHYS>\n          </ho:COMPU-METHOD>\n        </ho:COMPU-METHODS>\n      </fx:CODING>\n      <fx:CODING ID=\"cod31\">\n        <ho:SHORT-NAME>cod31</ho:SHORT-NAME>\n        <ho:CODED-TYPE ho:BASE-DATA-TYPE=\"A_UINT16\" CATEGORY=\"STANDARD-LENGTH-TYPE\" ENCODING=\"UNSIGNED\">\n          <ho:BIT-LENGTH>16</ho:BIT-LENGTH>\n        </ho:CODED-TYPE>\n        <ho:COMPU-METHODS>\n          <ho:COMPU-METHOD>\n            <ho:SHORT-NAME>cpm31</ho:SHORT-NAME>\n            <ho:CATEGORY>LINEAR</ho:CATEGORY>\n            <ho:UNIT-REF ID-REF=\"unit31\"/>\n            <ho:PHYS-CONSTRS>\n              <ho:SCALE-CONSTR>\n                <ho:LOWER-LIMIT INTERVAL-TYPE=\"CLOSED\">-500.0000000000001</ho:LOWER-LIMIT>\n                <ho:UPPER-LIMIT INTERVAL-TYPE=\"CLOSED\">500.0000000000001</ho:UPPER-LIMIT>\n              </ho:SCALE-CONSTR>\n            </ho:PHYS-CONSTRS>\n            <ho:COMPU-INTERNAL-TO-PHYS>\n              <ho:COMPU-SCALES>\n                <ho:COMPU-SCALE>\n                  <ho:COMPU-RATIONAL-COEFFS>\n                    <ho:COMPU-NUMERATOR>\n                      <ho:V>0</ho:V>\n                      <ho:V>1</ho:V>\n                    </ho:COMPU-NUMERATOR>\n                    <ho:COMPU-DENOMINATOR>\n                      <ho:V>1</ho:V>\n                    </ho:COMPU-DENOMINATOR>\n                  </ho:COMPU-RATIONAL-COEFFS>\n                </ho:COMPU-SCALE>\n              </ho:COMPU-SCALES>\n            </ho:COMPU-INTERNAL-TO-PHYS>\n          </ho:COMPU-METHOD>\n        </ho:COMPU-METHODS>\n      </fx:CODING>\n      <fx:CODING ID=\"cod32\">\n        <ho:SHORT-NAME>cod32</ho:SHORT-NAME>\n        <ho:CODED-TYPE ho:BASE-DATA-TYPE=\"A_UINT16\" CATEGORY=\"STANDARD-LENGTH-TYPE\" ENCODING=\"UNSIGNED\">\n          <ho:BIT-LENGTH>16</ho:BIT-LENGTH>\n        </ho:CODED-TYPE>\n        <ho:COMPU-METHODS>\n          <ho:COMPU-METHOD>\n            <ho:SHORT-NAME>cpm32</ho:SHORT-NAME>\n            <ho:CATEGORY>LINEAR</ho:CATEGORY>\n            <ho:UNIT-REF ID-REF=\"unit32\"/>\n            <ho:PHYS-CONSTRS>\n              <ho:SCALE-CONSTR>\n                <ho:LOWER-LIMIT INTERVAL-TYPE=\"CLOSED\">-500.0000000000001</ho:LOWER-LIMIT>\n                <ho:UPPER-LIMIT INTERVAL-TYPE=\"CLOSED\">500.0000000000001</ho:UPPER-LIMIT>\n              </ho:SCALE-CONSTR>\n            </ho:PHYS-CONSTRS>\n            <ho:COMPU-INTERNAL-TO-PHYS>\n              <ho:COMPU-SCALES>\n                <ho:COMPU-SCALE>\n                  <ho:COMPU-RATIONAL-COEFFS>\n                    <ho:COMPU-NUMERATOR>\n                      <ho:V>0</ho:V>\n                      <ho:V>1</ho:V>\n                    </ho:COMPU-NUMERATOR>\n                    <ho:COMPU-DENOMINATOR>\n                      <ho:V>1</ho:V>\n                    </ho:COMPU-DENOMINATOR>\n                  </ho:COMPU-RATIONAL-COEFFS>\n                </ho:COMPU-SCALE>\n              </ho:COMPU-SCALES>\n            </ho:COMPU-INTERNAL-TO-PHYS>\n          </ho:COMPU-METHOD>\n        </ho:COMPU-METHODS>\n      </fx:CODING>\n      <fx:CODING ID=\"cod33\">\n        <ho:SHORT-NAME>cod33</ho:SHORT-NAME>\n        <ho:CODED-TYPE ho:BASE-DATA-TYPE=\"A_UINT8\" CATEGORY=\"STANDARD-LENGTH-TYPE\" ENCODING=\"UNSIGNED\">\n          <ho:BIT-LENGTH>1</ho:BIT-LENGTH>\n        </ho:CODED-TYPE>\n        <ho:COMPU-METHODS>\n          <ho:COMPU-METHOD>\n            <ho:SHORT-NAME>cpm33</ho:SHORT-NAME>\n            <ho:CATEGORY>LINEAR</ho:CATEGORY>\n            <ho:UNIT-REF ID-REF=\"unit33\"/>\n            <ho:PHYS-CONSTRS>\n              <ho:SCALE-CONSTR>\n                <ho:LOWER-LIMIT INTERVAL-TYPE=\"CLOSED\">0</ho:LOWER-LIMIT>\n                <ho:UPPER-LIMIT INTERVAL-TYPE=\"CLOSED\">1</ho:UPPER-LIMIT>\n              </ho:SCALE-CONSTR>\n            </ho:PHYS-CONSTRS>\n            <ho:COMPU-INTERNAL-TO-PHYS>\n              <ho:COMPU-SCALES>\n                <ho:COMPU-SCALE>\n                  <ho:COMPU-RATIONAL-COEFFS>\n                    <ho:COMPU-NUMERATOR>\n                      <ho:V>0</ho:V>\n                      <ho:V>1</ho:V>\n                    </ho:COMPU-NUMERATOR>\n                    <ho:COMPU-DENOMINATOR>\n                      <ho:V>1</ho:V>\n                    </ho:COMPU-DENOMINATOR>\n                  </ho:COMPU-RATIONAL-COEFFS>\n                </ho:COMPU-SCALE>\n              </ho:COMPU-SCALES>\n            </ho:COMPU-INTERNAL-TO-PHYS>\n          </ho:COMPU-METHOD>\n        </ho:COMPU-METHODS>\n      </fx:CODING>\n      <fx:CODING ID=\"cod34\">\n        <ho:SHORT-NAME>cod34</ho:SHORT-NAME>\n        <ho:CODED-TYPE ho:BASE-DATA-TYPE=\"A_UINT8\" CATEGORY=\"STANDARD-LENGTH-TYPE\" ENCODING=\"UNSIGNED\">\n          <ho:BIT-LENGTH>8</ho:BIT-LENGTH>\n        </ho:CODED-TYPE>\n        <ho:COMPU-METHODS>\n          <ho:COMPU-METHOD>\n            <ho:SHORT-NAME>cpm34</ho:SHORT-NAME>\n            <ho:CATEGORY>LINEAR</ho:CATEGORY>\n            <ho:UNIT-REF ID-REF=\"unit34\"/>\n            <ho:PHYS-CONSTRS>\n              <ho:SCALE-CONSTR>\n                <ho:LOWER-LIMIT INTERVAL-TYPE=\"CLOSED\">1</ho:LOWER-LIMIT>\n                <ho:UPPER-LIMIT INTERVAL-TYPE=\"CLOSED\">12</ho:UPPER-LIMIT>\n              </ho:SCALE-CONSTR>\n            </ho:PHYS-CONSTRS>\n            <ho:COMPU-INTERNAL-TO-PHYS>\n              <ho:COMPU-SCALES>\n                <ho:COMPU-SCALE>\n                  <ho:COMPU-RATIONAL-COEFFS>\n                    <ho:COMPU-NUMERATOR>\n                      <ho:V>1</ho:V>\n                      <ho:V>1</ho:V>\n                    </ho:COMPU-NUMERATOR>\n                    <ho:COMPU-DENOMINATOR>\n                      <ho:V>1</ho:V>\n                    </ho:COMPU-DENOMINATOR>\n                  </ho:COMPU-RATIONAL-COEFFS>\n                </ho:COMPU-SCALE>\n              </ho:COMPU-SCALES>\n            </ho:COMPU-INTERNAL-TO-PHYS>\n          </ho:COMPU-METHOD>\n        </ho:COMPU-METHODS>\n      </fx:CODING>\n      <fx:CODING ID=\"cod35\">\n        <ho:SHORT-NAME>cod35</ho:SHORT-NAME>\n        <ho:CODED-TYPE ho:BASE-DATA-TYPE=\"A_UINT8\" CATEGORY=\"STANDARD-LENGTH-TYPE\" ENCODING=\"UNSIGNED\">\n          <ho:BIT-LENGTH>1</ho:BIT-LENGTH>\n        </ho:CODED-TYPE>\n        <ho:COMPU-METHODS>\n          <ho:COMPU-METHOD>\n            <ho:SHORT-NAME>cpm35</ho:SHORT-NAME>\n            <ho:CATEGORY>LINEAR</ho:CATEGORY>\n            <ho:UNIT-REF ID-REF=\"unit35\"/>\n            <ho:PHYS-CONSTRS>\n              <ho:SCALE-CONSTR>\n                <ho:LOWER-LIMIT INTERVAL-TYPE=\"CLOSED\">0</ho:LOWER-LIMIT>\n                <ho:UPPER-LIMIT INTERVAL-TYPE=\"CLOSED\">1</ho:UPPER-LIMIT>\n              </ho:SCALE-CONSTR>\n            </ho:PHYS-CONSTRS>\n            <ho:COMPU-INTERNAL-TO-PHYS>\n              <ho:COMPU-SCALES>\n                <ho:COMPU-SCALE>\n                  <ho:COMPU-RATIONAL-COEFFS>\n                    <ho:COMPU-NUMERATOR>\n                      <ho:V>0</ho:V>\n                      <ho:V>1</ho:V>\n                    </ho:COMPU-NUMERATOR>\n                    <ho:COMPU-DENOMINATOR>\n                      <ho:V>1</ho:V>\n                    </ho:COMPU-DENOMINATOR>\n                  </ho:COMPU-RATIONAL-COEFFS>\n                </ho:COMPU-SCALE>\n              </ho:COMPU-SCALES>\n            </ho:COMPU-INTERNAL-TO-PHYS>\n          </ho:COMPU-METHOD>\n        </ho:COMPU-METHODS>\n      </fx:CODING>\n      <fx:CODING ID=\"cod36\">\n        <ho:SHORT-NAME>cod36</ho:SHORT-NAME>\n        <ho:CODED-TYPE ho:BASE-DATA-TYPE=\"A_UINT8\" CATEGORY=\"STANDARD-LENGTH-TYPE\" ENCODING=\"UNSIGNED\">\n          <ho:BIT-LENGTH>8</ho:BIT-LENGTH>\n        </ho:CODED-TYPE>\n        <ho:COMPU-METHODS>\n          <ho:COMPU-METHOD>\n            <ho:SHORT-NAME>cpm36</ho:SHORT-NAME>\n            <ho:CATEGORY>LINEAR</ho:CATEGORY>\n            <ho:UNIT-REF ID-REF=\"unit36\"/>\n            <ho:PHYS-CONSTRS>\n              <ho:SCALE-CONSTR>\n                <ho:LOWER-LIMIT INTERVAL-TYPE=\"CLOSED\">0</ho:LOWER-LIMIT>\n                <ho:UPPER-LIMIT INTERVAL-TYPE=\"CLOSED\">1000</ho:UPPER-LIMIT>\n              </ho:SCALE-CONSTR>\n            </ho:PHYS-CONSTRS>\n            <ho:COMPU-INTERNAL-TO-PHYS>\n              <ho:COMPU-SCALES>\n                <ho:COMPU-SCALE>\n                  <ho:COMPU-RATIONAL-COEFFS>\n                    <ho:COMPU-NUMERATOR>\n                      <ho:V>0</ho:V>\n                      <ho:V>1</ho:V>\n                    </ho:COMPU-NUMERATOR>\n                    <ho:COMPU-DENOMINATOR>\n                      <ho:V>1</ho:V>\n                    </ho:COMPU-DENOMINATOR>\n                  </ho:COMPU-RATIONAL-COEFFS>\n                </ho:COMPU-SCALE>\n              </ho:COMPU-SCALES>\n            </ho:COMPU-INTERNAL-TO-PHYS>\n          </ho:COMPU-METHOD>\n        </ho:COMPU-METHODS>\n      </fx:CODING>\n      <fx:CODING ID=\"cod37\">\n        <ho:SHORT-NAME>cod37</ho:SHORT-NAME>\n        <ho:CODED-TYPE ho:BASE-DATA-TYPE=\"A_UINT8\" CATEGORY=\"STANDARD-LENGTH-TYPE\" ENCODING=\"UNSIGNED\">\n          <ho:BIT-LENGTH>8</ho:BIT-LENGTH>\n        </ho:CODED-TYPE>\n        <ho:COMPU-METHODS>\n          <ho:COMPU-METHOD>\n            <ho:SHORT-NAME>cpm37</ho:SHORT-NAME>\n            <ho:CATEGORY>LINEAR</ho:CATEGORY>\n            <ho:UNIT-REF ID-REF=\"unit37\"/>\n            <ho:PHYS-CONSTRS>\n              <ho:SCALE-CONSTR>\n                <ho:LOWER-LIMIT INTERVAL-TYPE=\"CLOSED\">0</ho:LOWER-LIMIT>\n                <ho:UPPER-LIMIT INTERVAL-TYPE=\"CLOSED\">1000</ho:UPPER-LIMIT>\n              </ho:SCALE-CONSTR>\n            </ho:PHYS-CONSTRS>\n            <ho:COMPU-INTERNAL-TO-PHYS>\n              <ho:COMPU-SCALES>\n                <ho:COMPU-SCALE>\n                  <ho:COMPU-RATIONAL-COEFFS>\n                    <ho:COMPU-NUMERATOR>\n                      <ho:V>0</ho:V>\n                      <ho:V>1</ho:V>\n                    </ho:COMPU-NUMERATOR>\n                    <ho:COMPU-DENOMINATOR>\n                      <ho:V>1</ho:V>\n                    </ho:COMPU-DENOMINATOR>\n                  </ho:COMPU-RATIONAL-COEFFS>\n                </ho:COMPU-SCALE>\n              </ho:COMPU-SCALES>\n            </ho:COMPU-INTERNAL-TO-PHYS>\n          </ho:COMPU-METHOD>\n        </ho:COMPU-METHODS>\n      </fx:CODING>\n      <fx:CODING ID=\"cod38\">\n        <ho:SHORT-NAME>cod38</ho:SHORT-NAME>\n        <ho:CODED-TYPE ho:BASE-DATA-TYPE=\"A_UINT8\" CATEGORY=\"STANDARD-LENGTH-TYPE\" ENCODING=\"UNSIGNED\">\n          <ho:BIT-LENGTH>8</ho:BIT-LENGTH>\n        </ho:CODED-TYPE>\n        <ho:COMPU-METHODS>\n          <ho:COMPU-METHOD>\n            <ho:SHORT-NAME>cpm38</ho:SHORT-NAME>\n            <ho:CATEGORY>LINEAR</ho:CATEGORY>\n            <ho:UNIT-REF ID-REF=\"unit38\"/>\n            <ho:PHYS-CONSTRS>\n              <ho:SCALE-CONSTR>\n                <ho:LOWER-LIMIT INTERVAL-TYPE=\"CLOSED\">0</ho:LOWER-LIMIT>\n                <ho:UPPER-LIMIT INTERVAL-TYPE=\"CLOSED\">1000</ho:UPPER-LIMIT>\n              </ho:SCALE-CONSTR>\n            </ho:PHYS-CONSTRS>\n            <ho:COMPU-INTERNAL-TO-PHYS>\n              <ho:COMPU-SCALES>\n                <ho:COMPU-SCALE>\n                  <ho:COMPU-RATIONAL-COEFFS>\n                    <ho:COMPU-NUMERATOR>\n                      <ho:V>0</ho:V>\n                      <ho:V>1</ho:V>\n                    </ho:COMPU-NUMERATOR>\n                    <ho:COMPU-DENOMINATOR>\n                      <ho:V>1</ho:V>\n                    </ho:COMPU-DENOMINATOR>\n                  </ho:COMPU-RATIONAL-COEFFS>\n                </ho:COMPU-SCALE>\n              </ho:COMPU-SCALES>\n            </ho:COMPU-INTERNAL-TO-PHYS>\n          </ho:COMPU-METHOD>\n        </ho:COMPU-METHODS>\n      </fx:CODING>\n      <fx:CODING ID=\"cod39\">\n        <ho:SHORT-NAME>cod39</ho:SHORT-NAME>\n        <ho:CODED-TYPE ho:BASE-DATA-TYPE=\"A_UINT8\" CATEGORY=\"STANDARD-LENGTH-TYPE\" ENCODING=\"UNSIGNED\">\n          <ho:BIT-LENGTH>1</ho:BIT-LENGTH>\n        </ho:CODED-TYPE>\n        <ho:COMPU-METHODS>\n          <ho:COMPU-METHOD>\n            <ho:SHORT-NAME>cpm39</ho:SHORT-NAME>\n            <ho:CATEGORY>LINEAR</ho:CATEGORY>\n            <ho:UNIT-REF ID-REF=\"unit39\"/>\n            <ho:PHYS-CONSTRS>\n              <ho:SCALE-CONSTR>\n                <ho:LOWER-LIMIT INTERVAL-TYPE=\"CLOSED\">0</ho:LOWER-LIMIT>\n                <ho:UPPER-LIMIT INTERVAL-TYPE=\"CLOSED\">1</ho:UPPER-LIMIT>\n              </ho:SCALE-CONSTR>\n            </ho:PHYS-CONSTRS>\n            <ho:COMPU-INTERNAL-TO-PHYS>\n              <ho:COMPU-SCALES>\n                <ho:COMPU-SCALE>\n                  <ho:COMPU-RATIONAL-COEFFS>\n                    <ho:COMPU-NUMERATOR>\n                      <ho:V>0</ho:V>\n                      <ho:V>1</ho:V>\n                    </ho:COMPU-NUMERATOR>\n                    <ho:COMPU-DENOMINATOR>\n                      <ho:V>1</ho:V>\n                    </ho:COMPU-DENOMINATOR>\n                  </ho:COMPU-RATIONAL-COEFFS>\n                </ho:COMPU-SCALE>\n              </ho:COMPU-SCALES>\n            </ho:COMPU-INTERNAL-TO-PHYS>\n          </ho:COMPU-METHOD>\n        </ho:COMPU-METHODS>\n      </fx:CODING>\n      <fx:CODING ID=\"cod40\">\n        <ho:SHORT-NAME>cod40</ho:SHORT-NAME>\n        <ho:CODED-TYPE ho:BASE-DATA-TYPE=\"A_UINT8\" CATEGORY=\"STANDARD-LENGTH-TYPE\" ENCODING=\"UNSIGNED\">\n          <ho:BIT-LENGTH>1</ho:BIT-LENGTH>\n        </ho:CODED-TYPE>\n        <ho:COMPU-METHODS>\n          <ho:COMPU-METHOD>\n            <ho:SHORT-NAME>cpm40</ho:SHORT-NAME>\n            <ho:CATEGORY>LINEAR</ho:CATEGORY>\n            <ho:UNIT-REF ID-REF=\"unit40\"/>\n            <ho:PHYS-CONSTRS>\n              <ho:SCALE-CONSTR>\n                <ho:LOWER-LIMIT INTERVAL-TYPE=\"CLOSED\">0</ho:LOWER-LIMIT>\n                <ho:UPPER-LIMIT INTERVAL-TYPE=\"CLOSED\">1</ho:UPPER-LIMIT>\n              </ho:SCALE-CONSTR>\n            </ho:PHYS-CONSTRS>\n            <ho:COMPU-INTERNAL-TO-PHYS>\n              <ho:COMPU-SCALES>\n                <ho:COMPU-SCALE>\n                  <ho:COMPU-RATIONAL-COEFFS>\n                    <ho:COMPU-NUMERATOR>\n                      <ho:V>0</ho:V>\n                      <ho:V>1</ho:V>\n                    </ho:COMPU-NUMERATOR>\n                    <ho:COMPU-DENOMINATOR>\n                      <ho:V>1</ho:V>\n                    </ho:COMPU-DENOMINATOR>\n                  </ho:COMPU-RATIONAL-COEFFS>\n                </ho:COMPU-SCALE>\n              </ho:COMPU-SCALES>\n            </ho:COMPU-INTERNAL-TO-PHYS>\n          </ho:COMPU-METHOD>\n        </ho:COMPU-METHODS>\n      </fx:CODING>\n      <fx:CODING ID=\"cod41\">\n        <ho:SHORT-NAME>cod41</ho:SHORT-NAME>\n        <ho:CODED-TYPE ho:BASE-DATA-TYPE=\"A_UINT8\" CATEGORY=\"STANDARD-LENGTH-TYPE\" ENCODING=\"UNSIGNED\">\n          <ho:BIT-LENGTH>1</ho:BIT-LENGTH>\n        </ho:CODED-TYPE>\n        <ho:COMPU-METHODS>\n          <ho:COMPU-METHOD>\n            <ho:SHORT-NAME>cpm41</ho:SHORT-NAME>\n            <ho:CATEGORY>LINEAR</ho:CATEGORY>\n            <ho:UNIT-REF ID-REF=\"unit41\"/>\n            <ho:PHYS-CONSTRS>\n              <ho:SCALE-CONSTR>\n                <ho:LOWER-LIMIT INTERVAL-TYPE=\"CLOSED\">0</ho:LOWER-LIMIT>\n                <ho:UPPER-LIMIT INTERVAL-TYPE=\"CLOSED\">1</ho:UPPER-LIMIT>\n              </ho:SCALE-CONSTR>\n            </ho:PHYS-CONSTRS>\n            <ho:COMPU-INTERNAL-TO-PHYS>\n              <ho:COMPU-SCALES>\n                <ho:COMPU-SCALE>\n                  <ho:COMPU-RATIONAL-COEFFS>\n                    <ho:COMPU-NUMERATOR>\n                      <ho:V>0</ho:V>\n                      <ho:V>1</ho:V>\n                    </ho:COMPU-NUMERATOR>\n                    <ho:COMPU-DENOMINATOR>\n                      <ho:V>1</ho:V>\n                    </ho:COMPU-DENOMINATOR>\n                  </ho:COMPU-RATIONAL-COEFFS>\n                </ho:COMPU-SCALE>\n              </ho:COMPU-SCALES>\n            </ho:COMPU-INTERNAL-TO-PHYS>\n          </ho:COMPU-METHOD>\n        </ho:COMPU-METHODS>\n      </fx:CODING>\n      <fx:CODING ID=\"cod42\">\n        <ho:SHORT-NAME>cod42</ho:SHORT-NAME>\n        <ho:CODED-TYPE ho:BASE-DATA-TYPE=\"A_UINT8\" CATEGORY=\"STANDARD-LENGTH-TYPE\" ENCODING=\"UNSIGNED\">\n          <ho:BIT-LENGTH>1</ho:BIT-LENGTH>\n        </ho:CODED-TYPE>\n        <ho:COMPU-METHODS>\n          <ho:COMPU-METHOD>\n            <ho:SHORT-NAME>cpm42</ho:SHORT-NAME>\n            <ho:CATEGORY>LINEAR</ho:CATEGORY>\n            <ho:UNIT-REF ID-REF=\"unit42\"/>\n            <ho:PHYS-CONSTRS>\n              <ho:SCALE-CONSTR>\n                <ho:LOWER-LIMIT INTERVAL-TYPE=\"CLOSED\">0</ho:LOWER-LIMIT>\n                <ho:UPPER-LIMIT INTERVAL-TYPE=\"CLOSED\">1</ho:UPPER-LIMIT>\n              </ho:SCALE-CONSTR>\n            </ho:PHYS-CONSTRS>\n            <ho:COMPU-INTERNAL-TO-PHYS>\n              <ho:COMPU-SCALES>\n                <ho:COMPU-SCALE>\n                  <ho:COMPU-RATIONAL-COEFFS>\n                    <ho:COMPU-NUMERATOR>\n                      <ho:V>0</ho:V>\n                      <ho:V>1</ho:V>\n                    </ho:COMPU-NUMERATOR>\n                    <ho:COMPU-DENOMINATOR>\n                      <ho:V>1</ho:V>\n                    </ho:COMPU-DENOMINATOR>\n                  </ho:COMPU-RATIONAL-COEFFS>\n                </ho:COMPU-SCALE>\n              </ho:COMPU-SCALES>\n            </ho:COMPU-INTERNAL-TO-PHYS>\n          </ho:COMPU-METHOD>\n        </ho:COMPU-METHODS>\n      </fx:CODING>\n      <fx:CODING ID=\"cod43\">\n        <ho:SHORT-NAME>cod43</ho:SHORT-NAME>\n        <ho:CODED-TYPE ho:BASE-DATA-TYPE=\"A_UINT16\" CATEGORY=\"STANDARD-LENGTH-TYPE\" ENCODING=\"UNSIGNED\">\n          <ho:BIT-LENGTH>16</ho:BIT-LENGTH>\n        </ho:CODED-TYPE>\n        <ho:COMPU-METHODS>\n          <ho:COMPU-METHOD>\n            <ho:SHORT-NAME>cpm43</ho:SHORT-NAME>\n            <ho:CATEGORY>LINEAR</ho:CATEGORY>\n            <ho:UNIT-REF ID-REF=\"unit43\"/>\n            <ho:PHYS-CONSTRS>\n              <ho:SCALE-CONSTR>\n                <ho:LOWER-LIMIT INTERVAL-TYPE=\"CLOSED\">0</ho:LOWER-LIMIT>\n                <ho:UPPER-LIMIT INTERVAL-TYPE=\"CLOSED\">5</ho:UPPER-LIMIT>\n              </ho:SCALE-CONSTR>\n            </ho:PHYS-CONSTRS>\n            <ho:COMPU-INTERNAL-TO-PHYS>\n              <ho:COMPU-SCALES>\n                <ho:COMPU-SCALE>\n                  <ho:COMPU-RATIONAL-COEFFS>\n                    <ho:COMPU-NUMERATOR>\n                      <ho:V>0</ho:V>\n                      <ho:V>1</ho:V>\n                    </ho:COMPU-NUMERATOR>\n                    <ho:COMPU-DENOMINATOR>\n                      <ho:V>1</ho:V>\n                    </ho:COMPU-DENOMINATOR>\n                  </ho:COMPU-RATIONAL-COEFFS>\n                </ho:COMPU-SCALE>\n              </ho:COMPU-SCALES>\n            </ho:COMPU-INTERNAL-TO-PHYS>\n          </ho:COMPU-METHOD>\n        </ho:COMPU-METHODS>\n      </fx:CODING>\n      <fx:CODING ID=\"cod44\">\n        <ho:SHORT-NAME>cod44</ho:SHORT-NAME>\n        <ho:CODED-TYPE ho:BASE-DATA-TYPE=\"A_UINT16\" CATEGORY=\"STANDARD-LENGTH-TYPE\" ENCODING=\"UNSIGNED\">\n          <ho:BIT-LENGTH>16</ho:BIT-LENGTH>\n        </ho:CODED-TYPE>\n        <ho:COMPU-METHODS>\n          <ho:COMPU-METHOD>\n            <ho:SHORT-NAME>cpm44</ho:SHORT-NAME>\n            <ho:CATEGORY>LINEAR</ho:CATEGORY>\n            <ho:UNIT-REF ID-REF=\"unit44\"/>\n            <ho:PHYS-CONSTRS>\n              <ho:SCALE-CONSTR>\n                <ho:LOWER-LIMIT INTERVAL-TYPE=\"CLOSED\">0</ho:LOWER-LIMIT>\n                <ho:UPPER-LIMIT INTERVAL-TYPE=\"CLOSED\">5</ho:UPPER-LIMIT>\n              </ho:SCALE-CONSTR>\n            </ho:PHYS-CONSTRS>\n            <ho:COMPU-INTERNAL-TO-PHYS>\n              <ho:COMPU-SCALES>\n                <ho:COMPU-SCALE>\n                  <ho:COMPU-RATIONAL-COEFFS>\n                    <ho:COMPU-NUMERATOR>\n                      <ho:V>0</ho:V>\n                      <ho:V>1</ho:V>\n                    </ho:COMPU-NUMERATOR>\n                    <ho:COMPU-DENOMINATOR>\n                      <ho:V>1</ho:V>\n                    </ho:COMPU-DENOMINATOR>\n                  </ho:COMPU-RATIONAL-COEFFS>\n                </ho:COMPU-SCALE>\n              </ho:COMPU-SCALES>\n            </ho:COMPU-INTERNAL-TO-PHYS>\n          </ho:COMPU-METHOD>\n        </ho:COMPU-METHODS>\n      </fx:CODING>\n      <fx:CODING ID=\"cod45\">\n        <ho:SHORT-NAME>cod45</ho:SHORT-NAME>\n        <ho:CODED-TYPE ho:BASE-DATA-TYPE=\"A_UINT16\" CATEGORY=\"STANDARD-LENGTH-TYPE\" ENCODING=\"UNSIGNED\">\n          <ho:BIT-LENGTH>16</ho:BIT-LENGTH>\n        </ho:CODED-TYPE>\n        <ho:COMPU-METHODS>\n          <ho:COMPU-METHOD>\n            <ho:SHORT-NAME>cpm45</ho:SHORT-NAME>\n            <ho:CATEGORY>LINEAR</ho:CATEGORY>\n            <ho:UNIT-REF ID-REF=\"unit45\"/>\n            <ho:PHYS-CONSTRS>\n              <ho:SCALE-CONSTR>\n                <ho:LOWER-LIMIT INTERVAL-TYPE=\"CLOSED\">0</ho:LOWER-LIMIT>\n                <ho:UPPER-LIMIT INTERVAL-TYPE=\"CLOSED\">5</ho:UPPER-LIMIT>\n              </ho:SCALE-CONSTR>\n            </ho:PHYS-CONSTRS>\n            <ho:COMPU-INTERNAL-TO-PHYS>\n              <ho:COMPU-SCALES>\n                <ho:COMPU-SCALE>\n                  <ho:COMPU-RATIONAL-COEFFS>\n                    <ho:COMPU-NUMERATOR>\n                      <ho:V>0</ho:V>\n                      <ho:V>1</ho:V>\n                    </ho:COMPU-NUMERATOR>\n                    <ho:COMPU-DENOMINATOR>\n                      <ho:V>1</ho:V>\n                    </ho:COMPU-DENOMINATOR>\n                  </ho:COMPU-RATIONAL-COEFFS>\n                </ho:COMPU-SCALE>\n              </ho:COMPU-SCALES>\n            </ho:COMPU-INTERNAL-TO-PHYS>\n          </ho:COMPU-METHOD>\n        </ho:COMPU-METHODS>\n      </fx:CODING>\n      <fx:CODING ID=\"cod46\">\n        <ho:SHORT-NAME>cod46</ho:SHORT-NAME>\n        <ho:CODED-TYPE ho:BASE-DATA-TYPE=\"A_UINT16\" CATEGORY=\"STANDARD-LENGTH-TYPE\" ENCODING=\"UNSIGNED\">\n          <ho:BIT-LENGTH>16</ho:BIT-LENGTH>\n        </ho:CODED-TYPE>\n        <ho:COMPU-METHODS>\n          <ho:COMPU-METHOD>\n            <ho:SHORT-NAME>cpm46</ho:SHORT-NAME>\n            <ho:CATEGORY>LINEAR</ho:CATEGORY>\n            <ho:UNIT-REF ID-REF=\"unit46\"/>\n            <ho:PHYS-CONSTRS>\n              <ho:SCALE-CONSTR>\n                <ho:LOWER-LIMIT INTERVAL-TYPE=\"CLOSED\">0</ho:LOWER-LIMIT>\n                <ho:UPPER-LIMIT INTERVAL-TYPE=\"CLOSED\">5</ho:UPPER-LIMIT>\n              </ho:SCALE-CONSTR>\n            </ho:PHYS-CONSTRS>\n            <ho:COMPU-INTERNAL-TO-PHYS>\n              <ho:COMPU-SCALES>\n                <ho:COMPU-SCALE>\n                  <ho:COMPU-RATIONAL-COEFFS>\n                    <ho:COMPU-NUMERATOR>\n                      <ho:V>0</ho:V>\n                      <ho:V>1</ho:V>\n                    </ho:COMPU-NUMERATOR>\n                    <ho:COMPU-DENOMINATOR>\n                      <ho:V>1</ho:V>\n                    </ho:COMPU-DENOMINATOR>\n                  </ho:COMPU-RATIONAL-COEFFS>\n                </ho:COMPU-SCALE>\n              </ho:COMPU-SCALES>\n            </ho:COMPU-INTERNAL-TO-PHYS>\n          </ho:COMPU-METHOD>\n        </ho:COMPU-METHODS>\n      </fx:CODING>\n      <fx:CODING ID=\"cod47\">\n        <ho:SHORT-NAME>cod47</ho:SHORT-NAME>\n        <ho:CODED-TYPE ho:BASE-DATA-TYPE=\"A_UINT16\" CATEGORY=\"STANDARD-LENGTH-TYPE\" ENCODING=\"UNSIGNED\">\n          <ho:BIT-LENGTH>16</ho:BIT-LENGTH>\n        </ho:CODED-TYPE>\n        <ho:COMPU-METHODS>\n          <ho:COMPU-METHOD>\n            <ho:SHORT-NAME>cpm47</ho:SHORT-NAME>\n            <ho:CATEGORY>LINEAR</ho:CATEGORY>\n            <ho:UNIT-REF ID-REF=\"unit47\"/>\n            <ho:PHYS-CONSTRS>\n              <ho:SCALE-CONSTR>\n                <ho:LOWER-LIMIT INTERVAL-TYPE=\"CLOSED\">0</ho:LOWER-LIMIT>\n                <ho:UPPER-LIMIT INTERVAL-TYPE=\"CLOSED\">5</ho:UPPER-LIMIT>\n              </ho:SCALE-CONSTR>\n            </ho:PHYS-CONSTRS>\n            <ho:COMPU-INTERNAL-TO-PHYS>\n              <ho:COMPU-SCALES>\n                <ho:COMPU-SCALE>\n                  <ho:COMPU-RATIONAL-COEFFS>\n                    <ho:COMPU-NUMERATOR>\n                      <ho:V>0</ho:V>\n                      <ho:V>1</ho:V>\n                    </ho:COMPU-NUMERATOR>\n                    <ho:COMPU-DENOMINATOR>\n                      <ho:V>1</ho:V>\n                    </ho:COMPU-DENOMINATOR>\n                  </ho:COMPU-RATIONAL-COEFFS>\n                </ho:COMPU-SCALE>\n              </ho:COMPU-SCALES>\n            </ho:COMPU-INTERNAL-TO-PHYS>\n          </ho:COMPU-METHOD>\n        </ho:COMPU-METHODS>\n      </fx:CODING>\n      <fx:CODING ID=\"cod48\">\n        <ho:SHORT-NAME>cod48</ho:SHORT-NAME>\n        <ho:CODED-TYPE ho:BASE-DATA-TYPE=\"A_UINT16\" CATEGORY=\"STANDARD-LENGTH-TYPE\" ENCODING=\"UNSIGNED\">\n          <ho:BIT-LENGTH>16</ho:BIT-LENGTH>\n        </ho:CODED-TYPE>\n        <ho:COMPU-METHODS>\n          <ho:COMPU-METHOD>\n            <ho:SHORT-NAME>cpm48</ho:SHORT-NAME>\n            <ho:CATEGORY>LINEAR</ho:CATEGORY>\n            <ho:UNIT-REF ID-REF=\"unit48\"/>\n            <ho:PHYS-CONSTRS>\n              <ho:SCALE-CONSTR>\n                <ho:LOWER-LIMIT INTERVAL-TYPE=\"CLOSED\">0</ho:LOWER-LIMIT>\n                <ho:UPPER-LIMIT INTERVAL-TYPE=\"CLOSED\">5</ho:UPPER-LIMIT>\n              </ho:SCALE-CONSTR>\n            </ho:PHYS-CONSTRS>\n            <ho:COMPU-INTERNAL-TO-PHYS>\n              <ho:COMPU-SCALES>\n                <ho:COMPU-SCALE>\n                  <ho:COMPU-RATIONAL-COEFFS>\n                    <ho:COMPU-NUMERATOR>\n                      <ho:V>0</ho:V>\n                      <ho:V>1</ho:V>\n                    </ho:COMPU-NUMERATOR>\n                    <ho:COMPU-DENOMINATOR>\n                      <ho:V>1</ho:V>\n                    </ho:COMPU-DENOMINATOR>\n                  </ho:COMPU-RATIONAL-COEFFS>\n                </ho:COMPU-SCALE>\n              </ho:COMPU-SCALES>\n            </ho:COMPU-INTERNAL-TO-PHYS>\n          </ho:COMPU-METHOD>\n        </ho:COMPU-METHODS>\n      </fx:CODING>\n      <fx:CODING ID=\"cod49\">\n        <ho:SHORT-NAME>cod49</ho:SHORT-NAME>\n        <ho:CODED-TYPE ho:BASE-DATA-TYPE=\"A_UINT16\" CATEGORY=\"STANDARD-LENGTH-TYPE\" ENCODING=\"UNSIGNED\">\n          <ho:BIT-LENGTH>16</ho:BIT-LENGTH>\n        </ho:CODED-TYPE>\n        <ho:COMPU-METHODS>\n          <ho:COMPU-METHOD>\n            <ho:SHORT-NAME>cpm49</ho:SHORT-NAME>\n            <ho:CATEGORY>LINEAR</ho:CATEGORY>\n            <ho:UNIT-REF ID-REF=\"unit49\"/>\n            <ho:PHYS-CONSTRS>\n              <ho:SCALE-CONSTR>\n                <ho:LOWER-LIMIT INTERVAL-TYPE=\"CLOSED\">0</ho:LOWER-LIMIT>\n                <ho:UPPER-LIMIT INTERVAL-TYPE=\"CLOSED\">5</ho:UPPER-LIMIT>\n              </ho:SCALE-CONSTR>\n            </ho:PHYS-CONSTRS>\n            <ho:COMPU-INTERNAL-TO-PHYS>\n              <ho:COMPU-SCALES>\n                <ho:COMPU-SCALE>\n                  <ho:COMPU-RATIONAL-COEFFS>\n                    <ho:COMPU-NUMERATOR>\n                      <ho:V>0</ho:V>\n                      <ho:V>1</ho:V>\n                    </ho:COMPU-NUMERATOR>\n                    <ho:COMPU-DENOMINATOR>\n                      <ho:V>1</ho:V>\n                    </ho:COMPU-DENOMINATOR>\n                  </ho:COMPU-RATIONAL-COEFFS>\n                </ho:COMPU-SCALE>\n              </ho:COMPU-SCALES>\n            </ho:COMPU-INTERNAL-TO-PHYS>\n          </ho:COMPU-METHOD>\n        </ho:COMPU-METHODS>\n      </fx:CODING>\n      <fx:CODING ID=\"cod50\">\n        <ho:SHORT-NAME>cod50</ho:SHORT-NAME>\n        <ho:CODED-TYPE ho:BASE-DATA-TYPE=\"A_UINT16\" CATEGORY=\"STANDARD-LENGTH-TYPE\" ENCODING=\"UNSIGNED\">\n          <ho:BIT-LENGTH>16</ho:BIT-LENGTH>\n        </ho:CODED-TYPE>\n        <ho:COMPU-METHODS>\n          <ho:COMPU-METHOD>\n            <ho:SHORT-NAME>cpm50</ho:SHORT-NAME>\n            <ho:CATEGORY>LINEAR</ho:CATEGORY>\n            <ho:UNIT-REF ID-REF=\"unit50\"/>\n            <ho:PHYS-CONSTRS>\n              <ho:SCALE-CONSTR>\n                <ho:LOWER-LIMIT INTERVAL-TYPE=\"CLOSED\">0</ho:LOWER-LIMIT>\n                <ho:UPPER-LIMIT INTERVAL-TYPE=\"CLOSED\">5</ho:UPPER-LIMIT>\n              </ho:SCALE-CONSTR>\n            </ho:PHYS-CONSTRS>\n            <ho:COMPU-INTERNAL-TO-PHYS>\n              <ho:COMPU-SCALES>\n                <ho:COMPU-SCALE>\n                  <ho:COMPU-RATIONAL-COEFFS>\n                    <ho:COMPU-NUMERATOR>\n                      <ho:V>0</ho:V>\n                      <ho:V>1</ho:V>\n                    </ho:COMPU-NUMERATOR>\n                    <ho:COMPU-DENOMINATOR>\n                      <ho:V>1</ho:V>\n                    </ho:COMPU-DENOMINATOR>\n                  </ho:COMPU-RATIONAL-COEFFS>\n                </ho:COMPU-SCALE>\n              </ho:COMPU-SCALES>\n            </ho:COMPU-INTERNAL-TO-PHYS>\n          </ho:COMPU-METHOD>\n        </ho:COMPU-METHODS>\n      </fx:CODING>\n      <fx:CODING ID=\"cod51\">\n        <ho:SHORT-NAME>cod51</ho:SHORT-NAME>\n        <ho:CODED-TYPE ho:BASE-DATA-TYPE=\"A_UINT16\" CATEGORY=\"STANDARD-LENGTH-TYPE\" ENCODING=\"UNSIGNED\">\n          <ho:BIT-LENGTH>16</ho:BIT-LENGTH>\n        </ho:CODED-TYPE>\n        <ho:COMPU-METHODS>\n          <ho:COMPU-METHOD>\n            <ho:SHORT-NAME>cpm51</ho:SHORT-NAME>\n            <ho:CATEGORY>LINEAR</ho:CATEGORY>\n            <ho:UNIT-REF ID-REF=\"unit51\"/>\n            <ho:PHYS-CONSTRS>\n              <ho:SCALE-CONSTR>\n                <ho:LOWER-LIMIT INTERVAL-TYPE=\"CLOSED\">0</ho:LOWER-LIMIT>\n                <ho:UPPER-LIMIT INTERVAL-TYPE=\"CLOSED\">5</ho:UPPER-LIMIT>\n              </ho:SCALE-CONSTR>\n            </ho:PHYS-CONSTRS>\n            <ho:COMPU-INTERNAL-TO-PHYS>\n              <ho:COMPU-SCALES>\n                <ho:COMPU-SCALE>\n                  <ho:COMPU-RATIONAL-COEFFS>\n                    <ho:COMPU-NUMERATOR>\n                      <ho:V>0</ho:V>\n                      <ho:V>1</ho:V>\n                    </ho:COMPU-NUMERATOR>\n                    <ho:COMPU-DENOMINATOR>\n                      <ho:V>1</ho:V>\n                    </ho:COMPU-DENOMINATOR>\n                  </ho:COMPU-RATIONAL-COEFFS>\n                </ho:COMPU-SCALE>\n              </ho:COMPU-SCALES>\n            </ho:COMPU-INTERNAL-TO-PHYS>\n          </ho:COMPU-METHOD>\n        </ho:COMPU-METHODS>\n      </fx:CODING>\n      <fx:CODING ID=\"cod52\">\n        <ho:SHORT-NAME>cod52</ho:SHORT-NAME>\n        <ho:CODED-TYPE ho:BASE-DATA-TYPE=\"A_UINT16\" CATEGORY=\"STANDARD-LENGTH-TYPE\" ENCODING=\"UNSIGNED\">\n          <ho:BIT-LENGTH>16</ho:BIT-LENGTH>\n        </ho:CODED-TYPE>\n        <ho:COMPU-METHODS>\n          <ho:COMPU-METHOD>\n            <ho:SHORT-NAME>cpm52</ho:SHORT-NAME>\n            <ho:CATEGORY>LINEAR</ho:CATEGORY>\n            <ho:UNIT-REF ID-REF=\"unit52\"/>\n            <ho:PHYS-CONSTRS>\n              <ho:SCALE-CONSTR>\n                <ho:LOWER-LIMIT INTERVAL-TYPE=\"CLOSED\">0</ho:LOWER-LIMIT>\n                <ho:UPPER-LIMIT INTERVAL-TYPE=\"CLOSED\">5</ho:UPPER-LIMIT>\n              </ho:SCALE-CONSTR>\n            </ho:PHYS-CONSTRS>\n            <ho:COMPU-INTERNAL-TO-PHYS>\n              <ho:COMPU-SCALES>\n                <ho:COMPU-SCALE>\n                  <ho:COMPU-RATIONAL-COEFFS>\n                    <ho:COMPU-NUMERATOR>\n                      <ho:V>0</ho:V>\n                      <ho:V>1</ho:V>\n                    </ho:COMPU-NUMERATOR>\n                    <ho:COMPU-DENOMINATOR>\n                      <ho:V>1</ho:V>\n                    </ho:COMPU-DENOMINATOR>\n                  </ho:COMPU-RATIONAL-COEFFS>\n                </ho:COMPU-SCALE>\n              </ho:COMPU-SCALES>\n            </ho:COMPU-INTERNAL-TO-PHYS>\n          </ho:COMPU-METHOD>\n        </ho:COMPU-METHODS>\n      </fx:CODING>\n      <fx:CODING ID=\"cod53\">\n        <ho:SHORT-NAME>cod53</ho:SHORT-NAME>\n        <ho:CODED-TYPE ho:BASE-DATA-TYPE=\"A_UINT16\" CATEGORY=\"STANDARD-LENGTH-TYPE\" ENCODING=\"UNSIGNED\">\n          <ho:BIT-LENGTH>16</ho:BIT-LENGTH>\n        </ho:CODED-TYPE>\n        <ho:COMPU-METHODS>\n          <ho:COMPU-METHOD>\n            <ho:SHORT-NAME>cpm53</ho:SHORT-NAME>\n            <ho:CATEGORY>LINEAR</ho:CATEGORY>\n            <ho:UNIT-REF ID-REF=\"unit53\"/>\n            <ho:PHYS-CONSTRS>\n              <ho:SCALE-CONSTR>\n                <ho:LOWER-LIMIT INTERVAL-TYPE=\"CLOSED\">0</ho:LOWER-LIMIT>\n                <ho:UPPER-LIMIT INTERVAL-TYPE=\"CLOSED\">5</ho:UPPER-LIMIT>\n              </ho:SCALE-CONSTR>\n            </ho:PHYS-CONSTRS>\n            <ho:COMPU-INTERNAL-TO-PHYS>\n              <ho:COMPU-SCALES>\n                <ho:COMPU-SCALE>\n                  <ho:COMPU-RATIONAL-COEFFS>\n                    <ho:COMPU-NUMERATOR>\n                      <ho:V>0</ho:V>\n                      <ho:V>1</ho:V>\n                    </ho:COMPU-NUMERATOR>\n                    <ho:COMPU-DENOMINATOR>\n                      <ho:V>1</ho:V>\n                    </ho:COMPU-DENOMINATOR>\n                  </ho:COMPU-RATIONAL-COEFFS>\n                </ho:COMPU-SCALE>\n              </ho:COMPU-SCALES>\n            </ho:COMPU-INTERNAL-TO-PHYS>\n          </ho:COMPU-METHOD>\n        </ho:COMPU-METHODS>\n      </fx:CODING>\n      <fx:CODING ID=\"cod54\">\n        <ho:SHORT-NAME>cod54</ho:SHORT-NAME>\n        <ho:CODED-TYPE ho:BASE-DATA-TYPE=\"A_UINT16\" CATEGORY=\"STANDARD-LENGTH-TYPE\" ENCODING=\"UNSIGNED\">\n          <ho:BIT-LENGTH>16</ho:BIT-LENGTH>\n        </ho:CODED-TYPE>\n        <ho:COMPU-METHODS>\n          <ho:COMPU-METHOD>\n            <ho:SHORT-NAME>cpm54</ho:SHORT-NAME>\n            <ho:CATEGORY>LINEAR</ho:CATEGORY>\n            <ho:UNIT-REF ID-REF=\"unit54\"/>\n            <ho:PHYS-CONSTRS>\n              <ho:SCALE-CONSTR>\n                <ho:LOWER-LIMIT INTERVAL-TYPE=\"CLOSED\">0</ho:LOWER-LIMIT>\n                <ho:UPPER-LIMIT INTERVAL-TYPE=\"CLOSED\">5</ho:UPPER-LIMIT>\n              </ho:SCALE-CONSTR>\n            </ho:PHYS-CONSTRS>\n            <ho:COMPU-INTERNAL-TO-PHYS>\n              <ho:COMPU-SCALES>\n                <ho:COMPU-SCALE>\n                  <ho:COMPU-RATIONAL-COEFFS>\n                    <ho:COMPU-NUMERATOR>\n                      <ho:V>0</ho:V>\n                      <ho:V>1</ho:V>\n                    </ho:COMPU-NUMERATOR>\n                    <ho:COMPU-DENOMINATOR>\n                      <ho:V>1</ho:V>\n                    </ho:COMPU-DENOMINATOR>\n                  </ho:COMPU-RATIONAL-COEFFS>\n                </ho:COMPU-SCALE>\n              </ho:COMPU-SCALES>\n            </ho:COMPU-INTERNAL-TO-PHYS>\n          </ho:COMPU-METHOD>\n        </ho:COMPU-METHODS>\n      </fx:CODING>\n      <fx:CODING ID=\"cod55\">\n        <ho:SHORT-NAME>cod55</ho:SHORT-NAME>\n        <ho:CODED-TYPE ho:BASE-DATA-TYPE=\"A_UINT16\" CATEGORY=\"STANDARD-LENGTH-TYPE\" ENCODING=\"UNSIGNED\">\n          <ho:BIT-LENGTH>16</ho:BIT-LENGTH>\n        </ho:CODED-TYPE>\n        <ho:COMPU-METHODS>\n          <ho:COMPU-METHOD>\n            <ho:SHORT-NAME>cpm55</ho:SHORT-NAME>\n            <ho:CATEGORY>LINEAR</ho:CATEGORY>\n            <ho:UNIT-REF ID-REF=\"unit55\"/>\n            <ho:PHYS-CONSTRS>\n              <ho:SCALE-CONSTR>\n                <ho:LOWER-LIMIT INTERVAL-TYPE=\"CLOSED\">0</ho:LOWER-LIMIT>\n                <ho:UPPER-LIMIT INTERVAL-TYPE=\"CLOSED\">5</ho:UPPER-LIMIT>\n              </ho:SCALE-CONSTR>\n            </ho:PHYS-CONSTRS>\n            <ho:COMPU-INTERNAL-TO-PHYS>\n              <ho:COMPU-SCALES>\n                <ho:COMPU-SCALE>\n                  <ho:COMPU-RATIONAL-COEFFS>\n                    <ho:COMPU-NUMERATOR>\n                      <ho:V>0</ho:V>\n                      <ho:V>1</ho:V>\n                    </ho:COMPU-NUMERATOR>\n                    <ho:COMPU-DENOMINATOR>\n                      <ho:V>1</ho:V>\n                    </ho:COMPU-DENOMINATOR>\n                  </ho:COMPU-RATIONAL-COEFFS>\n                </ho:COMPU-SCALE>\n              </ho:COMPU-SCALES>\n            </ho:COMPU-INTERNAL-TO-PHYS>\n          </ho:COMPU-METHOD>\n        </ho:COMPU-METHODS>\n      </fx:CODING>\n      <fx:CODING ID=\"cod56\">\n        <ho:SHORT-NAME>cod56</ho:SHORT-NAME>\n        <ho:CODED-TYPE ho:BASE-DATA-TYPE=\"A_UINT16\" CATEGORY=\"STANDARD-LENGTH-TYPE\" ENCODING=\"UNSIGNED\">\n          <ho:BIT-LENGTH>16</ho:BIT-LENGTH>\n        </ho:CODED-TYPE>\n        <ho:COMPU-METHODS>\n          <ho:COMPU-METHOD>\n            <ho:SHORT-NAME>cpm56</ho:SHORT-NAME>\n            <ho:CATEGORY>LINEAR</ho:CATEGORY>\n            <ho:UNIT-REF ID-REF=\"unit56\"/>\n            <ho:PHYS-CONSTRS>\n              <ho:SCALE-CONSTR>\n                <ho:LOWER-LIMIT INTERVAL-TYPE=\"CLOSED\">0</ho:LOWER-LIMIT>\n                <ho:UPPER-LIMIT INTERVAL-TYPE=\"CLOSED\">5</ho:UPPER-LIMIT>\n              </ho:SCALE-CONSTR>\n            </ho:PHYS-CONSTRS>\n            <ho:COMPU-INTERNAL-TO-PHYS>\n              <ho:COMPU-SCALES>\n                <ho:COMPU-SCALE>\n                  <ho:COMPU-RATIONAL-COEFFS>\n                    <ho:COMPU-NUMERATOR>\n                      <ho:V>0</ho:V>\n                      <ho:V>1</ho:V>\n                    </ho:COMPU-NUMERATOR>\n                    <ho:COMPU-DENOMINATOR>\n                      <ho:V>1</ho:V>\n                    </ho:COMPU-DENOMINATOR>\n                  </ho:COMPU-RATIONAL-COEFFS>\n                </ho:COMPU-SCALE>\n              </ho:COMPU-SCALES>\n            </ho:COMPU-INTERNAL-TO-PHYS>\n          </ho:COMPU-METHOD>\n        </ho:COMPU-METHODS>\n      </fx:CODING>\n      <fx:CODING ID=\"cod57\">\n        <ho:SHORT-NAME>cod57</ho:SHORT-NAME>\n        <ho:CODED-TYPE ho:BASE-DATA-TYPE=\"A_UINT16\" CATEGORY=\"STANDARD-LENGTH-TYPE\" ENCODING=\"UNSIGNED\">\n          <ho:BIT-LENGTH>16</ho:BIT-LENGTH>\n        </ho:CODED-TYPE>\n        <ho:COMPU-METHODS>\n          <ho:COMPU-METHOD>\n            <ho:SHORT-NAME>cpm57</ho:SHORT-NAME>\n            <ho:CATEGORY>LINEAR</ho:CATEGORY>\n            <ho:UNIT-REF ID-REF=\"unit57\"/>\n            <ho:PHYS-CONSTRS>\n              <ho:SCALE-CONSTR>\n                <ho:LOWER-LIMIT INTERVAL-TYPE=\"CLOSED\">0</ho:LOWER-LIMIT>\n                <ho:UPPER-LIMIT INTERVAL-TYPE=\"CLOSED\">5</ho:UPPER-LIMIT>\n              </ho:SCALE-CONSTR>\n            </ho:PHYS-CONSTRS>\n            <ho:COMPU-INTERNAL-TO-PHYS>\n              <ho:COMPU-SCALES>\n                <ho:COMPU-SCALE>\n                  <ho:COMPU-RATIONAL-COEFFS>\n                    <ho:COMPU-NUMERATOR>\n                      <ho:V>0</ho:V>\n                      <ho:V>1</ho:V>\n                    </ho:COMPU-NUMERATOR>\n                    <ho:COMPU-DENOMINATOR>\n                      <ho:V>1</ho:V>\n                    </ho:COMPU-DENOMINATOR>\n                  </ho:COMPU-RATIONAL-COEFFS>\n                </ho:COMPU-SCALE>\n              </ho:COMPU-SCALES>\n            </ho:COMPU-INTERNAL-TO-PHYS>\n          </ho:COMPU-METHOD>\n        </ho:COMPU-METHODS>\n      </fx:CODING>\n      <fx:CODING ID=\"cod58\">\n        <ho:SHORT-NAME>cod58</ho:SHORT-NAME>\n        <ho:CODED-TYPE ho:BASE-DATA-TYPE=\"A_UINT16\" CATEGORY=\"STANDARD-LENGTH-TYPE\" ENCODING=\"UNSIGNED\">\n          <ho:BIT-LENGTH>16</ho:BIT-LENGTH>\n        </ho:CODED-TYPE>\n        <ho:COMPU-METHODS>\n          <ho:COMPU-METHOD>\n            <ho:SHORT-NAME>cpm58</ho:SHORT-NAME>\n            <ho:CATEGORY>LINEAR</ho:CATEGORY>\n            <ho:UNIT-REF ID-REF=\"unit58\"/>\n            <ho:PHYS-CONSTRS>\n              <ho:SCALE-CONSTR>\n                <ho:LOWER-LIMIT INTERVAL-TYPE=\"CLOSED\">0</ho:LOWER-LIMIT>\n                <ho:UPPER-LIMIT INTERVAL-TYPE=\"CLOSED\">5</ho:UPPER-LIMIT>\n              </ho:SCALE-CONSTR>\n            </ho:PHYS-CONSTRS>\n            <ho:COMPU-INTERNAL-TO-PHYS>\n              <ho:COMPU-SCALES>\n                <ho:COMPU-SCALE>\n                  <ho:COMPU-RATIONAL-COEFFS>\n                    <ho:COMPU-NUMERATOR>\n                      <ho:V>0</ho:V>\n                      <ho:V>1</ho:V>\n                    </ho:COMPU-NUMERATOR>\n                    <ho:COMPU-DENOMINATOR>\n                      <ho:V>1</ho:V>\n                    </ho:COMPU-DENOMINATOR>\n                  </ho:COMPU-RATIONAL-COEFFS>\n                </ho:COMPU-SCALE>\n              </ho:COMPU-SCALES>\n            </ho:COMPU-INTERNAL-TO-PHYS>\n          </ho:COMPU-METHOD>\n        </ho:COMPU-METHODS>\n      </fx:CODING>\n      <fx:CODING ID=\"cod59\">\n        <ho:SHORT-NAME>cod59</ho:SHORT-NAME>\n        <ho:CODED-TYPE ho:BASE-DATA-TYPE=\"A_UINT16\" CATEGORY=\"STANDARD-LENGTH-TYPE\" ENCODING=\"UNSIGNED\">\n          <ho:BIT-LENGTH>16</ho:BIT-LENGTH>\n        </ho:CODED-TYPE>\n        <ho:COMPU-METHODS>\n          <ho:COMPU-METHOD>\n            <ho:SHORT-NAME>cpm59</ho:SHORT-NAME>\n            <ho:CATEGORY>LINEAR</ho:CATEGORY>\n            <ho:UNIT-REF ID-REF=\"unit59\"/>\n            <ho:PHYS-CONSTRS>\n              <ho:SCALE-CONSTR>\n                <ho:LOWER-LIMIT INTERVAL-TYPE=\"CLOSED\">-500.0000000000001</ho:LOWER-LIMIT>\n                <ho:UPPER-LIMIT INTERVAL-TYPE=\"CLOSED\">500.0000000000001</ho:UPPER-LIMIT>\n              </ho:SCALE-CONSTR>\n            </ho:PHYS-CONSTRS>\n            <ho:COMPU-INTERNAL-TO-PHYS>\n              <ho:COMPU-SCALES>\n                <ho:COMPU-SCALE>\n                  <ho:COMPU-RATIONAL-COEFFS>\n                    <ho:COMPU-NUMERATOR>\n                      <ho:V>0</ho:V>\n                      <ho:V>1</ho:V>\n                    </ho:COMPU-NUMERATOR>\n                    <ho:COMPU-DENOMINATOR>\n                      <ho:V>1</ho:V>\n                    </ho:COMPU-DENOMINATOR>\n                  </ho:COMPU-RATIONAL-COEFFS>\n                </ho:COMPU-SCALE>\n              </ho:COMPU-SCALES>\n            </ho:COMPU-INTERNAL-TO-PHYS>\n          </ho:COMPU-METHOD>\n        </ho:COMPU-METHODS>\n      </fx:CODING>\n      <fx:CODING ID=\"cod60\">\n        <ho:SHORT-NAME>cod60</ho:SHORT-NAME>\n        <ho:CODED-TYPE ho:BASE-DATA-TYPE=\"A_UINT16\" CATEGORY=\"STANDARD-LENGTH-TYPE\" ENCODING=\"UNSIGNED\">\n          <ho:BIT-LENGTH>16</ho:BIT-LENGTH>\n        </ho:CODED-TYPE>\n        <ho:COMPU-METHODS>\n          <ho:COMPU-METHOD>\n            <ho:SHORT-NAME>cpm60</ho:SHORT-NAME>\n            <ho:CATEGORY>LINEAR</ho:CATEGORY>\n            <ho:UNIT-REF ID-REF=\"unit60\"/>\n            <ho:PHYS-CONSTRS>\n              <ho:SCALE-CONSTR>\n                <ho:LOWER-LIMIT INTERVAL-TYPE=\"CLOSED\">-500.0000000000001</ho:LOWER-LIMIT>\n                <ho:UPPER-LIMIT INTERVAL-TYPE=\"CLOSED\">500.0000000000001</ho:UPPER-LIMIT>\n              </ho:SCALE-CONSTR>\n            </ho:PHYS-CONSTRS>\n            <ho:COMPU-INTERNAL-TO-PHYS>\n              <ho:COMPU-SCALES>\n                <ho:COMPU-SCALE>\n                  <ho:COMPU-RATIONAL-COEFFS>\n                    <ho:COMPU-NUMERATOR>\n                      <ho:V>0</ho:V>\n                      <ho:V>1</ho:V>\n                    </ho:COMPU-NUMERATOR>\n                    <ho:COMPU-DENOMINATOR>\n                      <ho:V>1</ho:V>\n                    </ho:COMPU-DENOMINATOR>\n                  </ho:COMPU-RATIONAL-COEFFS>\n                </ho:COMPU-SCALE>\n              </ho:COMPU-SCALES>\n            </ho:COMPU-INTERNAL-TO-PHYS>\n          </ho:COMPU-METHOD>\n        </ho:COMPU-METHODS>\n      </fx:CODING>\n      <fx:CODING ID=\"cod61\">\n        <ho:SHORT-NAME>cod61</ho:SHORT-NAME>\n        <ho:CODED-TYPE ho:BASE-DATA-TYPE=\"A_UINT16\" CATEGORY=\"STANDARD-LENGTH-TYPE\" ENCODING=\"UNSIGNED\">\n          <ho:BIT-LENGTH>16</ho:BIT-LENGTH>\n        </ho:CODED-TYPE>\n        <ho:COMPU-METHODS>\n          <ho:COMPU-METHOD>\n            <ho:SHORT-NAME>cpm61</ho:SHORT-NAME>\n            <ho:CATEGORY>LINEAR</ho:CATEGORY>\n            <ho:UNIT-REF ID-REF=\"unit61\"/>\n            <ho:PHYS-CONSTRS>\n              <ho:SCALE-CONSTR>\n                <ho:LOWER-LIMIT INTERVAL-TYPE=\"CLOSED\">-500.0000000000001</ho:LOWER-LIMIT>\n                <ho:UPPER-LIMIT INTERVAL-TYPE=\"CLOSED\">500.0000000000001</ho:UPPER-LIMIT>\n              </ho:SCALE-CONSTR>\n            </ho:PHYS-CONSTRS>\n            <ho:COMPU-INTERNAL-TO-PHYS>\n              <ho:COMPU-SCALES>\n                <ho:COMPU-SCALE>\n                  <ho:COMPU-RATIONAL-COEFFS>\n                    <ho:COMPU-NUMERATOR>\n                      <ho:V>0</ho:V>\n                      <ho:V>1</ho:V>\n                    </ho:COMPU-NUMERATOR>\n                    <ho:COMPU-DENOMINATOR>\n                      <ho:V>1</ho:V>\n                    </ho:COMPU-DENOMINATOR>\n                  </ho:COMPU-RATIONAL-COEFFS>\n                </ho:COMPU-SCALE>\n              </ho:COMPU-SCALES>\n            </ho:COMPU-INTERNAL-TO-PHYS>\n          </ho:COMPU-METHOD>\n        </ho:COMPU-METHODS>\n      </fx:CODING>\n      <fx:CODING ID=\"cod62\">\n        <ho:SHORT-NAME>cod62</ho:SHORT-NAME>\n        <ho:CODED-TYPE ho:BASE-DATA-TYPE=\"A_UINT16\" CATEGORY=\"STANDARD-LENGTH-TYPE\" ENCODING=\"UNSIGNED\">\n          <ho:BIT-LENGTH>16</ho:BIT-LENGTH>\n        </ho:CODED-TYPE>\n        <ho:COMPU-METHODS>\n          <ho:COMPU-METHOD>\n            <ho:SHORT-NAME>cpm62</ho:SHORT-NAME>\n            <ho:CATEGORY>LINEAR</ho:CATEGORY>\n            <ho:UNIT-REF ID-REF=\"unit62\"/>\n            <ho:PHYS-CONSTRS>\n              <ho:SCALE-CONSTR>\n                <ho:LOWER-LIMIT INTERVAL-TYPE=\"CLOSED\">-500.0000000000001</ho:LOWER-LIMIT>\n                <ho:UPPER-LIMIT INTERVAL-TYPE=\"CLOSED\">500.0000000000001</ho:UPPER-LIMIT>\n              </ho:SCALE-CONSTR>\n            </ho:PHYS-CONSTRS>\n            <ho:COMPU-INTERNAL-TO-PHYS>\n              <ho:COMPU-SCALES>\n                <ho:COMPU-SCALE>\n                  <ho:COMPU-RATIONAL-COEFFS>\n                    <ho:COMPU-NUMERATOR>\n                      <ho:V>0</ho:V>\n                      <ho:V>1</ho:V>\n                    </ho:COMPU-NUMERATOR>\n                    <ho:COMPU-DENOMINATOR>\n                      <ho:V>1</ho:V>\n                    </ho:COMPU-DENOMINATOR>\n                  </ho:COMPU-RATIONAL-COEFFS>\n                </ho:COMPU-SCALE>\n              </ho:COMPU-SCALES>\n            </ho:COMPU-INTERNAL-TO-PHYS>\n          </ho:COMPU-METHOD>\n        </ho:COMPU-METHODS>\n      </fx:CODING>\n      <fx:CODING ID=\"cod63\">\n        <ho:SHORT-NAME>cod63</ho:SHORT-NAME>\n        <ho:CODED-TYPE ho:BASE-DATA-TYPE=\"A_UINT16\" CATEGORY=\"STANDARD-LENGTH-TYPE\" ENCODING=\"UNSIGNED\">\n          <ho:BIT-LENGTH>16</ho:BIT-LENGTH>\n        </ho:CODED-TYPE>\n        <ho:COMPU-METHODS>\n          <ho:COMPU-METHOD>\n            <ho:SHORT-NAME>cpm63</ho:SHORT-NAME>\n            <ho:CATEGORY>LINEAR</ho:CATEGORY>\n            <ho:UNIT-REF ID-REF=\"unit63\"/>\n            <ho:PHYS-CONSTRS>\n              <ho:SCALE-CONSTR>\n                <ho:LOWER-LIMIT INTERVAL-TYPE=\"CLOSED\">-500.0000000000001</ho:LOWER-LIMIT>\n                <ho:UPPER-LIMIT INTERVAL-TYPE=\"CLOSED\">500.0000000000001</ho:UPPER-LIMIT>\n              </ho:SCALE-CONSTR>\n            </ho:PHYS-CONSTRS>\n            <ho:COMPU-INTERNAL-TO-PHYS>\n              <ho:COMPU-SCALES>\n                <ho:COMPU-SCALE>\n                  <ho:COMPU-RATIONAL-COEFFS>\n                    <ho:COMPU-NUMERATOR>\n                      <ho:V>0</ho:V>\n                      <ho:V>1</ho:V>\n                    </ho:COMPU-NUMERATOR>\n                    <ho:COMPU-DENOMINATOR>\n                      <ho:V>1</ho:V>\n                    </ho:COMPU-DENOMINATOR>\n                  </ho:COMPU-RATIONAL-COEFFS>\n                </ho:COMPU-SCALE>\n              </ho:COMPU-SCALES>\n            </ho:COMPU-INTERNAL-TO-PHYS>\n          </ho:COMPU-METHOD>\n        </ho:COMPU-METHODS>\n      </fx:CODING>\n      <fx:CODING ID=\"cod64\">\n        <ho:SHORT-NAME>cod64</ho:SHORT-NAME>\n        <ho:CODED-TYPE ho:BASE-DATA-TYPE=\"A_UINT16\" CATEGORY=\"STANDARD-LENGTH-TYPE\" ENCODING=\"UNSIGNED\">\n          <ho:BIT-LENGTH>16</ho:BIT-LENGTH>\n        </ho:CODED-TYPE>\n        <ho:COMPU-METHODS>\n          <ho:COMPU-METHOD>\n            <ho:SHORT-NAME>cpm64</ho:SHORT-NAME>\n            <ho:CATEGORY>LINEAR</ho:CATEGORY>\n            <ho:UNIT-REF ID-REF=\"unit64\"/>\n            <ho:PHYS-CONSTRS>\n              <ho:SCALE-CONSTR>\n                <ho:LOWER-LIMIT INTERVAL-TYPE=\"CLOSED\">-500.0000000000001</ho:LOWER-LIMIT>\n                <ho:UPPER-LIMIT INTERVAL-TYPE=\"CLOSED\">500.0000000000001</ho:UPPER-LIMIT>\n              </ho:SCALE-CONSTR>\n            </ho:PHYS-CONSTRS>\n            <ho:COMPU-INTERNAL-TO-PHYS>\n              <ho:COMPU-SCALES>\n                <ho:COMPU-SCALE>\n                  <ho:COMPU-RATIONAL-COEFFS>\n                    <ho:COMPU-NUMERATOR>\n                      <ho:V>0</ho:V>\n                      <ho:V>1</ho:V>\n                    </ho:COMPU-NUMERATOR>\n                    <ho:COMPU-DENOMINATOR>\n                      <ho:V>1</ho:V>\n                    </ho:COMPU-DENOMINATOR>\n                  </ho:COMPU-RATIONAL-COEFFS>\n                </ho:COMPU-SCALE>\n              </ho:COMPU-SCALES>\n            </ho:COMPU-INTERNAL-TO-PHYS>\n          </ho:COMPU-METHOD>\n        </ho:COMPU-METHODS>\n      </fx:CODING>\n      <fx:CODING ID=\"cod65\">\n        <ho:SHORT-NAME>cod65</ho:SHORT-NAME>\n        <ho:CODED-TYPE ho:BASE-DATA-TYPE=\"A_UINT16\" CATEGORY=\"STANDARD-LENGTH-TYPE\" ENCODING=\"UNSIGNED\">\n          <ho:BIT-LENGTH>16</ho:BIT-LENGTH>\n        </ho:CODED-TYPE>\n        <ho:COMPU-METHODS>\n          <ho:COMPU-METHOD>\n            <ho:SHORT-NAME>cpm65</ho:SHORT-NAME>\n            <ho:CATEGORY>LINEAR</ho:CATEGORY>\n            <ho:UNIT-REF ID-REF=\"unit65\"/>\n            <ho:PHYS-CONSTRS>\n              <ho:SCALE-CONSTR>\n                <ho:LOWER-LIMIT INTERVAL-TYPE=\"CLOSED\">-500.0000000000001</ho:LOWER-LIMIT>\n                <ho:UPPER-LIMIT INTERVAL-TYPE=\"CLOSED\">500.0000000000001</ho:UPPER-LIMIT>\n              </ho:SCALE-CONSTR>\n            </ho:PHYS-CONSTRS>\n            <ho:COMPU-INTERNAL-TO-PHYS>\n              <ho:COMPU-SCALES>\n                <ho:COMPU-SCALE>\n                  <ho:COMPU-RATIONAL-COEFFS>\n                    <ho:COMPU-NUMERATOR>\n                      <ho:V>0</ho:V>\n                      <ho:V>1</ho:V>\n                    </ho:COMPU-NUMERATOR>\n                    <ho:COMPU-DENOMINATOR>\n                      <ho:V>1</ho:V>\n                    </ho:COMPU-DENOMINATOR>\n                  </ho:COMPU-RATIONAL-COEFFS>\n                </ho:COMPU-SCALE>\n              </ho:COMPU-SCALES>\n            </ho:COMPU-INTERNAL-TO-PHYS>\n          </ho:COMPU-METHOD>\n        </ho:COMPU-METHODS>\n      </fx:CODING>\n      <fx:CODING ID=\"cod66\">\n        <ho:SHORT-NAME>cod66</ho:SHORT-NAME>\n        <ho:CODED-TYPE ho:BASE-DATA-TYPE=\"A_UINT16\" CATEGORY=\"STANDARD-LENGTH-TYPE\" ENCODING=\"UNSIGNED\">\n          <ho:BIT-LENGTH>16</ho:BIT-LENGTH>\n        </ho:CODED-TYPE>\n        <ho:COMPU-METHODS>\n          <ho:COMPU-METHOD>\n            <ho:SHORT-NAME>cpm66</ho:SHORT-NAME>\n            <ho:CATEGORY>LINEAR</ho:CATEGORY>\n            <ho:UNIT-REF ID-REF=\"unit66\"/>\n            <ho:PHYS-CONSTRS>\n              <ho:SCALE-CONSTR>\n                <ho:LOWER-LIMIT INTERVAL-TYPE=\"CLOSED\">-500.0000000000001</ho:LOWER-LIMIT>\n                <ho:UPPER-LIMIT INTERVAL-TYPE=\"CLOSED\">500.0000000000001</ho:UPPER-LIMIT>\n              </ho:SCALE-CONSTR>\n            </ho:PHYS-CONSTRS>\n            <ho:COMPU-INTERNAL-TO-PHYS>\n              <ho:COMPU-SCALES>\n                <ho:COMPU-SCALE>\n                  <ho:COMPU-RATIONAL-COEFFS>\n                    <ho:COMPU-NUMERATOR>\n                      <ho:V>0</ho:V>\n                      <ho:V>1</ho:V>\n                    </ho:COMPU-NUMERATOR>\n                    <ho:COMPU-DENOMINATOR>\n                      <ho:V>1</ho:V>\n                    </ho:COMPU-DENOMINATOR>\n                  </ho:COMPU-RATIONAL-COEFFS>\n                </ho:COMPU-SCALE>\n              </ho:COMPU-SCALES>\n            </ho:COMPU-INTERNAL-TO-PHYS>\n          </ho:COMPU-METHOD>\n        </ho:COMPU-METHODS>\n      </fx:CODING>\n      <fx:CODING ID=\"cod67\">\n        <ho:SHORT-NAME>cod67</ho:SHORT-NAME>\n        <ho:CODED-TYPE ho:BASE-DATA-TYPE=\"A_UINT8\" CATEGORY=\"STANDARD-LENGTH-TYPE\" ENCODING=\"UNSIGNED\">\n          <ho:BIT-LENGTH>8</ho:BIT-LENGTH>\n        </ho:CODED-TYPE>\n        <ho:COMPU-METHODS>\n          <ho:COMPU-METHOD>\n            <ho:SHORT-NAME>cpm67</ho:SHORT-NAME>\n            <ho:CATEGORY>LINEAR</ho:CATEGORY>\n            <ho:UNIT-REF ID-REF=\"unit67\"/>\n            <ho:PHYS-CONSTRS>\n              <ho:SCALE-CONSTR>\n                <ho:LOWER-LIMIT INTERVAL-TYPE=\"CLOSED\">0</ho:LOWER-LIMIT>\n                <ho:UPPER-LIMIT INTERVAL-TYPE=\"CLOSED\">255</ho:UPPER-LIMIT>\n              </ho:SCALE-CONSTR>\n            </ho:PHYS-CONSTRS>\n            <ho:COMPU-INTERNAL-TO-PHYS>\n              <ho:COMPU-SCALES>\n                <ho:COMPU-SCALE>\n                  <ho:COMPU-RATIONAL-COEFFS>\n                    <ho:COMPU-NUMERATOR>\n                      <ho:V>0</ho:V>\n                      <ho:V>1</ho:V>\n                    </ho:COMPU-NUMERATOR>\n                    <ho:COMPU-DENOMINATOR>\n                      <ho:V>1</ho:V>\n                    </ho:COMPU-DENOMINATOR>\n                  </ho:COMPU-RATIONAL-COEFFS>\n                </ho:COMPU-SCALE>\n              </ho:COMPU-SCALES>\n            </ho:COMPU-INTERNAL-TO-PHYS>\n          </ho:COMPU-METHOD>\n        </ho:COMPU-METHODS>\n      </fx:CODING>\n      <fx:CODING ID=\"cod68\">\n        <ho:SHORT-NAME>cod68</ho:SHORT-NAME>\n        <ho:CODED-TYPE ho:BASE-DATA-TYPE=\"A_UINT16\" CATEGORY=\"STANDARD-LENGTH-TYPE\" ENCODING=\"UNSIGNED\">\n          <ho:BIT-LENGTH>16</ho:BIT-LENGTH>\n        </ho:CODED-TYPE>\n        <ho:COMPU-METHODS>\n          <ho:COMPU-METHOD>\n            <ho:SHORT-NAME>cpm68</ho:SHORT-NAME>\n            <ho:CATEGORY>LINEAR</ho:CATEGORY>\n            <ho:UNIT-REF ID-REF=\"unit68\"/>\n            <ho:PHYS-CONSTRS>\n              <ho:SCALE-CONSTR>\n                <ho:LOWER-LIMIT INTERVAL-TYPE=\"CLOSED\">0</ho:LOWER-LIMIT>\n                <ho:UPPER-LIMIT INTERVAL-TYPE=\"CLOSED\">5</ho:UPPER-LIMIT>\n              </ho:SCALE-CONSTR>\n            </ho:PHYS-CONSTRS>\n            <ho:COMPU-INTERNAL-TO-PHYS>\n              <ho:COMPU-SCALES>\n                <ho:COMPU-SCALE>\n                  <ho:COMPU-RATIONAL-COEFFS>\n                    <ho:COMPU-NUMERATOR>\n                      <ho:V>0</ho:V>\n                      <ho:V>1</ho:V>\n                    </ho:COMPU-NUMERATOR>\n                    <ho:COMPU-DENOMINATOR>\n                      <ho:V>1</ho:V>\n                    </ho:COMPU-DENOMINATOR>\n                  </ho:COMPU-RATIONAL-COEFFS>\n                </ho:COMPU-SCALE>\n              </ho:COMPU-SCALES>\n            </ho:COMPU-INTERNAL-TO-PHYS>\n          </ho:COMPU-METHOD>\n        </ho:COMPU-METHODS>\n      </fx:CODING>\n      <fx:CODING ID=\"cod69\">\n        <ho:SHORT-NAME>cod69</ho:SHORT-NAME>\n        <ho:CODED-TYPE ho:BASE-DATA-TYPE=\"A_UINT16\" CATEGORY=\"STANDARD-LENGTH-TYPE\" ENCODING=\"UNSIGNED\">\n          <ho:BIT-LENGTH>16</ho:BIT-LENGTH>\n        </ho:CODED-TYPE>\n        <ho:COMPU-METHODS>\n          <ho:COMPU-METHOD>\n            <ho:SHORT-NAME>cpm69</ho:SHORT-NAME>\n            <ho:CATEGORY>LINEAR</ho:CATEGORY>\n            <ho:UNIT-REF ID-REF=\"unit69\"/>\n            <ho:PHYS-CONSTRS>\n              <ho:SCALE-CONSTR>\n                <ho:LOWER-LIMIT INTERVAL-TYPE=\"CLOSED\">0</ho:LOWER-LIMIT>\n                <ho:UPPER-LIMIT INTERVAL-TYPE=\"CLOSED\">5</ho:UPPER-LIMIT>\n              </ho:SCALE-CONSTR>\n            </ho:PHYS-CONSTRS>\n            <ho:COMPU-INTERNAL-TO-PHYS>\n              <ho:COMPU-SCALES>\n                <ho:COMPU-SCALE>\n                  <ho:COMPU-RATIONAL-COEFFS>\n                    <ho:COMPU-NUMERATOR>\n                      <ho:V>0</ho:V>\n                      <ho:V>1</ho:V>\n                    </ho:COMPU-NUMERATOR>\n                    <ho:COMPU-DENOMINATOR>\n                      <ho:V>1</ho:V>\n                    </ho:COMPU-DENOMINATOR>\n                  </ho:COMPU-RATIONAL-COEFFS>\n                </ho:COMPU-SCALE>\n              </ho:COMPU-SCALES>\n            </ho:COMPU-INTERNAL-TO-PHYS>\n          </ho:COMPU-METHOD>\n        </ho:COMPU-METHODS>\n      </fx:CODING>\n      <fx:CODING ID=\"cod70\">\n        <ho:SHORT-NAME>cod70</ho:SHORT-NAME>\n        <ho:CODED-TYPE ho:BASE-DATA-TYPE=\"A_UINT16\" CATEGORY=\"STANDARD-LENGTH-TYPE\" ENCODING=\"UNSIGNED\">\n          <ho:BIT-LENGTH>16</ho:BIT-LENGTH>\n        </ho:CODED-TYPE>\n        <ho:COMPU-METHODS>\n          <ho:COMPU-METHOD>\n            <ho:SHORT-NAME>cpm70</ho:SHORT-NAME>\n            <ho:CATEGORY>LINEAR</ho:CATEGORY>\n            <ho:UNIT-REF ID-REF=\"unit70\"/>\n            <ho:PHYS-CONSTRS>\n              <ho:SCALE-CONSTR>\n                <ho:LOWER-LIMIT INTERVAL-TYPE=\"CLOSED\">0</ho:LOWER-LIMIT>\n                <ho:UPPER-LIMIT INTERVAL-TYPE=\"CLOSED\">5</ho:UPPER-LIMIT>\n              </ho:SCALE-CONSTR>\n            </ho:PHYS-CONSTRS>\n            <ho:COMPU-INTERNAL-TO-PHYS>\n              <ho:COMPU-SCALES>\n                <ho:COMPU-SCALE>\n                  <ho:COMPU-RATIONAL-COEFFS>\n                    <ho:COMPU-NUMERATOR>\n                      <ho:V>0</ho:V>\n                      <ho:V>1</ho:V>\n                    </ho:COMPU-NUMERATOR>\n                    <ho:COMPU-DENOMINATOR>\n                      <ho:V>1</ho:V>\n                    </ho:COMPU-DENOMINATOR>\n                  </ho:COMPU-RATIONAL-COEFFS>\n                </ho:COMPU-SCALE>\n              </ho:COMPU-SCALES>\n            </ho:COMPU-INTERNAL-TO-PHYS>\n          </ho:COMPU-METHOD>\n        </ho:COMPU-METHODS>\n      </fx:CODING>\n      <fx:CODING ID=\"cod71\">\n        <ho:SHORT-NAME>cod71</ho:SHORT-NAME>\n        <ho:CODED-TYPE ho:BASE-DATA-TYPE=\"A_UINT16\" CATEGORY=\"STANDARD-LENGTH-TYPE\" ENCODING=\"UNSIGNED\">\n          <ho:BIT-LENGTH>16</ho:BIT-LENGTH>\n        </ho:CODED-TYPE>\n        <ho:COMPU-METHODS>\n          <ho:COMPU-METHOD>\n            <ho:SHORT-NAME>cpm71</ho:SHORT-NAME>\n            <ho:CATEGORY>LINEAR</ho:CATEGORY>\n            <ho:UNIT-REF ID-REF=\"unit71\"/>\n            <ho:PHYS-CONSTRS>\n              <ho:SCALE-CONSTR>\n                <ho:LOWER-LIMIT INTERVAL-TYPE=\"CLOSED\">0</ho:LOWER-LIMIT>\n                <ho:UPPER-LIMIT INTERVAL-TYPE=\"CLOSED\">5</ho:UPPER-LIMIT>\n              </ho:SCALE-CONSTR>\n            </ho:PHYS-CONSTRS>\n            <ho:COMPU-INTERNAL-TO-PHYS>\n              <ho:COMPU-SCALES>\n                <ho:COMPU-SCALE>\n                  <ho:COMPU-RATIONAL-COEFFS>\n                    <ho:COMPU-NUMERATOR>\n                      <ho:V>0</ho:V>\n                      <ho:V>1</ho:V>\n                    </ho:COMPU-NUMERATOR>\n                    <ho:COMPU-DENOMINATOR>\n                      <ho:V>1</ho:V>\n                    </ho:COMPU-DENOMINATOR>\n                  </ho:COMPU-RATIONAL-COEFFS>\n                </ho:COMPU-SCALE>\n              </ho:COMPU-SCALES>\n            </ho:COMPU-INTERNAL-TO-PHYS>\n          </ho:COMPU-METHOD>\n        </ho:COMPU-METHODS>\n      </fx:CODING>\n      <fx:CODING ID=\"cod72\">\n        <ho:SHORT-NAME>cod72</ho:SHORT-NAME>\n        <ho:CODED-TYPE ho:BASE-DATA-TYPE=\"A_UINT16\" CATEGORY=\"STANDARD-LENGTH-TYPE\" ENCODING=\"UNSIGNED\">\n          <ho:BIT-LENGTH>16</ho:BIT-LENGTH>\n        </ho:CODED-TYPE>\n        <ho:COMPU-METHODS>\n          <ho:COMPU-METHOD>\n            <ho:SHORT-NAME>cpm72</ho:SHORT-NAME>\n            <ho:CATEGORY>LINEAR</ho:CATEGORY>\n            <ho:UNIT-REF ID-REF=\"unit72\"/>\n            <ho:PHYS-CONSTRS>\n              <ho:SCALE-CONSTR>\n                <ho:LOWER-LIMIT INTERVAL-TYPE=\"CLOSED\">0</ho:LOWER-LIMIT>\n                <ho:UPPER-LIMIT INTERVAL-TYPE=\"CLOSED\">1000</ho:UPPER-LIMIT>\n              </ho:SCALE-CONSTR>\n            </ho:PHYS-CONSTRS>\n            <ho:COMPU-INTERNAL-TO-PHYS>\n              <ho:COMPU-SCALES>\n                <ho:COMPU-SCALE>\n                  <ho:COMPU-RATIONAL-COEFFS>\n                    <ho:COMPU-NUMERATOR>\n                      <ho:V>0</ho:V>\n                      <ho:V>1</ho:V>\n                    </ho:COMPU-NUMERATOR>\n                    <ho:COMPU-DENOMINATOR>\n                      <ho:V>1</ho:V>\n                    </ho:COMPU-DENOMINATOR>\n                  </ho:COMPU-RATIONAL-COEFFS>\n                </ho:COMPU-SCALE>\n              </ho:COMPU-SCALES>\n            </ho:COMPU-INTERNAL-TO-PHYS>\n          </ho:COMPU-METHOD>\n        </ho:COMPU-METHODS>\n      </fx:CODING>\n      <fx:CODING ID=\"cod73\">\n        <ho:SHORT-NAME>cod73</ho:SHORT-NAME>\n        <ho:CODED-TYPE ho:BASE-DATA-TYPE=\"A_UINT16\" CATEGORY=\"STANDARD-LENGTH-TYPE\" ENCODING=\"UNSIGNED\">\n          <ho:BIT-LENGTH>16</ho:BIT-LENGTH>\n        </ho:CODED-TYPE>\n        <ho:COMPU-METHODS>\n          <ho:COMPU-METHOD>\n            <ho:SHORT-NAME>cpm73</ho:SHORT-NAME>\n            <ho:CATEGORY>LINEAR</ho:CATEGORY>\n            <ho:UNIT-REF ID-REF=\"unit73\"/>\n            <ho:PHYS-CONSTRS>\n              <ho:SCALE-CONSTR>\n                <ho:LOWER-LIMIT INTERVAL-TYPE=\"CLOSED\">0</ho:LOWER-LIMIT>\n                <ho:UPPER-LIMIT INTERVAL-TYPE=\"CLOSED\">5</ho:UPPER-LIMIT>\n              </ho:SCALE-CONSTR>\n            </ho:PHYS-CONSTRS>\n            <ho:COMPU-INTERNAL-TO-PHYS>\n              <ho:COMPU-SCALES>\n                <ho:COMPU-SCALE>\n                  <ho:COMPU-RATIONAL-COEFFS>\n                    <ho:COMPU-NUMERATOR>\n                      <ho:V>0</ho:V>\n                      <ho:V>1</ho:V>\n                    </ho:COMPU-NUMERATOR>\n                    <ho:COMPU-DENOMINATOR>\n                      <ho:V>1</ho:V>\n                    </ho:COMPU-DENOMINATOR>\n                  </ho:COMPU-RATIONAL-COEFFS>\n                </ho:COMPU-SCALE>\n              </ho:COMPU-SCALES>\n            </ho:COMPU-INTERNAL-TO-PHYS>\n          </ho:COMPU-METHOD>\n        </ho:COMPU-METHODS>\n      </fx:CODING>\n      <fx:CODING ID=\"cod74\">\n        <ho:SHORT-NAME>cod74</ho:SHORT-NAME>\n        <ho:CODED-TYPE ho:BASE-DATA-TYPE=\"A_UINT16\" CATEGORY=\"STANDARD-LENGTH-TYPE\" ENCODING=\"UNSIGNED\">\n          <ho:BIT-LENGTH>16</ho:BIT-LENGTH>\n        </ho:CODED-TYPE>\n        <ho:COMPU-METHODS>\n          <ho:COMPU-METHOD>\n            <ho:SHORT-NAME>cpm74</ho:SHORT-NAME>\n            <ho:CATEGORY>LINEAR</ho:CATEGORY>\n            <ho:UNIT-REF ID-REF=\"unit74\"/>\n            <ho:PHYS-CONSTRS>\n              <ho:SCALE-CONSTR>\n                <ho:LOWER-LIMIT INTERVAL-TYPE=\"CLOSED\">0</ho:LOWER-LIMIT>\n                <ho:UPPER-LIMIT INTERVAL-TYPE=\"CLOSED\">5</ho:UPPER-LIMIT>\n              </ho:SCALE-CONSTR>\n            </ho:PHYS-CONSTRS>\n            <ho:COMPU-INTERNAL-TO-PHYS>\n              <ho:COMPU-SCALES>\n                <ho:COMPU-SCALE>\n                  <ho:COMPU-RATIONAL-COEFFS>\n                    <ho:COMPU-NUMERATOR>\n                      <ho:V>0</ho:V>\n                      <ho:V>1</ho:V>\n                    </ho:COMPU-NUMERATOR>\n                    <ho:COMPU-DENOMINATOR>\n                      <ho:V>1</ho:V>\n                    </ho:COMPU-DENOMINATOR>\n                  </ho:COMPU-RATIONAL-COEFFS>\n                </ho:COMPU-SCALE>\n              </ho:COMPU-SCALES>\n            </ho:COMPU-INTERNAL-TO-PHYS>\n          </ho:COMPU-METHOD>\n        </ho:COMPU-METHODS>\n      </fx:CODING>\n      <fx:CODING ID=\"cod75\">\n        <ho:SHORT-NAME>cod75</ho:SHORT-NAME>\n        <ho:CODED-TYPE ho:BASE-DATA-TYPE=\"A_UINT16\" CATEGORY=\"STANDARD-LENGTH-TYPE\" ENCODING=\"UNSIGNED\">\n          <ho:BIT-LENGTH>16</ho:BIT-LENGTH>\n        </ho:CODED-TYPE>\n        <ho:COMPU-METHODS>\n          <ho:COMPU-METHOD>\n            <ho:SHORT-NAME>cpm75</ho:SHORT-NAME>\n            <ho:CATEGORY>LINEAR</ho:CATEGORY>\n            <ho:UNIT-REF ID-REF=\"unit75\"/>\n            <ho:PHYS-CONSTRS>\n              <ho:SCALE-CONSTR>\n                <ho:LOWER-LIMIT INTERVAL-TYPE=\"CLOSED\">0</ho:LOWER-LIMIT>\n                <ho:UPPER-LIMIT INTERVAL-TYPE=\"CLOSED\">5</ho:UPPER-LIMIT>\n              </ho:SCALE-CONSTR>\n            </ho:PHYS-CONSTRS>\n            <ho:COMPU-INTERNAL-TO-PHYS>\n              <ho:COMPU-SCALES>\n                <ho:COMPU-SCALE>\n                  <ho:COMPU-RATIONAL-COEFFS>\n                    <ho:COMPU-NUMERATOR>\n                      <ho:V>0</ho:V>\n                      <ho:V>1</ho:V>\n                    </ho:COMPU-NUMERATOR>\n                    <ho:COMPU-DENOMINATOR>\n                      <ho:V>1</ho:V>\n                    </ho:COMPU-DENOMINATOR>\n                  </ho:COMPU-RATIONAL-COEFFS>\n                </ho:COMPU-SCALE>\n              </ho:COMPU-SCALES>\n            </ho:COMPU-INTERNAL-TO-PHYS>\n          </ho:COMPU-METHOD>\n        </ho:COMPU-METHODS>\n      </fx:CODING>\n    </fx:CODINGS>\n  </fx:PROCESSING-INFORMATION>\n</fx:FIBEX>\n")   [LabVIEW 2021, in "BS120x Driver.lvlib" / "BS120x.lvclass"]
uses:
  BS120x.lvclass
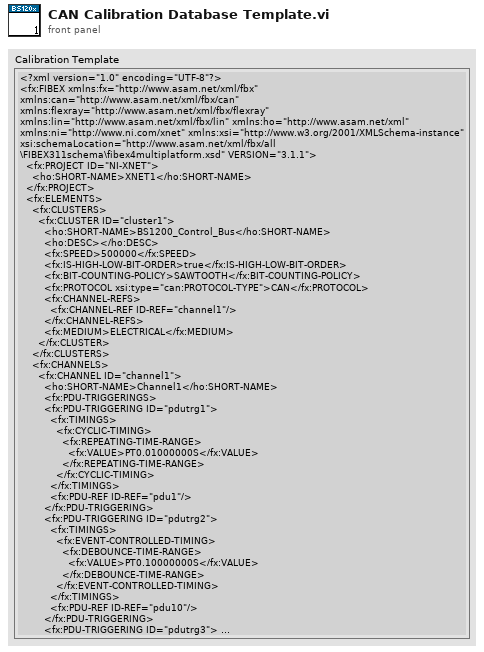
[diagram p1: front panel]
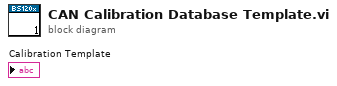
[diagram p0: block diagram]
diagram:
